vi "Omniax_MotorDrive_XYZR_SUPER.vi"() -> ()   [LabVIEW 2009]
uses:
  <vilib>/Utility/file.llb/Read From Spreadsheet File (DBL).vi
  <vilib>/Utility/file.llb/Read From Spreadsheet File (string).vi
  <vilib>/Instr/_visa.llb/VISA Configure Serial Port (Instr).vi
  <vilib>/Utility/file.llb/Write To Spreadsheet File (string).vi
  <vilib>/Utility/file.llb/Write To Spreadsheet File (DBL).vi
panel:
  out "OP":bool
  out "CL":bool
  out "Valve \nopend/closed":bool
  in  "OK Button":bool
  out "STATUS":string
  in  "Delete Button":bool
  in  "String":string
  in  "Add Button":bool
  in  "Set Button":bool
  in  "Preset positions":i32(ring) items=["ZERO", "Default", "CDOSE", "QMS", "test", "test2", "test3"]
  out "Presets":i32[][](array[numeric])
  out "X MINPOS":i32=-94296
  out "X MAXPOS":i32=-34296
  out "Y MINPOS":i32=-94296
  out "Y MAXPOS":i32=-34296
  out "R MAXPOS":i32=-34296
  out "R MINPOS":i32=-94296
  out "Z MINPOS":i32=-94296
  out "Z MAXPOS":i32=-34296
  in  "HARDSTOP":bool
  in  "GO":bool
  out "XYZR VEL PV Array":i32[](array[numeric])
  out "XYZ in RANGE Array":bool[](array[boolean])
  out "STEP SP Array":i32[](array[numeric])
  out "RUNHOLDArray":i32[](array[numeric])
  out "ZCONSTArray":dbl[](array[numeric])
  out "RCONSTArray":dbl[](array[numeric])
  out "XCONSTArray":dbl[](array[numeric])
  out "YCONSTArray":dbl[](array[numeric])
  out "Error Array":errorcluster[](array[cluster])
  out "COM PORT Array":refnum<visa-resource-name>[](array[refnum])
  out "Z COM PORT":refnum<visa-resource-name>="COM6"
  in  "Tab Control 3":enum32{"Status", "Reset"}(tab)
  out "Y in Range":bool
  out "Y Scan":bool
  out "Y in Motion":bool
  out "Y Backlash corr":bool
  out "X  in Range":bool
  out "X Scan":bool
  out "X  in Motion":bool
  out "X Backlash corr":bool
  out "Z in Range":bool
  out "Z Scan":bool
  out "Z in Motion":bool
  out "Z Backlash corr":bool
  out "R in Range":bool
  out "R Scan":bool
  out "R in Motion":bool
  out "R Backlash corr":bool
  out "X Ready":bool
  out "Y Ready":bool
  out "Z Ready":bool
  out "R Ready":bool
  in  "Reset Y Position mm":dbl
  out "Reset Y Motor Steps":i32
  in  "Reset X Position mm":dbl
  out "Reset X Motor Steps":i32
  in  "Reset Z Position mm":dbl
  out "Reset Z Motor Steps":i32
  in  "Reset R Position deg":dbl
  out "Reset R Motor Steps":i32
  in  "Reset":bool
  in  "Tab Control 2":enum32{"mm", "step"}(tab)
  in  "X Scan Length SP mm":dbl
  in  "X Scan Velocity SP mm/sec":dbl
  in  "Y Scan Length SP mm":dbl
  in  "Y Scan Velocity SP mm/sec":dbl
  in  "Set Scan \nParameters":bool
  in  "Z Scan Length SP mm":dbl
  in  "Z Scan Velocity SP mm/sec":dbl
  in  "R Scan Length SP deg":dbl
  in  "R Scan Velocity SP deg/sec":dbl
  in  "Z as dominating length":bool
  in  "X Scan Velocity SP steps/sec":i32=1 min=1 max=102400 step=1
  in  "X Scan Length SP steps":i32 min=-3507200 max=1100800 step=100
  out "X Scan length MV mm":dbl
  out "X Scan velocity MV mm/sec":dbl format="%#_6f"
  in  "Y Scan Velocity SP steps/sec":i32=1 min=1 max=102400 step=1
  in  "Y Scan Length SP steps":i32 min=-2562560 max=2045440 step=100
  out "Y Scan length MV mm":dbl
  out "Y Scan velocity MV mm/sec":dbl format="%#_6f"
  in  "Z Scan Velocity SP steps/sec":i32=1 min=1 max=102400 step=1
  in  "Z Scan Length SP steps":i32 min=-91443200 max=10956800 step=100
  out "Z Scan length MV mm":dbl
  out "Z Scan velocity MV mm/sec":dbl format="%#_6f"
  in  "R Scan Velocity SP steps/sec":i32=1 min=1 max=102400 step=1
  in  "R Scan Length SP steps":i32 min=-1501867 max=4642133 step=100
  out "R Scan length MV deg":dbl
  out "R Scan velocity MV deg/sec":dbl format="%#_6f"
  out "atan Y/Z":dbl
  in  "Tab Control":enum32{"mm", "step"}(tab)
  in  "X Position SP mm":dbl
  in  "X Velocity SP mm/sec":dbl
  in  "X Move Set":bool
  in  "Y Move Set":bool
  in  "Y Position SP mm":dbl
  in  "Y Velocity SP mm/sec":dbl
  in  "Z Position SP mm":dbl
  in  "Z Velocity SP mm/sec":dbl
  in  "Z Move Set":bool
  in  "R Position SP deg":dbl
  in  "R Velocity SP deg/sec":dbl
  in  "R Move Set":bool
  in  "X Velocity SP step/sec":i32 min=1 max=128000
  out "X Velocity MV mm/sec":dbl
  in  "Y Velocity SP step/sec":i32 min=1 max=128000
  out "Y Velocity MV mm/sec":dbl
  in  "Z Velocity SP step/sec":i32 min=1 max=204800
  out "Z Velocity MV mm/sec":dbl
  in  "R Velocity SP step/sec":i32 min=1 max=20000
  out "R Velocity MVdeg/sec":dbl
  in  "Y Step SP":i32=-20000 min=-2304000 max=2304000 step=500
  out "Y Position MV mm":dbl
  in  "X Step SP":i32=-20000 min=-2304000 max=2304000 step=500
  out "X Position MV mm":dbl
  in  "Z Step SP":i32=-20000 min=0 max=102400000 step=500
  out "Z Position MV mm":dbl
  in  "R Step SP":i32=-20000 min=-6144000 max=0 step=500
  out "R Position MV deg":dbl
  out "X Step PV":i32 max=2000
  out "Y Step PV":i32 max=2000
  out "Z Step PV":i32 max=2000
  out "R Step PV":i32 max=2000
  in  "Clear ZY":bool
  out "ZY Graph":cluster{dbl[], dbl[]}(graph)
  out "ZR Graph":cluster{"Y":dbl[], "Y":dbl[]}[](graph)
  out "XY Graph":cluster{"Y":dbl[], "Y":dbl[]}[](graph)
  out "X Scan Duration":dbl
  out "Y Scan Duration":dbl
  out "Z Scan Duration":dbl
  out "R Scan Duration":dbl
  out "R Backlash steps/sec":i32
  out "R Backlash":i32
  out "R Holding Current %":i32
  out "R Run Current %":i32
  out "R offset deg":dbl
  out "R deg/rev":dbl
  out "R steps/rev":u32
  out "R velocity PV step/sec":i32
  out "R COM PORT":refnum<visa-resource-name>="COM5"
  out "R Position deg PV":dbl
  out "Z Backlash steps/sec":i32
  out "Z Backlash":i32
  out "Z Holding Current %":i32
  out "Z Run Current %":i32
  out "Z offset mm":dbl
  out "Z mm/rev":dbl
  out "Z steps/rev":u32
  out "Z  velocity PV step/sec":i32
  out "Z Position mm PV":dbl
  out "X Position mm PV":dbl
  out "X velocity PV step/sec":i32
  in  "Set for Scan":bool
  out "X Backlash steps/sec":i32
  out "X Backlash":i32
  out "X Holding Current %":i32
  out "X Run Current %":i32
  out "X offset mm":dbl
  out "X mm/rev":dbl
  out "X steps/rev":u32
  out "X COM PORT":refnum<visa-resource-name>="COM5"
  out "Y Backlash steps/sec":i32
  out "Y Backlash":i32
  out "Y Holding Current %":i32
  out "Y Run Current %":i32
  in  "Scan Cancel":bool
  out "Y Position mm PV":dbl
  out "Y offset mm":dbl
  out "Y mm/rev":dbl
  out "Y steps/rev":u32
  out "Y velocity PV step/sec":i32
  in  "Scan Go":bool
  in  "Stop":bool
  out "Y COM PORT":refnum<visa-resource-name>="COM5"
  # "MX"
  # "MY"
  # "MZ"
  # "MR"
  # "Indicators"
  # "L"
  # "M"
  # "B"
  # "S"
  # "R"
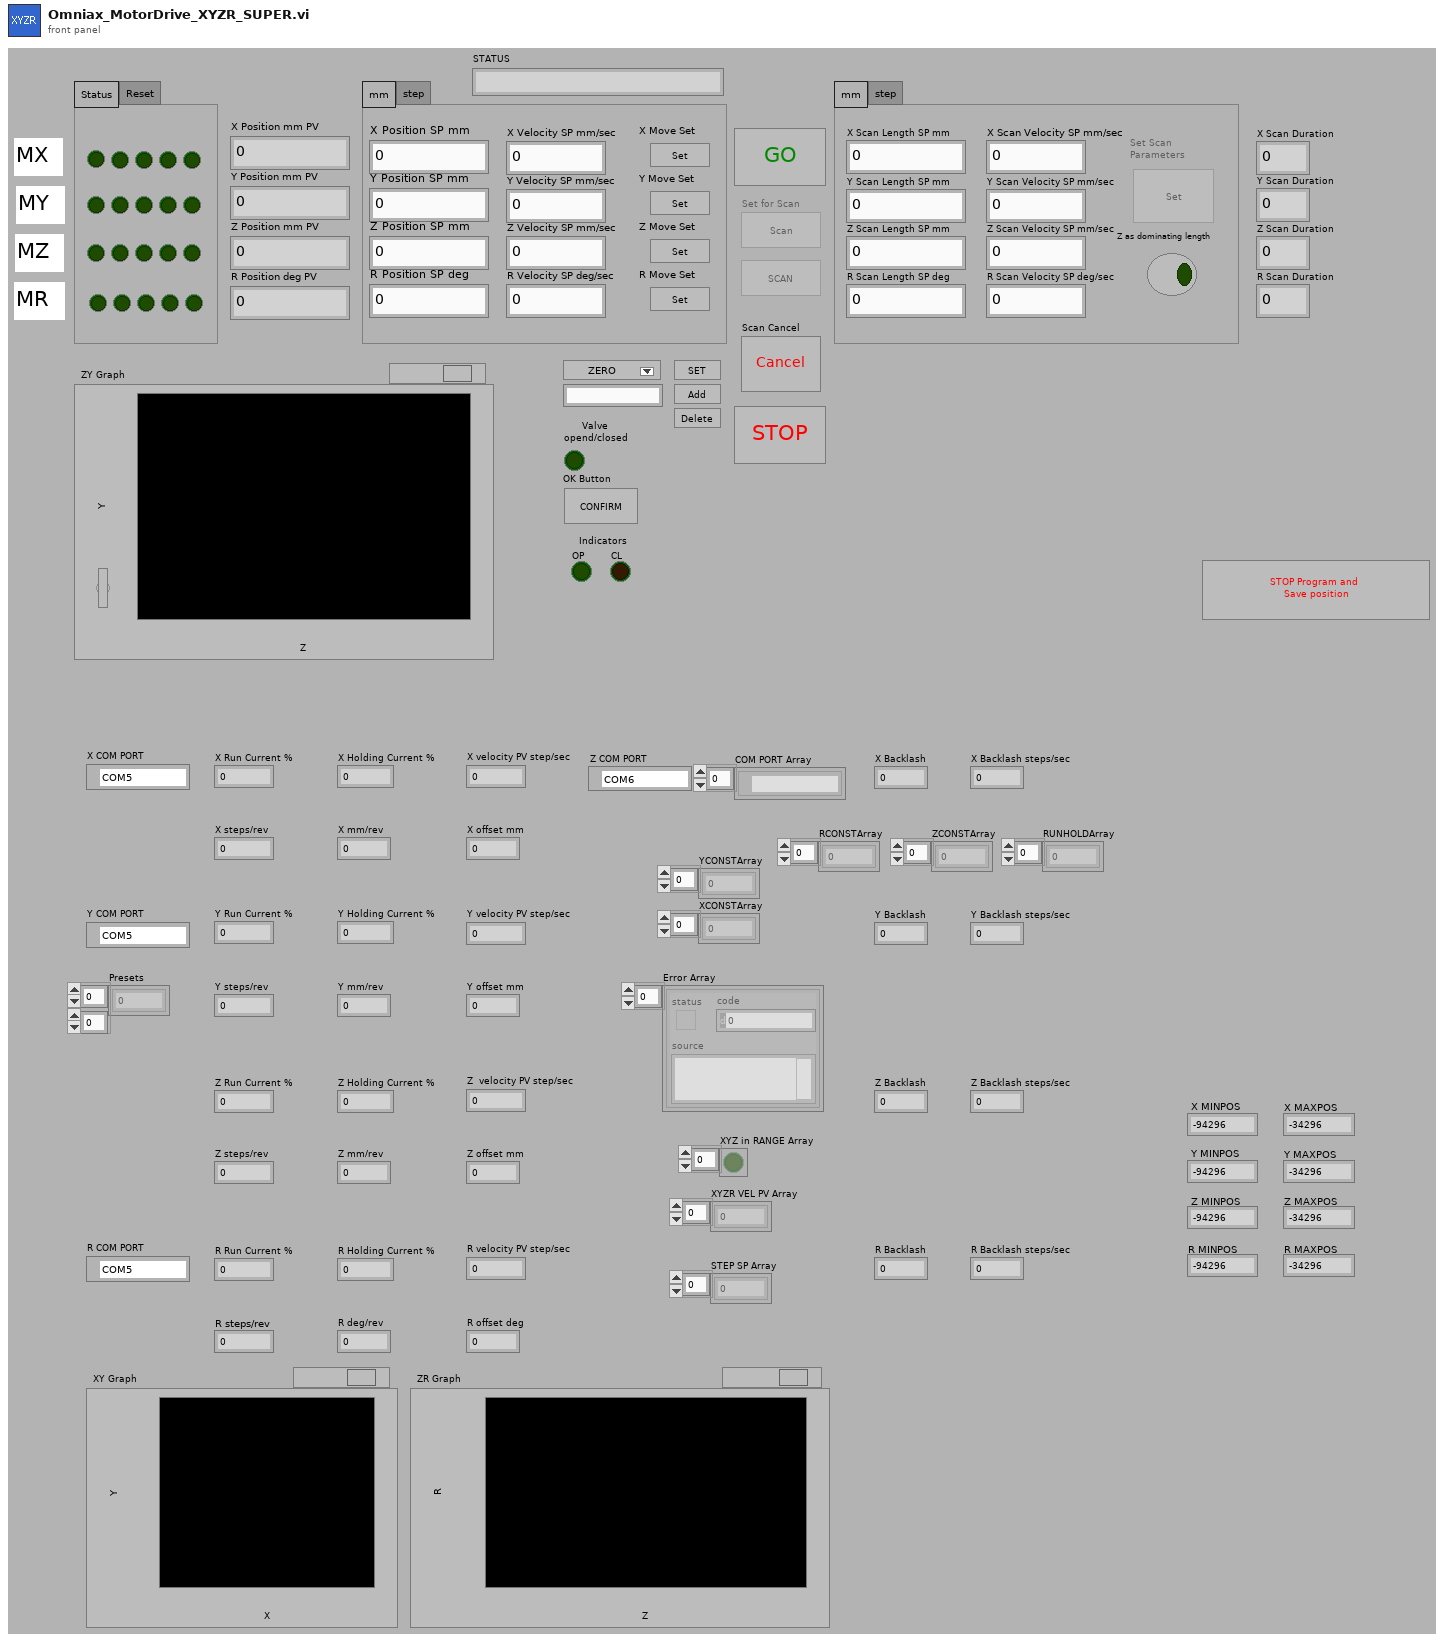
[diagram p1: front panel]
types:
  T1 = enum8{"Enabled", "Disabled", "Disabled and Grayed Out"}
  T2 = cluster{"[0]":i32, "[1]":i32, "[2]":i32, "[3]":i32, "[4]":i32, "[5]":i32, "[6]":i32, "[7]":i32, "[8]":i32}
  T3 = cluster{"XY Max Min array OUT[0]":dbl, "XY Max Min array OUT[1]":dbl, "XY Max Min array OUT[2]":dbl, "XY Max Min array OUT[3]":dbl, "XY Max Min array OUT[4]":dbl, "XY Max Min array OUT[5]":dbl, "XY Max Min array OUT[6]":dbl, "XY Max Min array OUT[7]":dbl, "XY Max Min array OUT[8]":dbl}
  T4 = cluster{"COM PORT Array OUT[0]":refnum<visa-resource-name>, "COM PORT Array OUT[1]":refnum<visa-resource-name>, "COM PORT Array OUT[2]":refnum<visa-resource-name>, "COM PORT Array OUT[3]":refnum<visa-resource-name>, "COM PORT Array OUT[4]":refnum<visa-resource-name>, "COM PORT Array OUT[5]":refnum<visa-resource-name>, "COM PORT Array OUT[6]":refnum<visa-resource-name>, "COM PORT Array OUT[7]":refnum<visa-resource-name>, "COM PORT Array OUT[8]":refnum<visa-resource-name>}
  T5 = cluster{"STEP SP Array OUT[0]":i32, "STEP SP Array OUT[1]":i32, "STEP SP Array OUT[2]":i32, "STEP SP Array OUT[3]":i32, "STEP SP Array OUT[4]":i32, "STEP SP Array OUT[5]":i32, "STEP SP Array OUT[6]":i32, "STEP SP Array OUT[7]":i32, "STEP SP Array OUT[8]":i32}
  T6 = cluster{"XYZ in RANGE Array OUT[0]":bool, "XYZ in RANGE Array OUT[1]":bool, "XYZ in RANGE Array OUT[2]":bool, "XYZ in RANGE Array OUT[3]":bool, "XYZ in RANGE Array OUT[4]":bool, "XYZ in RANGE Array OUT[5]":bool, "XYZ in RANGE Array OUT[6]":bool, "XYZ in RANGE Array OUT[7]":bool, "XYZ in RANGE Array OUT[8]":bool}
  T7 = cluster{"XYZR VEL PV Array OUT[0]":i32, "XYZR VEL PV Array OUT[1]":i32, "XYZR VEL PV Array OUT[2]":i32, "XYZR VEL PV Array OUT[3]":i32, "XYZR VEL PV Array OUT[4]":i32, "XYZR VEL PV Array OUT[5]":i32, "XYZR VEL PV Array OUT[6]":i32, "XYZR VEL PV Array OUT[7]":i32, "XYZR VEL PV Array OUT[8]":i32}
  T8 = cluster{"XYZR MAX MIN POS[0]":i32, "XYZR MAX MIN POS[1]":i32, "XYZR MAX MIN POS[2]":i32, "XYZR MAX MIN POS[3]":i32, "XYZR MAX MIN POS[4]":i32, "XYZR MAX MIN POS[5]":i32, "XYZR MAX MIN POS[6]":i32, "XYZR MAX MIN POS[7]":i32, "XYZR MAX MIN POS[8]":i32}
  T9 = cluster{"Error Array OUT[0]":errorcluster, "Error Array OUT[1]":errorcluster, "Error Array OUT[2]":errorcluster, "Error Array OUT[3]":errorcluster, "Error Array OUT[4]":errorcluster, "Error Array OUT[5]":errorcluster, "Error Array OUT[6]":errorcluster, "Error Array OUT[7]":errorcluster, "Error Array OUT[8]":errorcluster}
  T10 = enum16{"Stop", "Reset", "Run Current", "Holding Current", "Accel Rate", "Decel Rate", "Move to Relative Position", "Move to Absolute Position", "Echo Mode", "Print Parameter", "Send String", "Microstep Resolution", "Set Current Position", "Max Velocity"}
  T11 = cluster{"Presets[0]":i32, "Presets[1]":i32, "Presets[2]":i32, "Presets[3]":i32, "Presets[4]":i32, "Presets[5]":i32, "Presets[6]":i32, "Presets[7]":i32, "Presets[8]":i32}
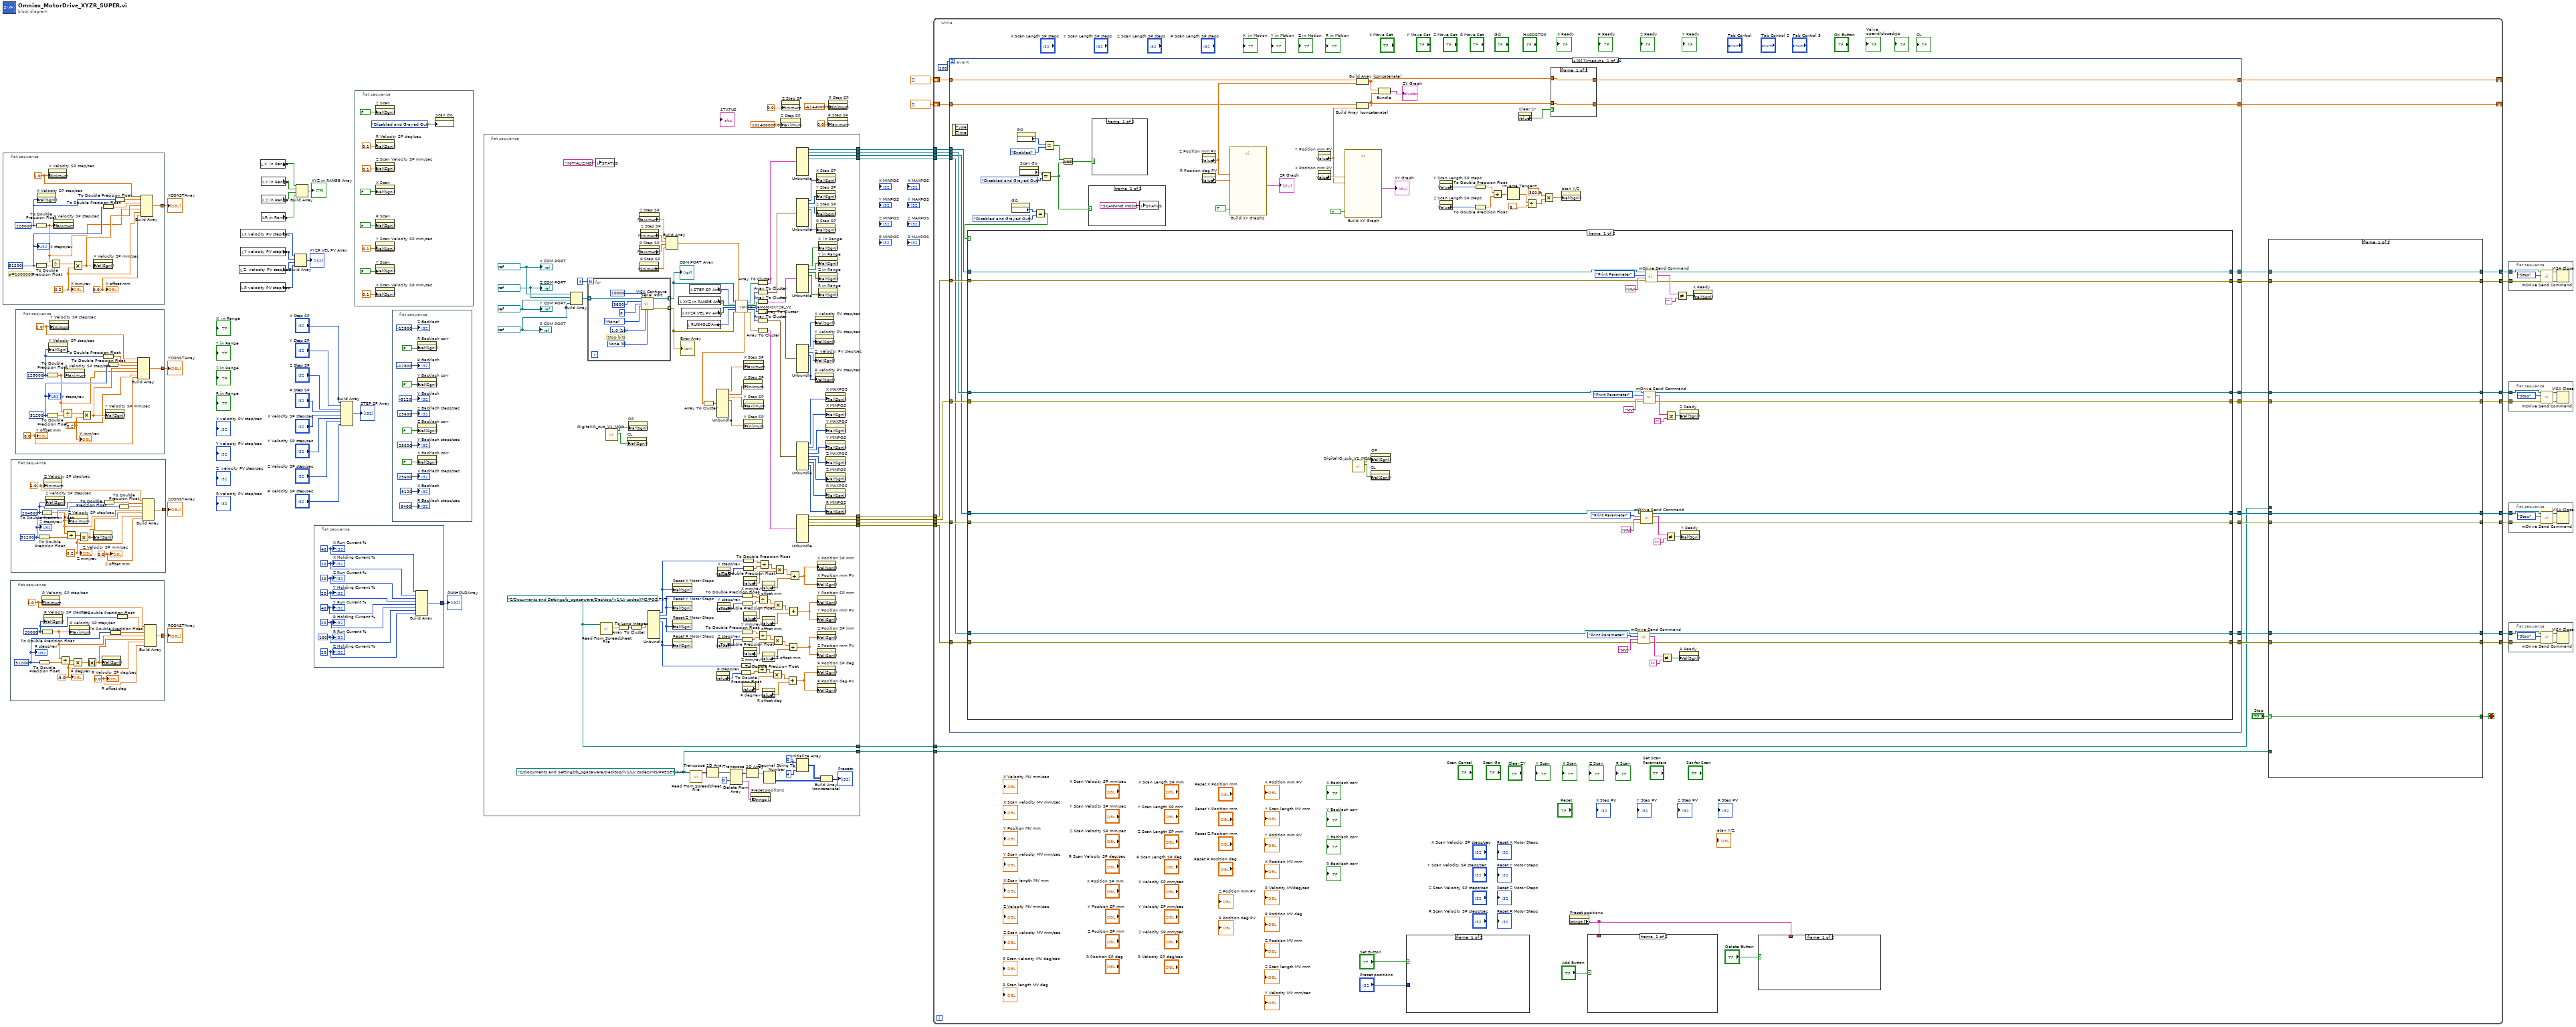
[diagram p0: block diagram]
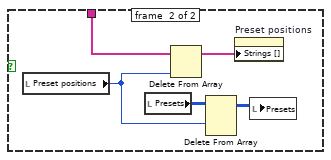
[diagram p2: hidden frame]
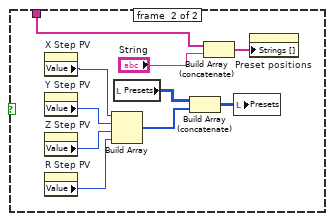
[diagram p3: hidden frame]
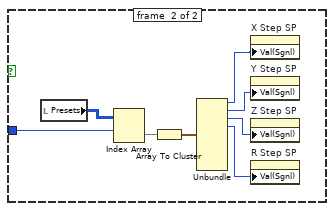
[diagram p4: hidden frame]
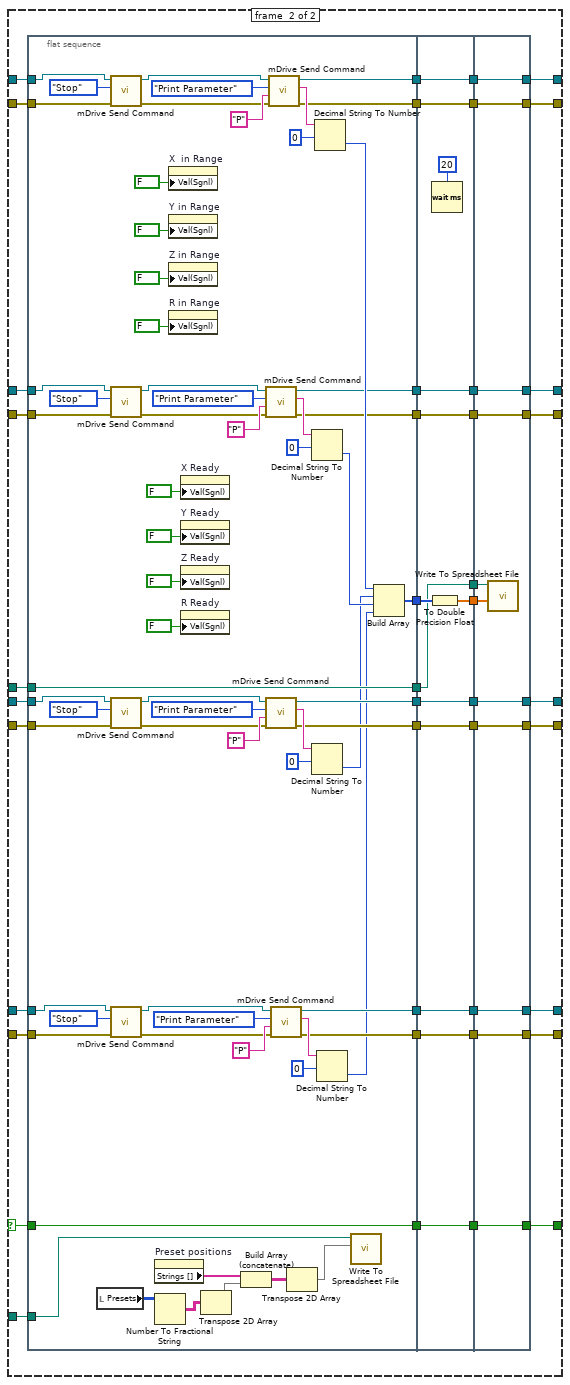
[diagram p5: hidden frame]
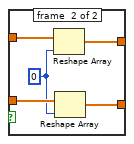
[diagram p6: hidden frame]
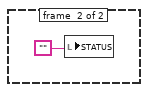
[diagram p8: hidden frame]
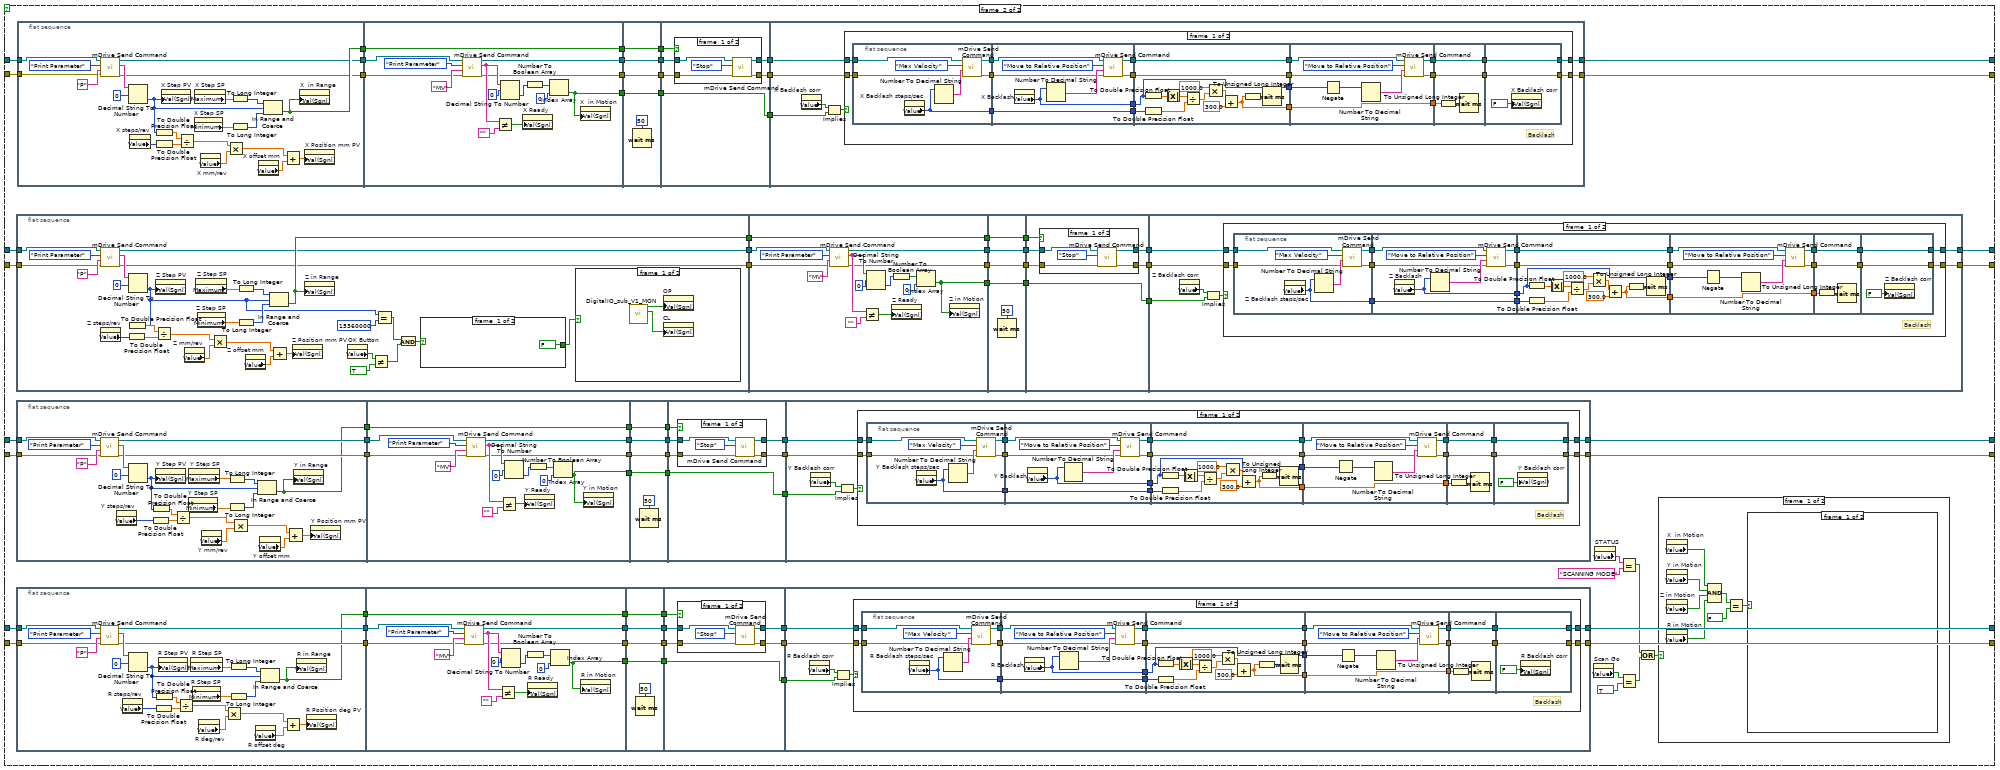
[diagram p9: hidden frame]
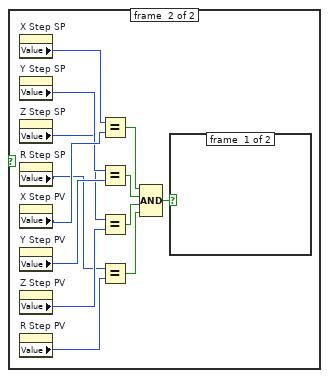
[diagram p10: hidden frame]
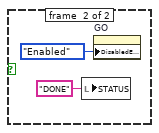
[diagram p11: hidden frame]
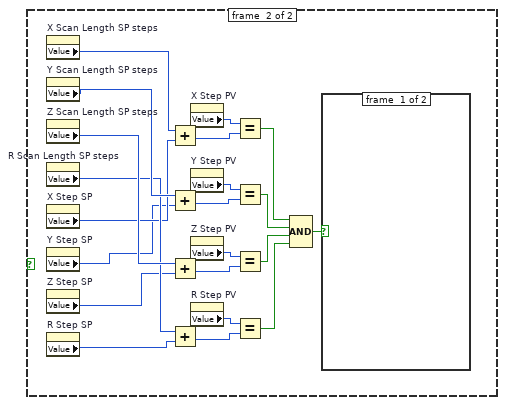
[diagram p12: hidden frame]
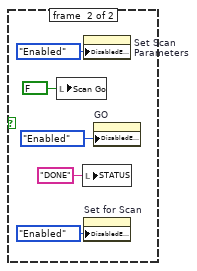
[diagram p13: hidden frame]
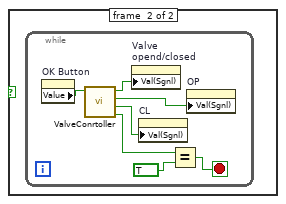
[diagram p18: hidden frame]
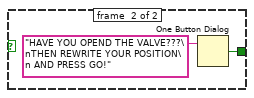
[diagram p19: hidden frame]
diagram:
  n1 = flat-sequence {
    tunnel: [w52] -> w35
    frame #0 {
      w50 = 0.2 ("MM/rev")
      w55 = u32 51200 ("step/rev")
      w57 = 128000 ("Value (Signaling)")
      w58 = 1.0 ("Data Entry Limits:Minimum")
      w51 = 0.0 ("offset")
      # "a=1000000"
      n2 = To Double Precision Float(number=w57) -> (double precision float=w49:dbl)
      n3 = To Double Precision Float(number=w55) -> (double precision float=w60:dbl)
      n4 = property on="X Velocity SP step/sec" class="DigNum (strict)"("Val(Sgnl)"=w57) -> ()  [unwired: 2 in, 2 out]
      n5 = property on="X Velocity SP step/sec" class="DigNum (strict)"("Minimum"=w58) -> ()  [unwired: 2 in, 2 out]
      n6 = Divide(x=w49, y=w60) -> (x/y=w59:dbl)
      n7 = property on="X Velocity SP step/sec" class="DigNum (strict)"("Maximum"=w49) -> ()  [unwired: 2 in, 2 out]
      n8 = Multiply(x=w59, y=w50) -> (x*y=w53:dbl)
      n9 = property on="X Velocity SP mm/sec" class="DigNum (strict)"("Val(Sgnl)"=w53) -> ()  [unwired: 2 in, 2 out]
      n10 = To Double Precision Float(number=w55) -> (double precision float=w54:dbl)
      n11 = To Double Precision Float(number=w57) -> (double precision float=w56:dbl)
      n12 = Build Array(w58, w56, w54, w53, w49, w50, w51) -> (w52:dbl[])
      "X offset mm" <- w51
      "X steps/rev" <- w55
      "X mm/rev" <- w50
    }
  }
  n13 = flat-sequence {
    tunnel: [w61] -> w34
    frame #0 {
      w70 = 1.0 ("Data Entry Limits:Minimum")
      w64 = 0.0 ("R offset deg")
      w65 = -3.0 ("R deg/rev")
      w68 = u32 51200 ("step/rev")
      w69 = 20000 ("Value (Signaling)")
      n14 = To Double Precision Float(number=w68) -> (double precision float=w71:dbl)
      n15 = To Double Precision Float(number=w69) -> (double precision float=w67:dbl)
      n16 = property on="R Velocity SP step/sec" class="DigNum (strict)"("Minimum"=w70) -> ()  [unwired: 2 in, 2 out]
      n17 = property on="R Velocity SP step/sec" class="DigNum (strict)"("Val(Sgnl)"=w69) -> ()  [unwired: 2 in, 2 out]
      n18 = Divide(x=w67, y=w71) -> (x/y=w73:dbl)
      n19 = property on="R Velocity SP step/sec" class="DigNum (strict)"("Maximum"=w67) -> ()  [unwired: 2 in, 2 out]
      n20 = Multiply(x=w73, y=w65) -> (x*y=w72:dbl)
      n21 = Absolute Value(x=w72) -> (abs(x)=w66:dbl)
      n22 = property on="R Velocity SP deg/sec" class="DigNum (strict)"("Val(Sgnl)"=w66) -> ()  [unwired: 2 in, 2 out]
      n23 = To Double Precision Float(number=w68) -> (double precision float=w62:dbl)
      n24 = To Double Precision Float(number=w69) -> (double precision float=w63:dbl)
      n25 = Build Array(w70, w63, w62, w67, w66, w65, w64) -> (w61:dbl[])
      "R offset deg" <- w64
      "R deg/rev" <- w65
      "R steps/rev" <- w68
    }
  }
  n26 = flat-sequence {
    tunnel: [w74] -> w33
    frame #0 {
      w76 = 0.2 ("Z mm/rev")
      w80 = u32 51200 ("step/rev")
      w82 = 204800 ("Value (Signaling)")
      w83 = 1.0 ("Data Entry Limits:Minimum")
      w75 = 0.0 ("Z offset mm")
      n27 = To Double Precision Float(number=w80) -> (double precision float=w85:dbl)
      n28 = To Double Precision Float(number=w82) -> (double precision float=w78:dbl)
      n29 = property on="Z Velocity SP step/sec" class="DigNum (strict)"("Minimum"=w83) -> ()  [unwired: 2 in, 2 out]
      n30 = property on="Z Velocity SP step/sec" class="DigNum (strict)"("Val(Sgnl)"=w82) -> ()  [unwired: 2 in, 2 out]
      n31 = Divide(x=w78, y=w85) -> (x/y=w84:dbl)
      n32 = property on="Z Velocity SP step/sec" class="DigNum (strict)"("Maximum"=w78) -> ()  [unwired: 2 in, 2 out]
      n33 = Multiply(x=w84, y=w76) -> (x*y=w77:dbl)
      n34 = property on="Z Velocity SP mm/sec" class="DigNum (strict)"("Val(Sgnl)"=w77) -> ()  [unwired: 2 in, 2 out]
      n35 = To Double Precision Float(number=w82) -> (double precision float=w81:dbl)
      n36 = To Double Precision Float(number=w80) -> (double precision float=w79:dbl)
      n37 = Build Array(w83, w81, w79, w78, w77, w76, w75) -> (w74:dbl[])
      "Z offset mm" <- w75
      "Z mm/rev" <- w76
      "Z steps/rev" <- w80
    }
  }
  n38 = flat-sequence {
    tunnel: [w89] -> w36
    frame #0 {
      w87 = 0.2 ("MM/rev")
      w92 = u32 51200 ("step/rev")
      w94 = 128000 ("Value (Signaling)")
      w95 = 1.0 ("Data Entry Limits:Minimum")
      w88 = 0.0 ("offset")
      n39 = To Double Precision Float(number=w94) -> (double precision float=w86:dbl)
      n40 = To Double Precision Float(number=w92) -> (double precision float=w97:dbl)
      n41 = property on="Y Velocity SP step/sec" class="DigNum (strict)"("Val(Sgnl)"=w94) -> ()  [unwired: 2 in, 2 out]
      n42 = property on="Y Velocity SP step/sec" class="DigNum (strict)"("Minimum"=w95) -> ()  [unwired: 2 in, 2 out]
      n43 = Divide(x=w86, y=w97) -> (x/y=w96:dbl)
      n44 = property on="Y Velocity SP step/sec" class="DigNum (strict)"("Maximum"=w86) -> ()  [unwired: 2 in, 2 out]
      n45 = Multiply(x=w96, y=w87) -> (x*y=w90:dbl)
      n46 = To Double Precision Float(number=w94) -> (double precision float=w93:dbl)
      n47 = property on="Y Velocity SP mm/sec" class="DigNum (strict)"("Val(Sgnl)"=w90) -> ()  [unwired: 2 in, 2 out]
      n48 = To Double Precision Float(number=w92) -> (double precision float=w91:dbl)
      n49 = Build Array(w95, w93, w91, w90, w86, w87, w88) -> (w89:dbl[])
      "Y offset mm" <- w88
      "Y steps/rev" <- w92
      "Y mm/rev" <- w87
    }
  }
  n50 = local read "Z  velocity PV step/sec"() -> (w16:i32)
  n51 = local read "R velocity PV step/sec"() -> (w18:i32)
  n52 = local read "X velocity PV step/sec"() -> (w19:i32)
  n53 = local read "Y velocity PV step/sec"() -> (w17:i32)
  n54 = local read "X  in Range"() -> (w23:bool)
  n55 = local read "R in Range"() -> (w20:bool)
  n56 = local read "Y in Range"() -> (w22:bool)
  n57 = local read "Z in Range"() -> (w21:bool)
  n58 = Build Array(w19, w17, w16, w18) -> (→"XYZR VEL PV Array":i32[])
  n59 = Build Array(w23, w22, w21, w20) -> (→"XYZ in RANGE Array":bool[])
  n60 = flat-sequence {
    tunnel: [w98] -> w32
    frame #0 {
      w101 = 20 ("R Holding Current %")
      w100 = 100 ("R Run Current %")
      w103 = 20 ("Holding Current %")
      w102 = 40 ("Run Current %")
      w105 = 20 ("Holding Current %")
      w106 = 40 ("Run Current %")
      w104 = 40 ("Z Run Current %")
      w99 = 20 ("Z Holding Current %")
      n61 = Build Array(w106, w105, w104, w103, w102, w101, w100, w99) -> (w98:i32[])
      "Z Holding Current %" <- w99
      "Z Run Current %" <- w104
      "X Run Current %" <- w106
      "X Holding Current %" <- w105
      "Y Run Current %" <- w102
      "Y Holding Current %" <- w103
      "R Holding Current %" <- w101
      "R Run Current %" <- w100
    }
  }
  n62 = Build Array("X Step SP", "Y Step SP", "Z Step SP", "R Step SP", "X Velocity SP step/sec", "Y Velocity SP step/sec", "Z Velocity SP step/sec", "R Velocity SP step/sec") -> (→"STEP SP Array":i32[])
  n63 = flat-sequence {
    frame #0 {
      n64 = property on="Z Scan" class="Bool (strict)"("Val(Sgnl)"=FALSE ("Value (Signaling)")) -> ()  [unwired: 2 in, 2 out]
      n65 = property on="R Velocity SP deg/sec" class="DigNum (strict)"("Val(Sgnl)"=0.1 ("Value (Signaling)")) -> ()  [unwired: 2 in, 2 out]
      n66 = property on="Z Scan Velocity SP mm/sec" class="DigNum (strict)"("Val(Sgnl)"=0.1 ("Value (Signaling)")) -> ()  [unwired: 2 in, 2 out]
      n67 = property on="X Scan" class="Bool (strict)"("Val(Sgnl)"=FALSE ("Value (Signaling)")) -> ()  [unwired: 2 in, 2 out]
      n68 = property on="R Scan" class="Bool (strict)"("Val(Sgnl)"=FALSE ("Value (Signaling)")) -> ()  [unwired: 2 in, 2 out]
      n69 = property on="Y Scan Velocity SP mm/sec" class="DigNum (strict)"("Val(Sgnl)"=0.1 ("Value (Signaling)")) -> ()  [unwired: 2 in, 2 out]
      n70 = property on="Y Scan" class="Bool (strict)"("Val(Sgnl)"=FALSE ("Value (Signaling)")) -> ()  [unwired: 2 in, 2 out]
      n71 = property on="X Scan Velocity SP mm/sec" class="DigNum (strict)"("Val(Sgnl)"=0.1 ("Value (Signaling)")) -> ()  [unwired: 2 in, 2 out]
      n72 = property on="Scan Go" class="Bool (strict)"("DisabledEnum"=T1."Disabled and Grayed Out" ("Disabled")) -> ()  [unwired: 2 in, 2 out]
    }
  }
  n73 = flat-sequence {
    frame #0 {
      n74 = property on="R Backlash corr" class="Bool (strict)"("Val(Sgnl)"=FALSE ("Value (Signaling)")) -> ()  [unwired: 2 in, 2 out]
      n75 = property on="Y Backlash corr" class="Bool (strict)"("Val(Sgnl)"=FALSE ("Value (Signaling)")) -> ()  [unwired: 2 in, 2 out]
      n76 = property on="Z Backlash corr" class="Bool (strict)"("Val(Sgnl)"=FALSE ("Value (Signaling)")) -> ()  [unwired: 2 in, 2 out]
      n77 = property on="X Backlash corr" class="Bool (strict)"("Val(Sgnl)"=FALSE ("Value (Signaling)")) -> ()  [unwired: 2 in, 2 out]
      "Z Backlash steps/sec" <- 25600 ("Z Backlash steps/sec")
      "Z Backlash" <- -12800 ("Z Backlash")
      "X Backlash steps/sec" <- 25600 ("Value (Signaling)")
      "X Backlash" <- 5120 ("Backlash2")
      "Y Backlash" <- -5120 ("Backlash2")
      "Y Backlash steps/sec" <- 25600 ("Value (Signaling)")
      "R Backlash steps/sec" <- 6400 ("R Backlash steps/sec")
      "R Backlash" <- -12800 ("R Backlash")
    }
  }
  n78 = flat-sequence {
    tunnel: [w222] -> w12
    tunnel: [w221] -> w11
    tunnel: [w220] -> w10
    tunnel: [w219] -> w9
    tunnel: [w218] -> w8
    tunnel: [w217] -> w7
    tunnel: [w216] -> w6
    tunnel: [w215] -> w5
    tunnel: [w212] -> w4
    tunnel: [w182] -> w3
    frame #0 {
      w182 = path "C:/Documents and Settings/b_ogasawara/Desktop/lv1/LV codes/IMS/PRESET.TXT"
      w180 = 0 ("element")
      w212 = path "C:/Documents and Settings/b_ogasawara/Desktop/lv1/LV codes/IMS/POS.TXT"
      w242 = refnum<visa-resource-name> "COM7" ("COM PORT")
      w243 = refnum<visa-resource-name> "COM5" ("COM PORT")
      w244 = refnum<visa-resource-name> "COM6" ("VISA resource name")
      w245 = refnum<visa-resource-name> "COM4" ("COM PORT")
      n79 = Build Array(w245, w244, w243, w242) -> (w240:refnum<visa-resource-name>[])
      n80 = for {
        N: 4 -> [_]
        tunnel: w240 -> [w248] mode=indexing
        tunnel: [w247] -> w238 mode=indexing
        tunnel: [w246] -> w239 mode=indexing
        w250 = u16 0 items=["None", "XON/XOFF", "RTS/CTS", "XON/XOFF & RTS/CTS", "DTR/DSR", "XON/XOFF & DTR/DSR"] ("flow control (0:none)")
        w251 = u16 10 items=["1.0"=10, "1.5"=15, "2.0"=20] ("stop bits (10: 1 bit)")
        # "Stop bits"
        n81 = call-poly "VISA Configure Serial Port"("VISA resource name"=w248, "timeout (10sec)"=u32 10000, "baud rate (9600)"=u32 9600, "data bits (8)"=u16 8, "parity (0:none)"=enum16{"None", "Odd", "Even", "Mark", "Space"}."None", "stop bits (10: 1 bit)"=w251, "flow control (0:none)"=w250) -> ("VISA resource name out"=w247:refnum<visa-resource-name>, "error out"=w246:errorcluster)  [unwired: 7 in]
      }
      "COM PORT Array" <- w238
      "Error Array" <- w239
      n82 = local write "STATUS"("INITIALIZING" ("STATUS")) -> ()
      n83 = call-poly <vilib>:"Read From Spreadsheet File.vi"("file path (dialog if empty)"=w212) -> ("first row"=w213:dbl[])  [unwired: 6 in, 4 out]
      n84 = call "DigitalIO_sub_V1_MON.vi"() -> ("CL"=w139:bool, "OP"=w140:bool)  [unwired: 8 in]
      n85 = To Long Integer(number=w213) -> (32bit integer=w179:i32[])
      n86 = property on="CL" class="Bool (strict)"("Val(Sgnl)"=w139) -> ()  [unwired: 2 in, 2 out]
      n87 = property on="OP" class="Bool (strict)"("Val(Sgnl)"=w140) -> ()  [unwired: 2 in, 2 out]
      n88 = Array To Cluster(array=w179) -> (cluster=w178:T2)
      n89 = property on="Z Step SP" class="DigNum (strict)"() -> ("Maximum"=w137:dbl)  [unwired: 2 in, 2 out]
      n90 = property on="R Step SP" class="DigNum (strict)"() -> ("Maximum"=w135:dbl)  [unwired: 2 in, 2 out]
      n91 = property on="R Step SP" class="DigNum (strict)"() -> ("Minimum"=w136:dbl)  [unwired: 2 in, 2 out]
      n92 = property on="Z Step SP" class="DigNum (strict)"() -> ("Minimum"=w138:dbl)  [unwired: 2 in, 2 out]
      n93 = Unbundle(w178) -> ("[0]"=w154:i32, "[1]"=w155:i32, "[2]"=w156:i32, "[3]"=w157:i32)  [unwired: 5 out]
      n94 = Build Array(w137, w138, w135, w136) -> (w134:dbl[])
      n95 = property on="Reset X Motor Steps" class="DigNum (strict)"("Val(Sgnl)"=w154) -> ()  [unwired: 2 in, 2 out]
      n96 = property on="Reset Y Motor Steps" class="DigNum (strict)"("Val(Sgnl)"=w155) -> ()  [unwired: 2 in, 2 out]
      n97 = property on="Reset Z Motor Steps" class="DigNum (strict)"("Val(Sgnl)"=w156) -> ()  [unwired: 2 in, 2 out]
      n98 = property on="Reset R Motor Steps" class="DigNum (strict)"("Val(Sgnl)"=w157) -> ()  [unwired: 2 in, 2 out]
      n99 = local read "XYZ in RANGE Array"() -> (w234:bool[])
      n100 = local read "XYZR VEL PV Array"() -> (w233:i32[])
      n101 = local read "RUNHOLDArray"() -> (w232:i32[])
      n102 = local read "STEP SP Array"() -> (w235:i32[])
      n103 = call-poly <vilib>:"Read From Spreadsheet File.vi"("file path (dialog if empty)"=w182) -> ("all rows"=w187:string[][])  [unwired: 6 in, 4 out]
      n104 = Transpose 2D Array(2D array=w187) -> (transposed array=w186:string[][])
      n105 = property on="R steps/rev" class="DigNum (strict)"() -> ("Value"=w150:u32)  [unwired: 2 in, 2 out]
      n106 = property on="X steps/rev" class="DigNum (strict)"() -> ("Value"=w153:u32)  [unwired: 2 in, 2 out]
      n107 = property on="Y steps/rev" class="DigNum (strict)"() -> ("Value"=w152:u32)  [unwired: 2 in, 2 out]
      n108 = property on="Z steps/rev" class="DigNum (strict)"() -> ("Value"=w151:u32)  [unwired: 2 in, 2 out]
      n109 = Delete From Array(array=w186, index (row)=0) -> (deleted portion=w181:string[], array with subset deleted=w184:string[][])  [unwired: 2 in]
      n110 = call "InitializeMotorsXYZR_V2.vi"("COM PORT Array IN"=w238, "STEP SP Array IN"=w235, "XYZ in RANGE Array IN"=w234, "XYZR VEL PV Array IN"=w233, "RUNHOLDArray IN"=w232, "Error Array IN"=w239, "ZR Max Min array"=w134) -> ("XY Max Min array OUT"=w133:dbl[], "COM PORT Array OUT"=w237:refnum<visa-resource-name>[], "STEP SP Array OUT"=w231:i32[], "XYZ in RANGE Array OUT"=w230:bool[], "XYZR VEL PV Array OUT"=w229:i32[], "XYZR MAX MIN POS"=w214:i32[], "Error Array OUT"=w236:errorcluster[])  [unwired: 6 in]
      n111 = Array To Cluster(array=w133) -> (cluster=w132:T3)
      n112 = Unbundle(w132) -> ("XY Max Min array OUT[0]"=w131:dbl, "XY Max Min array OUT[1]"=w129:dbl, "XY Max Min array OUT[2]"=w128:dbl, "XY Max Min array OUT[3]"=w130:dbl)  [unwired: 5 out]
      n113 = To Double Precision Float(number=w157) -> (double precision float=w163:dbl)
      n114 = To Double Precision Float(number=w150) -> (double precision float=w162:dbl)
      n115 = To Double Precision Float(number=w156) -> (double precision float=w167:dbl)
      n116 = To Double Precision Float(number=w151) -> (double precision float=w166:dbl)
      n117 = To Double Precision Float(number=w155) -> (double precision float=w171:dbl)
      n118 = To Double Precision Float(number=w152) -> (double precision float=w170:dbl)
      n119 = To Double Precision Float(number=w154) -> (double precision float=w175:dbl)
      n120 = To Double Precision Float(number=w153) -> (double precision float=w174:dbl)
      n121 = property on="R deg/rev" class="DigNum (strict)"() -> ("Value"=w146:dbl)  [unwired: 2 in, 2 out]
      n122 = property on="X Step SP" class="DigNum (strict)"("Maximum"=w131) -> ()  [unwired: 2 in, 2 out]
      n123 = property on="X Step SP" class="DigNum (strict)"("Minimum"=w129) -> ()  [unwired: 2 in, 2 out]
      n124 = property on="Y Step SP" class="DigNum (strict)"("Maximum"=w128) -> ()  [unwired: 2 in, 2 out]
      n125 = property on="Y Step SP" class="DigNum (strict)"("Minimum"=w130) -> ()  [unwired: 2 in, 2 out]
      n126 = property on="X mm/rev" class="DigNum (strict)"() -> ("Value"=w147:dbl)  [unwired: 2 in, 2 out]
      n127 = property on="Y mm/rev" class="DigNum (strict)"() -> ("Value"=w148:dbl)  [unwired: 2 in, 2 out]
      n128 = property on="Z mm/rev" class="DigNum (strict)"() -> ("Value"=w149:dbl)  [unwired: 2 in, 2 out]
      n129 = Transpose 2D Array(2D array=w184) -> (transposed array=w183:string[][])
      n130 = property on="Preset positions" class="Ring (strict)"("Strings []"=w181) -> ()  [unwired: 2 in, 2 out]
      n131 = Divide(x=w163, y=w162) -> (x/y=w165:dbl)
      n132 = Array To Cluster(array=w237) -> (cluster=w228:T4)
      n133 = Array To Cluster(array=w231) -> (cluster=w226:T5)
      n134 = Array To Cluster(array=w230) -> (cluster=w225:T6)
      n135 = Array To Cluster(array=w229) -> (cluster=w224:T7)
      n136 = Array To Cluster(array=w214) -> (cluster=w223:T8)
      n137 = Array To Cluster(array=w236) -> (cluster=w227:T9)
      n138 = Divide(x=w167, y=w166) -> (x/y=w169:dbl)
      n139 = Divide(x=w171, y=w170) -> (x/y=w173:dbl)
      n140 = Divide(x=w175, y=w174) -> (x/y=w177:dbl)
      n141 = property on="X offset mm" class="DigNum (strict)"() -> ("Value"=w142:dbl)  [unwired: 2 in, 2 out]
      n142 = property on="Y offset mm" class="DigNum (strict)"() -> ("Value"=w143:dbl)  [unwired: 2 in, 2 out]
      n143 = property on="Z offset mm" class="DigNum (strict)"() -> ("Value"=w144:dbl)  [unwired: 2 in, 2 out]
      n144 = property on="R offset deg" class="DigNum (strict)"() -> ("Value"=w145:dbl)  [unwired: 2 in, 2 out]
      n145 = Decimal String To Number(string=w183) -> (number=w185:i32[][])  [unwired: 2 in, 1 out]
      n146 = Multiply(x=w165, y=w146) -> (x*y=w164:dbl)
      n147 = Multiply(x=w169, y=w149) -> (x*y=w168:dbl)
      n148 = Multiply(x=w173, y=w148) -> (x*y=w172:dbl)
      n149 = Multiply(x=w177, y=w147) -> (x*y=w176:dbl)
      n150 = Add(x=w164, y=w145) -> (x+y=w161:dbl)
      n151 = Add(x=w168, y=w144) -> (x+y=w160:dbl)
      n152 = Add(x=w172, y=w143) -> (x+y=w159:dbl)
      n153 = Add(x=w176, y=w142) -> (x+y=w158:dbl)
      n154 = Unbundle(w228) -> ("COM PORT Array OUT[0]"=w222:refnum<visa-resource-name>, "COM PORT Array OUT[1]"=w221:refnum<visa-resource-name>, "COM PORT Array OUT[2]"=w220:refnum<visa-resource-name>, "COM PORT Array OUT[3]"=w219:refnum<visa-resource-name>)  [unwired: 5 out]
      n155 = Unbundle(w226) -> ("STEP SP Array OUT[0]"=w196:i32, "STEP SP Array OUT[1]"=w197:i32, "STEP SP Array OUT[2]"=w198:i32, "STEP SP Array OUT[3]"=w199:i32)  [unwired: 5 out]
      n156 = Unbundle(w225) -> ("XYZ in RANGE Array OUT[0]"=w211:bool, "XYZ in RANGE Array OUT[1]"=w210:bool, "XYZ in RANGE Array OUT[2]"=w209:bool, "XYZ in RANGE Array OUT[3]"=w208:bool)  [unwired: 5 out]
      n157 = Unbundle(w224) -> ("XYZR VEL PV Array OUT[0]"=w195:i32, "XYZR VEL PV Array OUT[1]"=w194:i32, "XYZR VEL PV Array OUT[2]"=w193:i32, "XYZR VEL PV Array OUT[3]"=w192:i32)  [unwired: 5 out]
      n158 = Unbundle(w223) -> ("XYZR MAX MIN POS[0]"=w207:i32, "XYZR MAX MIN POS[1]"=w206:i32, "XYZR MAX MIN POS[2]"=w205:i32, "XYZR MAX MIN POS[3]"=w204:i32, "XYZR MAX MIN POS[4]"=w203:i32, "XYZR MAX MIN POS[5]"=w202:i32, "XYZR MAX MIN POS[6]"=w201:i32, "XYZR MAX MIN POS[7]"=w200:i32)  [unwired: 1 out]
      n159 = Unbundle(w227) -> ("Error Array OUT[0]"=w218:errorcluster, "Error Array OUT[1]"=w217:errorcluster, "Error Array OUT[2]"=w216:errorcluster, "Error Array OUT[3]"=w215:errorcluster)  [unwired: 5 out]
      n160 = Initialize Array(w180, w180, 4 ("dimension size")) -> (w190:i32[][])
      n161 = property on="X velocity PV step/sec" class="DigNum (strict)"("Val(Sgnl)"=w195) -> ()  [unwired: 2 in, 2 out]
      n162 = property on="Y velocity PV step/sec" class="DigNum (strict)"("Val(Sgnl)"=w194) -> ()  [unwired: 2 in, 2 out]
      n163 = property on="Z  velocity PV step/sec" class="DigNum (strict)"("Val(Sgnl)"=w193) -> ()  [unwired: 2 in, 2 out]
      n164 = property on="R velocity PV step/sec" class="DigNum (strict)"("Val(Sgnl)"=w192) -> ()  [unwired: 2 in, 2 out]
      n165 = property on="X Step SP" class="DigNum (strict)"("Val(Sgnl)"=w196) -> ()  [unwired: 2 in, 2 out]
      n166 = property on="Y Step SP" class="DigNum (strict)"("Val(Sgnl)"=w197) -> ()  [unwired: 2 in, 2 out]
      n167 = property on="Z Step SP" class="DigNum (strict)"("Val(Sgnl)"=w198) -> ()  [unwired: 2 in, 2 out]
      n168 = property on="R Step SP" class="DigNum (strict)"("Val(Sgnl)"=w199) -> ()  [unwired: 2 in, 2 out]
      n169 = property on="X Position SP mm" class="DigNum (strict)"("Val(Sgnl)"=w158) -> ()  [unwired: 2 in, 2 out]
      n170 = property on="X Position mm PV" class="DigNum (strict)"("Val(Sgnl)"=w158) -> ()  [unwired: 2 in, 2 out]
      n171 = property on="Y Position SP mm" class="DigNum (strict)"("Val(Sgnl)"=w159) -> ()  [unwired: 2 in, 2 out]
      n172 = property on="Y Position mm PV" class="DigNum (strict)"("Val(Sgnl)"=w159) -> ()  [unwired: 2 in, 2 out]
      n173 = property on="Z Position SP mm" class="DigNum (strict)"("Val(Sgnl)"=w160) -> ()  [unwired: 2 in, 2 out]
      n174 = property on="Z Position mm PV" class="DigNum (strict)"("Val(Sgnl)"=w160) -> ()  [unwired: 2 in, 2 out]
      n175 = property on="R Position SP deg" class="DigNum (strict)"("Val(Sgnl)"=w161) -> ()  [unwired: 2 in, 2 out]
      n176 = property on="R Position deg PV" class="DigNum (strict)"("Val(Sgnl)"=w161) -> ()  [unwired: 2 in, 2 out]
      n177 = property on="X  in Range" class="Bool (strict)"("Val(Sgnl)"=w211) -> ()  [unwired: 2 in, 2 out]
      n178 = property on="Y in Range" class="Bool (strict)"("Val(Sgnl)"=w210) -> ()  [unwired: 2 in, 2 out]
      n179 = property on="Z in Range" class="Bool (strict)"("Val(Sgnl)"=w209) -> ()  [unwired: 2 in, 2 out]
      n180 = property on="R in Range" class="Bool (strict)"("Val(Sgnl)"=w208) -> ()  [unwired: 2 in, 2 out]
      n181 = Build Array (concatenate)(w190, w185) -> (→"Presets":i32[][])
      n182 = property on="X MAXPOS" class="DigNum (strict)"("Val(Sgnl)"=w207) -> ()  [unwired: 2 in, 2 out]
      n183 = property on="X MINPOS" class="DigNum (strict)"("Val(Sgnl)"=w206) -> ()  [unwired: 2 in, 2 out]
      n184 = property on="Y MAXPOS" class="DigNum (strict)"("Val(Sgnl)"=w205) -> ()  [unwired: 2 in, 2 out]
      n185 = property on="Y MINPOS" class="DigNum (strict)"("Val(Sgnl)"=w204) -> ()  [unwired: 2 in, 2 out]
      n186 = property on="Z MAXPOS" class="DigNum (strict)"("Val(Sgnl)"=w203) -> ()  [unwired: 2 in, 2 out]
      n187 = property on="Z MINPOS" class="DigNum (strict)"("Val(Sgnl)"=w202) -> ()  [unwired: 2 in, 2 out]
      n188 = property on="R MAXPOS" class="DigNum (strict)"("Val(Sgnl)"=w201) -> ()  [unwired: 2 in, 2 out]
      n189 = property on="R MINPOS" class="DigNum (strict)"("Val(Sgnl)"=w200) -> ()  [unwired: 2 in, 2 out]
      "X COM PORT" <- w245
      "Z COM PORT" <- w244
      "Y COM PORT" <- w243
      "R COM PORT" <- w242
    }
  }
  n190 = property on="Z Step SP" class="DigNum (strict)"("Maximum"=102400000.0 ("upper limit")) -> ()  [unwired: 2 in, 2 out]
  n191 = property on="Z Step SP" class="DigNum (strict)"("Minimum"=0.0 ("lower limit")) -> ()  [unwired: 2 in, 2 out]
  n192 = property on="R Step SP" class="DigNum (strict)"("Maximum"=0.0 ("Data Entry Limits:Maximum")) -> ()  [unwired: 2 in, 2 out]
  n193 = property on="R Step SP" class="DigNum (strict)"("Minimum"=-6144000.0 ("Data Entry Limits:Minimum")) -> ()  [unwired: 2 in, 2 out]
  n194 = while {
    tunnel: [w269] -> w39
    tunnel: [w272] -> w40
    tunnel: [w275] -> w48
    tunnel: [w268] -> w47
    tunnel: [w274] -> w42
    tunnel: [w273] -> w41
    tunnel: [w271] -> w38
    tunnel: [w270] -> w37
    tunnel: w12 -> [w291]
    tunnel: w11 -> [w289]
    tunnel: w10 -> [w287]
    tunnel: w9 -> [w285]
    tunnel: w8 -> [w290]
    tunnel: w7 -> [w288]
    tunnel: w6 -> [w286]
    tunnel: w5 -> [w284]
    tunnel: w4 -> [w265]
    tunnel: w3 -> [w264]
    shift-right: [w258] -> _
    shift-left: dbl[] [] -> [w256]
    shift-right: [w257] -> _
    shift-left: dbl[] [] -> [w255]
    stop <- w266 stop-if-true
    n195 = event shown="[0] Timeout" {
      selector: _ -> [_ _ _ _ _ _ _ _ _ _ _ _ _ _ _ _]
      dyn-events: _ -> [_ _ _ _ _ _ _ _ _ _ _ _ _ _ _ _]
      timeout: 100 -> [_ _ _ _ _ _ _ _ _ _ _ _ _ _ _ _]
      tunnel: [w489 w1226 w1262 w1579 w1705 w1749 w1827 w1917 w1946 w1974 w2004 w2033 w2157 w2328 w2398 w2632] -> w281
      tunnel: [w490 w1221 w1263 w1580 w1702 w1746 w1824 w1914 w1943 w1972 w2001 w2030 w2154 w2329 w2399 w2633] -> w280
      tunnel: [w508 w1223 w1271 w1570 w1700 w1744 w1822 w1912 w1941 w1970 w1999 w2028 w2181 w2322 w2391 w2637] -> w277
      tunnel: [w507 w1228 w1270 w1569 w1707 w1751 w1829 w1919 w1948 w1977 w2006 w2035 w2180 w2321 w2389 w2636] -> w276
      tunnel: [w492 w1222 w1267 w1568 w1701 w1745 w1823 w1913 w1942 w1971 w2000 w2029 w2141 w2318 w2397 w2635] -> w278
      tunnel: [w491 w1227 w1266 w1567 w1706 w1750 w1828 w1918 w1947 w1976 w2005 w2034 w2140 w2317 w2396 w2634] -> w279
      tunnel: [w486 w1224 w1259 w1578 w1703 w1747 w1825 w1915 w1944 w1973 w2002 w2031 w2127 w2314 w2394 w2631] -> w283
      tunnel: [w485 w1225 w1258 w1577 w1704 w1748 w1826 w1916 w1945 w1975 w2003 w2032 w2126 w2313 w2393 w2630] -> w282
      tunnel: w291 -> [w484 w1223 w1273 w1573 w1700 w1744 w1822 w1912 w1941 w1970 w1999 w2028 w2176 w2312 w2387 w2625]
      tunnel: w290 -> [w483 w1228 w1272 w1598 w1707 w1751 w1829 w1919 w1948 w1977 w2006 w2035 w2177 w2310 w2386 w2629]
      tunnel: w289 -> [w482 w1222 w1268 w1576 w1701 w1745 w1823 w1913 w1942 w1971 w2000 w2029 w2142 w2311 w2385 w2624]
      tunnel: w288 -> [w481 w1227 w1269 w1597 w1706 w1750 w1828 w1918 w1947 w1976 w2005 w2034 w2143 w2309 w2384 w2628]
      tunnel: w287 -> [w480 w1221 w1264 w1583 w1702 w1746 w1824 w1914 w1943 w1972 w2001 w2030 w2155 w2308 w2383 w2623]
      tunnel: w286 -> [w479 w1226 w1265 w1596 w1705 w1749 w1827 w1917 w1946 w1974 w2004 w2033 w2156 w2306 w2382 w2627]
      tunnel: w285 -> [w478 w1224 w1260 w1586 w1703 w1747 w1825 w1915 w1944 w1973 w2002 w2031 w2128 w2307 w2381 w2622]
      tunnel: w284 -> [w477 w1225 w1261 w1595 w1704 w1748 w1826 w1916 w1945 w1975 w2003 w2032 w2129 w2305 w2380 w2626]
      tunnel: [w460 _ _ _ _ _ _ _ _ _ _ _ _ _ _ _] -> w258
      tunnel: [w458 _ _ _ _ _ _ _ _ _ _ _ _ _ _ _] -> w257
      tunnel: w256 -> [w463 _ _ _ _ _ _ _ _ _ _ _ _ _ _ _]
      tunnel: w255 -> [w462 _ _ _ _ _ _ _ _ _ _ _ _ _ _ _]
      event #0 {
        n196 = event-data() -> ()  [unwired: 1 in, 2 out]
        n197 = property on="GO" class="Bool"() -> ("DisabledEnum"=w476:T1)  [unwired: 2 in, 2 out]
        n198 = property on="GO" class="Bool"() -> ("DisabledEnum"=w473:T1)  [unwired: 2 in, 2 out]
        n199 = property on="Scan Go" class="Bool (strict)"() -> ("DisabledEnum"=w470:T1)  [unwired: 2 in, 2 out]
        n200 = Equal?(x=w476, y=T1."Disabled and Grayed Out") -> (x = y?=w474:bool)
        n201 = case shown="True" w474 {
          tunnel: [w531 w578] -> w508
          tunnel: [w530 w577] -> w507
          tunnel: [w529 w576] -> w492
          tunnel: [w528 w575] -> w491
          tunnel: [w527 w574] -> w490
          tunnel: [w526 w573] -> w489
          tunnel: [w525 w572] -> w486
          tunnel: [w524 w571] -> w485
          tunnel: w484 -> [w539 w570]
          tunnel: w483 -> [w538 w569]
          tunnel: w482 -> [w537 w568]
          tunnel: w481 -> [w536 w567]
          tunnel: w480 -> [w535 w566]
          tunnel: w479 -> [w534 w565]
          tunnel: w478 -> [w533 w564]
          tunnel: w477 -> [w532 w563]
          frame #0 {
            n202 = call "DigitalIO_sub_V1_MON.vi"() -> ("CL"=w518:bool, "OP"=w519:bool)  [unwired: 8 in]
            n203 = property on="CL" class="Bool (strict)"("Val(Sgnl)"=w518) -> ()  [unwired: 2 in, 2 out]
            n204 = property on="OP" class="Bool (strict)"("Val(Sgnl)"=w519) -> ()  [unwired: 2 in, 2 out]
            n205 = call "mDrive Send Command.vi"("error in (no error)"=w532, "Extra"="MV", "Command"=T10."Print Parameter", "VISA resource name"=w533) -> ("error out"=w524:errorcluster, "read buffer"=w541:string, "VISA resource name out"=w525:refnum<visa-resource-name>)  [unwired: 3 in]
            n206 = call "mDrive Send Command.vi"("error in (no error)"=w534, "Extra"="MV", "Command"=T10."Print Parameter", "VISA resource name"=w535) -> ("error out"=w526:errorcluster, "read buffer"=w545:string, "VISA resource name out"=w527:refnum<visa-resource-name>)  [unwired: 3 in]
            n207 = call "mDrive Send Command.vi"("error in (no error)"=w536, "Extra"="MV", "Command"=T10."Print Parameter", "VISA resource name"=w537) -> ("error out"=w528:errorcluster, "read buffer"=w549:string, "VISA resource name out"=w529:refnum<visa-resource-name>)  [unwired: 3 in]
            n208 = call "mDrive Send Command.vi"("error in (no error)"=w538, "Extra"="MV", "Command"=T10."Print Parameter", "VISA resource name"=w539) -> ("error out"=w530:errorcluster, "read buffer"=w553:string, "VISA resource name out"=w531:refnum<visa-resource-name>)  [unwired: 3 in]
            n209 = Not Equal?(x=w541, y="") -> (x != y?=w520:bool)
            n210 = Not Equal?(x=w545, y="") -> (x != y?=w521:bool)
            n211 = Not Equal?(x=w549, y="") -> (x != y?=w522:bool)
            n212 = Not Equal?(x=w553, y="") -> (x != y?=w523:bool)
            n213 = property on="R Ready" class="Bool (strict)"("Val(Sgnl)"=w520) -> ()  [unwired: 2 in, 2 out]
            n214 = property on="Z Ready" class="Bool (strict)"("Val(Sgnl)"=w522) -> ()  [unwired: 2 in, 2 out]
            n215 = property on="Y Ready" class="Bool (strict)"("Val(Sgnl)"=w521) -> ()  [unwired: 2 in, 2 out]
            n216 = property on="X Ready" class="Bool (strict)"("Val(Sgnl)"=w523) -> ()  [unwired: 2 in, 2 out]
          }
          frame #1 {
            n217 = flat-sequence {
              tunnel: [w957] -> w620
              tunnel: [w948] -> w619
              tunnel: [w947] -> w618
              tunnel: w568 -> [w951]
              tunnel: w567 -> [w950]
              tunnel: [w989] -> w617
              tunnel: [w988] -> w616
              tunnel: [w987] -> w615
              tunnel: [w980] -> w614
              tunnel: w620 -> [w987]
              tunnel: w619 -> [w986]
              tunnel: w618 -> [w985]
              tunnel: w617 -> [w999]
              tunnel: [w999] -> w613
              tunnel: w616 -> [w998]
              tunnel: [w998] -> w612
              tunnel: w615 -> [w997]
              tunnel: [w997] -> w611
              tunnel: w614 -> [w996]
              tunnel: [w996] -> w610
              tunnel: [w1003] -> w609
              tunnel: [w1004] -> w608
              tunnel: [w1000] -> w607
              tunnel: w610 -> [w1000]
              tunnel: w611 -> [w1001]
              tunnel: w612 -> [w1005]
              tunnel: w613 -> [w1002]
              tunnel: w609 -> [w1016]
              tunnel: w608 -> [w1017]
              tunnel: w607 -> [w1019]
              tunnel: [w1015] -> w575
              tunnel: [w1014] -> w576
              frame #0 {
                n218 = call "mDrive Send Command.vi"("error in (no error)"=w950, "Extra"="P", "Command"=T10."Print Parameter", "VISA resource name"=w951) -> ("error out"=w947:errorcluster, "read buffer"=w967:string, "VISA resource name out"=w948:refnum<visa-resource-name>)  [unwired: 3 in]
                n219 = property on="Z steps/rev" class="DigNum (strict)"() -> ("Value"=w956:u32)  [unwired: 2 in, 2 out]
                n220 = To Double Precision Float(number=w956) -> (double precision float=w963:dbl)
                n221 = Decimal String To Number(string=w967, offset=0) -> (number=w946:i32)  [unwired: 1 in, 1 out]
                n222 = To Double Precision Float(number=w946) -> (double precision float=w961:dbl)
                n223 = Divide(x=w961, y=w963) -> (x/y=w962:dbl)
                n224 = property on="Z Step PV" class="DigNum (strict)"("Val(Sgnl)"=w946) -> ()  [unwired: 2 in, 2 out]
                n225 = property on="Z mm/rev" class="DigNum (strict)"() -> ("Value"=w955:dbl)  [unwired: 2 in, 2 out]
                n226 = property on="Z Step SP" class="DigNum (strict)"() -> ("Maximum"=w958:dbl)  [unwired: 2 in, 2 out]
                n227 = property on="Z Step SP" class="DigNum (strict)"() -> ("Minimum"=w952:dbl)  [unwired: 2 in, 2 out]
                n228 = Multiply(x=w962, y=w955) -> (x*y=w949:dbl)
                n229 = To Long Integer(number=w958) -> (32bit integer=w964:i32)
                n230 = To Long Integer(number=w952) -> (32bit integer=w965:i32)
                n231 = property on="Z offset mm" class="DigNum (strict)"() -> ("Value"=w954:dbl)  [unwired: 2 in, 2 out]
                n232 = In Range and Coerce(upper limit=w964, x=w946, lower limit=w965) -> (In Range?=w957:bool)  [unwired: 1 out]
                n233 = Add(x=w949, y=w954) -> (x+y=w953:dbl)
                n234 = property on="Z Position mm PV" class="DigNum (strict)"("Val(Sgnl)"=w953) -> ()  [unwired: 2 in, 2 out]
                n235 = property on="Z in Range" class="Bool (strict)"("Val(Sgnl)"=w957) -> ()  [unwired: 2 in, 2 out]
                n236 = property on="OK Button" class="Bool (strict)"() -> ("Value"=w943:bool)  [unwired: 2 in, 2 out]
                n237 = Not Equal?(x=w943, y=TRUE) -> (x != y?=w941:bool)
                n238 = Equal?(x=w946, y=15360000) -> (x = y?=w940:bool)
                n239 = And(x=w940, y=w941) -> (x .and. y?=w939:bool)
                n240 = case shown="True" w939 {
                  tunnel: [FALSE ("true") w978] -> w944
                  frame #0 {
                  }
                  frame #1 {
                    n241 = One Button Dialog(message="HAVE YOU OPEND THE VALVE???\nTHEN REWRITE YOUR POSITION\n AND PRESS GO!") -> (true=w978:bool)  [unwired: 1 in]
                  }
                }
                n242 = case shown="True" w944 {
                  frame #0 {
                    n243 = call "DigitalIO_sub_V1_MON.vi"() -> ("CL"=w968:bool, "OP"=w969:bool)  [unwired: 8 in]
                    n244 = property on="OP" class="Bool (strict)"("Val(Sgnl)"=w969) -> ()  [unwired: 2 in, 2 out]
                    n245 = property on="CL" class="Bool (strict)"("Val(Sgnl)"=w968) -> ()  [unwired: 2 in, 2 out]
                  }
                  frame #1 {
                    n246 = while {
                      stop <- w976 stop-if-true
                      n247 = property on="OK Button" class="Bool (strict)"() -> ("Value"=w970:bool)  [unwired: 2 in, 2 out]
                      n248 = call "ValveConrtoller.vi"("OK Button"=w970) -> ("OUTGOING SIGNAL"=w971:bool, "CL"=w972:bool, "OP"=w973:bool, "VALVE\nopend/closed"=w974:bool)  [unwired: 3 in]
                      n249 = property on="Valve \nopend/closed" class="Bool (strict)"("Val(Sgnl)"=w974) -> ()  [unwired: 2 in, 2 out]
                      n250 = property on="CL" class="Bool (strict)"("Val(Sgnl)"=w972) -> ()  [unwired: 2 in, 2 out]
                      n251 = Equal?(x=w971, y=TRUE) -> (x = y?=w976:bool)
                      n252 = property on="OP" class="Bool (strict)"("Val(Sgnl)"=w973) -> ()  [unwired: 2 in, 2 out]
                    }
                  }
                }
              }
              frame #1 {
                n253 = call "mDrive Send Command.vi"("error in (no error)"=w985, "Extra"="MV", "Command"=T10."Print Parameter", "VISA resource name"=w986) -> ("error out"=w988:errorcluster, "read buffer"=w991:string, "VISA resource name out"=w989:refnum<visa-resource-name>)  [unwired: 3 in]
                n254 = Not Equal?(x=w991, y="") -> (x != y?=w984:bool)
                n255 = Decimal String To Number(string=w991, offset=0 ("offset (0)")) -> (number=w981:i32)  [unwired: 1 in, 1 out]
                n256 = property on="Z Ready" class="Bool (strict)"("Val(Sgnl)"=w984) -> ()  [unwired: 2 in, 2 out]
                n257 = Number To Boolean Array(number=w981) -> (Boolean array=w983:bool[])
                n258 = Index Array(array=w983, index=0) -> (element=w980:bool)
                n259 = property on="Z in Motion" class="Bool (strict)"("Val(Sgnl)"=w980) -> ()  [unwired: 2 in, 2 out]
              }
              frame #2 {
                n260 = Wait (ms)(milliseconds to wait=u32 50) -> ()  [unwired: 1 out]
              }
              frame #3 {
                n261 = case shown="False" w1001 {
                  tunnel: w1002 -> [w1008 w1012]
                  tunnel: [w1009 w1012] -> w1003
                  tunnel: [w1010 w1011] -> w1004
                  tunnel: w1005 -> [w1007 w1011]
                  frame #0 {
                    n262 = call "mDrive Send Command.vi"("error in (no error)"=w1007, "Command"=T10."Stop", "VISA resource name"=w1008) -> ("error out"=w1010:errorcluster, "VISA resource name out"=w1009:refnum<visa-resource-name>)  [unwired: 4 in, 1 out]
                  }
                  frame #1 {
                  }
                }
              }
              frame #4 {
                n263 = property on="Z Backlash corr" class="Bool (strict)"() -> ("Value"=w1013:bool)  [unwired: 2 in, 2 out]
                n264 = Implies(1:w1019, 2:w1013) -> (0:w1018:bool)
                n265 = case shown="False" w1018 {
                  tunnel: w1017 -> [w1027 w1084]
                  tunnel: w1016 -> [w1026 w1085]
                  tunnel: [w1021 w1084] -> w1015
                  tunnel: [w1025 w1085] -> w1014
                  frame #0 {
                    # "Backlash"
                    n266 = flat-sequence {
                      tunnel: [w1040] -> w1039
                      tunnel: [w1044] -> w1038
                      tunnel: [w1043] -> w1037
                      tunnel: w1027 -> [w1042]
                      tunnel: w1026 -> [w1041]
                      tunnel: w1039 -> [w1052]
                      tunnel: [w1052] -> w1036
                      tunnel: w1038 -> [w1051]
                      tunnel: w1037 -> [w1050]
                      tunnel: [w1049] -> w1035
                      tunnel: [w1048] -> w1034
                      tunnel: [w1047] -> w1024
                      tunnel: w1036 -> [w1066]
                      tunnel: w1035 -> [w1057]
                      tunnel: w1034 -> [w1065]
                      tunnel: [w1057] -> w1033
                      tunnel: [w1065] -> w1032
                      tunnel: [w1056] -> w1029
                      tunnel: [w1064] -> w1028
                      tunnel: w1024 -> [w1064]
                      tunnel: w1033 -> [w1069]
                      tunnel: w1032 -> [w1070]
                      tunnel: [w1068] -> w1031
                      tunnel: [w1076] -> w1030
                      tunnel: w1029 -> [w1076]
                      tunnel: w1028 -> [w1072]
                      tunnel: [w1071] -> w1022
                      tunnel: w1031 -> [w1079]
                      tunnel: w1030 -> [w1078]
                      tunnel: [w1080] -> w1023
                      tunnel: w1022 -> [w1080]
                      tunnel: [w1079] -> w1020
                      tunnel: [w1083] -> w1025
                      tunnel: w1023 -> [w1083]
                      tunnel: [w1082] -> w1021
                      tunnel: w1020 -> [w1082]
                      frame #0 {
                        n267 = property on="Z Backlash steps/sec" class="DigNum (strict)"() -> ("Value"=w1040:i32)  [unwired: 2 in, 2 out]
                        n268 = Number To Decimal String(number=w1040) -> (decimal integer string=w1045:string)  [unwired: 1 in]
                        n269 = call "mDrive Send Command.vi"("error in (no error)"=w1042, "Extra"=w1045, "Command"=T10."Max Velocity", "VISA resource name"=w1041) -> ("error out"=w1043:errorcluster, "VISA resource name out"=w1044:refnum<visa-resource-name>)  [unwired: 3 in, 1 out]
                      }
                      frame #1 {
                        n270 = property on="Z Backlash" class="DigNum (strict)"() -> ("Value"=w1047:i32)  [unwired: 2 in, 2 out]
                        n271 = Number To Decimal String(number=w1047) -> (decimal integer string=w1053:string)  [unwired: 1 in]
                        n272 = call "mDrive Send Command.vi"("error in (no error)"=w1050, "Extra"=w1053, "Command"=T10."Move to Relative Position", "VISA resource name"=w1051) -> ("error out"=w1049:errorcluster, "VISA resource name out"=w1048:refnum<visa-resource-name>)  [unwired: 3 in, 1 out]
                      }
                      frame #2 {
                        n273 = To Double Precision Float(number=w1064) -> (double precision float=w1062:dbl)
                        n274 = To Double Precision Float(number=w1066) -> (double precision float=w1067:dbl)
                        n275 = Absolute Value(x=w1062) -> (abs(x)=w1063:dbl)
                        n276 = Divide(x=w1063, y=w1067) -> (x/y=w1060:dbl)
                        n277 = Multiply(x=1000.0, y=w1060) -> (x*y=w1058:dbl)
                        n278 = Add(x=w1058, y=300.0) -> (x+y=w1056:dbl)
                        n279 = To Unsigned Long Integer(number=w1056) -> (unsigned 32bit integer=w1055:u32)
                        n280 = Wait (ms)(milliseconds to wait=w1055) -> ()  [unwired: 1 out]
                      }
                      frame #3 {
                        n281 = Negate(x=w1072) -> (-x=w1073:i32)
                        n282 = Number To Decimal String(number=w1073) -> (decimal integer string=w1074:string)  [unwired: 1 in]
                        n283 = call "mDrive Send Command.vi"("error in (no error)"=w1069, "Extra"=w1074, "Command"=T10."Move to Relative Position", "VISA resource name"=w1070) -> ("error out"=w1068:errorcluster, "VISA resource name out"=w1071:refnum<visa-resource-name>)  [unwired: 3 in, 1 out]
                      }
                      frame #4 {
                        n284 = To Unsigned Long Integer(number=w1078) -> (unsigned 32bit integer=w1077:u32)
                        n285 = Wait (ms)(milliseconds to wait=w1077) -> ()  [unwired: 1 out]
                      }
                      frame #5 {
                        n286 = property on="Z Backlash corr" class="Bool (strict)"("Val(Sgnl)"=FALSE ("Value (Signaling)")) -> ()  [unwired: 2 in, 2 out]
                      }
                    }
                  }
                  frame #1 {
                  }
                }
              }
            }
            n287 = flat-sequence {
              tunnel: [w820] -> w606
              tunnel: [w822] -> w605
              tunnel: [w821] -> w604
              tunnel: w566 -> [w813]
              tunnel: w565 -> [w812]
              tunnel: [w842] -> w603
              tunnel: [w841] -> w602
              tunnel: [w840] -> w601
              tunnel: [w833] -> w600
              tunnel: w606 -> [w840]
              tunnel: w605 -> [w839]
              tunnel: w604 -> [w838]
              tunnel: w603 -> [w852]
              tunnel: [w852] -> w599
              tunnel: w602 -> [w851]
              tunnel: [w851] -> w598
              tunnel: w601 -> [w850]
              tunnel: [w850] -> w597
              tunnel: w600 -> [w849]
              tunnel: [w849] -> w596
              tunnel: [w856] -> w595
              tunnel: [w857] -> w594
              tunnel: [w853] -> w593
              tunnel: w596 -> [w853]
              tunnel: w597 -> [w854]
              tunnel: w598 -> [w858]
              tunnel: w599 -> [w855]
              tunnel: w595 -> [w869]
              tunnel: w594 -> [w870]
              tunnel: w593 -> [w872]
              tunnel: [w868] -> w573
              tunnel: [w867] -> w574
              frame #0 {
                n288 = call "mDrive Send Command.vi"("error in (no error)"=w812, "Extra"="P", "Command"=T10."Print Parameter", "VISA resource name"=w813) -> ("error out"=w821:errorcluster, "read buffer"=w832:string, "VISA resource name out"=w822:refnum<visa-resource-name>)  [unwired: 3 in]
                n289 = property on="Y steps/rev" class="DigNum (strict)"() -> ("Value"=w816:u32)  [unwired: 2 in, 2 out]
                n290 = Decimal String To Number(string=w832, offset=0) -> (number=w811:i32)  [unwired: 1 in, 1 out]
                n291 = To Double Precision Float(number=w816) -> (double precision float=w828:dbl)
                n292 = To Double Precision Float(number=w811) -> (double precision float=w825:dbl)
                n293 = property on="Y Step PV" class="DigNum (strict)"("Val(Sgnl)"=w811) -> ()  [unwired: 2 in, 2 out]
                n294 = Divide(x=w825, y=w828) -> (x/y=w827:dbl)
                n295 = property on="Y Step SP" class="DigNum (strict)"() -> ("Maximum"=w815:dbl)  [unwired: 2 in, 2 out]
                n296 = property on="Y Step SP" class="DigNum (strict)"() -> ("Minimum"=w814:dbl)  [unwired: 2 in, 2 out]
                n297 = property on="Y mm/rev" class="DigNum (strict)"() -> ("Value"=w817:dbl)  [unwired: 2 in, 2 out]
                n298 = To Long Integer(number=w815) -> (32bit integer=w829:i32)
                n299 = To Long Integer(number=w814) -> (32bit integer=w830:i32)
                n300 = Multiply(x=w827, y=w817) -> (x*y=w826:dbl)
                n301 = In Range and Coerce(upper limit=w829, x=w811, lower limit=w830) -> (In Range?=w820:bool)  [unwired: 1 out]
                n302 = property on="Y offset mm" class="DigNum (strict)"() -> ("Value"=w818:dbl)  [unwired: 2 in, 2 out]
                n303 = Add(x=w826, y=w818) -> (x+y=w819:dbl)
                n304 = property on="Y in Range" class="Bool (strict)"("Val(Sgnl)"=w820) -> ()  [unwired: 2 in, 2 out]
                n305 = property on="Y Position mm PV" class="DigNum (strict)"("Val(Sgnl)"=w819) -> ()  [unwired: 2 in, 2 out]
              }
              frame #1 {
                n306 = call "mDrive Send Command.vi"("error in (no error)"=w838, "Extra"="MV", "Command"=T10."Print Parameter", "VISA resource name"=w839) -> ("error out"=w841:errorcluster, "read buffer"=w844:string, "VISA resource name out"=w842:refnum<visa-resource-name>)  [unwired: 3 in]
                n307 = Not Equal?(x=w844, y="") -> (x != y?=w837:bool)
                n308 = Decimal String To Number(string=w844, offset=0 ("offset (0)")) -> (number=w834:i32)  [unwired: 1 in, 1 out]
                n309 = property on="Y Ready" class="Bool (strict)"("Val(Sgnl)"=w837) -> ()  [unwired: 2 in, 2 out]
                n310 = Number To Boolean Array(number=w834) -> (Boolean array=w836:bool[])
                n311 = Index Array(array=w836, index=0) -> (element=w833:bool)
                n312 = property on="Y in Motion" class="Bool (strict)"("Val(Sgnl)"=w833) -> ()  [unwired: 2 in, 2 out]
              }
              frame #2 {
                n313 = Wait (ms)(milliseconds to wait=u32 50) -> ()  [unwired: 1 out]
              }
              frame #3 {
                n314 = case shown="True" w854 {
                  tunnel: w855 -> [w861 w864]
                  tunnel: [w862 w864] -> w856
                  tunnel: [w863 w865] -> w857
                  tunnel: w858 -> [w860 w865]
                  frame #0 {
                    n315 = call "mDrive Send Command.vi"("error in (no error)"=w860, "Command"=T10."Stop", "VISA resource name"=w861) -> ("error out"=w863:errorcluster, "VISA resource name out"=w862:refnum<visa-resource-name>)  [unwired: 4 in, 1 out]
                  }
                  frame #1 {
                  }
                }
              }
              frame #4 {
                n316 = property on="Y Backlash corr" class="Bool (strict)"() -> ("Value"=w866:bool)  [unwired: 2 in, 2 out]
                n317 = Implies(1:w872, 2:w866) -> (0:w871:bool)
                n318 = case shown="False" w871 {
                  tunnel: w870 -> [w880 w937]
                  tunnel: w869 -> [w879 w938]
                  tunnel: [w874 w937] -> w868
                  tunnel: [w878 w938] -> w867
                  frame #0 {
                    # "Backlash"
                    n319 = flat-sequence {
                      tunnel: [w893] -> w892
                      tunnel: [w897] -> w891
                      tunnel: [w896] -> w890
                      tunnel: w880 -> [w895]
                      tunnel: w879 -> [w894]
                      tunnel: w892 -> [w905]
                      tunnel: [w905] -> w889
                      tunnel: w891 -> [w904]
                      tunnel: w890 -> [w903]
                      tunnel: [w902] -> w888
                      tunnel: [w901] -> w887
                      tunnel: [w900] -> w877
                      tunnel: w889 -> [w919]
                      tunnel: w888 -> [w910]
                      tunnel: w887 -> [w918]
                      tunnel: [w910] -> w886
                      tunnel: [w918] -> w885
                      tunnel: [w909] -> w882
                      tunnel: [w917] -> w881
                      tunnel: w877 -> [w917]
                      tunnel: w886 -> [w922]
                      tunnel: w885 -> [w923]
                      tunnel: [w921] -> w884
                      tunnel: [w929] -> w883
                      tunnel: w882 -> [w929]
                      tunnel: w881 -> [w925]
                      tunnel: [w924] -> w875
                      tunnel: w884 -> [w932]
                      tunnel: w883 -> [w931]
                      tunnel: [w933] -> w876
                      tunnel: w875 -> [w933]
                      tunnel: [w932] -> w873
                      tunnel: [w936] -> w878
                      tunnel: w876 -> [w936]
                      tunnel: [w935] -> w874
                      tunnel: w873 -> [w935]
                      frame #0 {
                        n320 = property on="Y Backlash steps/sec" class="DigNum (strict)"() -> ("Value"=w893:i32)  [unwired: 2 in, 2 out]
                        n321 = Number To Decimal String(number=w893) -> (decimal integer string=w898:string)  [unwired: 1 in]
                        n322 = call "mDrive Send Command.vi"("error in (no error)"=w895, "Extra"=w898, "Command"=T10."Max Velocity", "VISA resource name"=w894) -> ("error out"=w896:errorcluster, "VISA resource name out"=w897:refnum<visa-resource-name>)  [unwired: 3 in, 1 out]
                      }
                      frame #1 {
                        n323 = property on="Y Backlash" class="DigNum (strict)"() -> ("Value"=w900:i32)  [unwired: 2 in, 2 out]
                        n324 = Number To Decimal String(number=w900) -> (decimal integer string=w906:string)  [unwired: 1 in]
                        n325 = call "mDrive Send Command.vi"("error in (no error)"=w903, "Extra"=w906, "Command"=T10."Move to Relative Position", "VISA resource name"=w904) -> ("error out"=w902:errorcluster, "VISA resource name out"=w901:refnum<visa-resource-name>)  [unwired: 3 in, 1 out]
                      }
                      frame #2 {
                        n326 = To Double Precision Float(number=w917) -> (double precision float=w915:dbl)
                        n327 = To Double Precision Float(number=w919) -> (double precision float=w920:dbl)
                        n328 = Absolute Value(x=w915) -> (abs(x)=w916:dbl)
                        n329 = Divide(x=w916, y=w920) -> (x/y=w913:dbl)
                        n330 = Multiply(x=1000.0, y=w913) -> (x*y=w911:dbl)
                        n331 = Add(x=w911, y=300.0) -> (x+y=w909:dbl)
                        n332 = To Unsigned Long Integer(number=w909) -> (unsigned 32bit integer=w908:u32)
                        n333 = Wait (ms)(milliseconds to wait=w908) -> ()  [unwired: 1 out]
                      }
                      frame #3 {
                        n334 = Negate(x=w925) -> (-x=w926:i32)
                        n335 = Number To Decimal String(number=w926) -> (decimal integer string=w927:string)  [unwired: 1 in]
                        n336 = call "mDrive Send Command.vi"("error in (no error)"=w922, "Extra"=w927, "Command"=T10."Move to Relative Position", "VISA resource name"=w923) -> ("error out"=w921:errorcluster, "VISA resource name out"=w924:refnum<visa-resource-name>)  [unwired: 3 in, 1 out]
                      }
                      frame #4 {
                        n337 = To Unsigned Long Integer(number=w931) -> (unsigned 32bit integer=w930:u32)
                        n338 = Wait (ms)(milliseconds to wait=w930) -> ()  [unwired: 1 out]
                      }
                      frame #5 {
                        n339 = property on="Y Backlash corr" class="Bool (strict)"("Val(Sgnl)"=FALSE ("Value (Signaling)")) -> ()  [unwired: 2 in, 2 out]
                      }
                    }
                  }
                  frame #1 {
                  }
                }
              }
            }
            n340 = flat-sequence {
              tunnel: [w692] -> w592
              tunnel: [w694] -> w591
              tunnel: [w693] -> w590
              tunnel: w564 -> [w685]
              tunnel: w563 -> [w684]
              tunnel: [w714] -> w589
              tunnel: [w713] -> w588
              tunnel: [w712] -> w587
              tunnel: [w705] -> w586
              tunnel: w592 -> [w712]
              tunnel: w591 -> [w711]
              tunnel: w590 -> [w710]
              tunnel: w589 -> [w724]
              tunnel: [w724] -> w585
              tunnel: w588 -> [w723]
              tunnel: [w723] -> w584
              tunnel: w587 -> [w722]
              tunnel: [w722] -> w583
              tunnel: w586 -> [w721]
              tunnel: [w721] -> w582
              tunnel: [w728] -> w581
              tunnel: [w729] -> w580
              tunnel: [w725] -> w579
              tunnel: w582 -> [w725]
              tunnel: w583 -> [w726]
              tunnel: w584 -> [w730]
              tunnel: w585 -> [w727]
              tunnel: w581 -> [w741]
              tunnel: w580 -> [w742]
              tunnel: w579 -> [w744]
              tunnel: [w740] -> w571
              tunnel: [w739] -> w572
              frame #0 {
                n341 = call "mDrive Send Command.vi"("error in (no error)"=w684, "Extra"="P", "Command"=T10."Print Parameter", "VISA resource name"=w685) -> ("error out"=w693:errorcluster, "read buffer"=w704:string, "VISA resource name out"=w694:refnum<visa-resource-name>)  [unwired: 3 in]
                n342 = property on="R steps/rev" class="DigNum (strict)"() -> ("Value"=w686:u32)  [unwired: 2 in, 2 out]
                n343 = Decimal String To Number(string=w704, offset=0) -> (number=w683:i32)  [unwired: 1 in, 1 out]
                n344 = To Double Precision Float(number=w686) -> (double precision float=w700:dbl)
                n345 = To Double Precision Float(number=w683) -> (double precision float=w697:dbl)
                n346 = property on="R Step PV" class="DigNum (strict)"("Val(Sgnl)"=w683) -> ()  [unwired: 2 in, 2 out]
                n347 = Divide(x=w697, y=w700) -> (x/y=w699:dbl)
                n348 = property on="R Step SP" class="DigNum (strict)"() -> ("Maximum"=w687:dbl)  [unwired: 2 in, 2 out]
                n349 = property on="R Step SP" class="DigNum (strict)"() -> ("Minimum"=w688:dbl)  [unwired: 2 in, 2 out]
                n350 = property on="R deg/rev" class="DigNum (strict)"() -> ("Value"=w689:dbl)  [unwired: 2 in, 2 out]
                n351 = Multiply(x=w699, y=w689) -> (x*y=w698:dbl)
                n352 = To Long Integer(number=w687) -> (32bit integer=w701:i32)
                n353 = To Long Integer(number=w688) -> (32bit integer=w702:i32)
                n354 = property on="R offset deg" class="DigNum (strict)"() -> ("Value"=w690:dbl)  [unwired: 2 in, 2 out]
                n355 = In Range and Coerce(upper limit=w701, x=w683, lower limit=w702) -> (In Range?=w692:bool)  [unwired: 1 out]
                n356 = Add(x=w698, y=w690) -> (x+y=w691:dbl)
                n357 = property on="R in Range" class="Bool (strict)"("Val(Sgnl)"=w692) -> ()  [unwired: 2 in, 2 out]
                n358 = property on="R Position deg PV" class="DigNum (strict)"("Val(Sgnl)"=w691) -> ()  [unwired: 2 in, 2 out]
              }
              frame #1 {
                n359 = call "mDrive Send Command.vi"("error in (no error)"=w710, "Extra"="MV", "Command"=T10."Print Parameter", "VISA resource name"=w711) -> ("error out"=w713:errorcluster, "read buffer"=w716:string, "VISA resource name out"=w714:refnum<visa-resource-name>)  [unwired: 3 in]
                n360 = Not Equal?(x=w716, y="") -> (x != y?=w709:bool)
                n361 = Decimal String To Number(string=w716, offset=0 ("offset (0)")) -> (number=w706:i32)  [unwired: 1 in, 1 out]
                n362 = Number To Boolean Array(number=w706) -> (Boolean array=w708:bool[])
                n363 = property on="R Ready" class="Bool (strict)"("Val(Sgnl)"=w709) -> ()  [unwired: 2 in, 2 out]
                n364 = Index Array(array=w708, index=0) -> (element=w705:bool)
                n365 = property on="R in Motion" class="Bool (strict)"("Val(Sgnl)"=w705) -> ()  [unwired: 2 in, 2 out]
              }
              frame #2 {
                n366 = Wait (ms)(milliseconds to wait=u32 50) -> ()  [unwired: 1 out]
              }
              frame #3 {
                n367 = case shown="True" w726 {
                  tunnel: w727 -> [w733 w737]
                  tunnel: [w734 w737] -> w728
                  tunnel: [w735 w736] -> w729
                  tunnel: w730 -> [w732 w736]
                  frame #0 {
                    n368 = call "mDrive Send Command.vi"("error in (no error)"=w732, "Command"=T10."Stop", "VISA resource name"=w733) -> ("error out"=w735:errorcluster, "VISA resource name out"=w734:refnum<visa-resource-name>)  [unwired: 4 in, 1 out]
                  }
                  frame #1 {
                  }
                }
              }
              frame #4 {
                n369 = property on="R Backlash corr" class="Bool (strict)"() -> ("Value"=w738:bool)  [unwired: 2 in, 2 out]
                n370 = Implies(1:w744, 2:w738) -> (0:w743:bool)
                n371 = case shown="False" w743 {
                  tunnel: w742 -> [w752 w809]
                  tunnel: w741 -> [w751 w810]
                  tunnel: [w746 w809] -> w740
                  tunnel: [w750 w810] -> w739
                  frame #0 {
                    # "Backlash"
                    n372 = flat-sequence {
                      tunnel: [w765] -> w764
                      tunnel: [w769] -> w763
                      tunnel: [w768] -> w762
                      tunnel: w752 -> [w767]
                      tunnel: w751 -> [w766]
                      tunnel: w764 -> [w777]
                      tunnel: [w777] -> w761
                      tunnel: w763 -> [w776]
                      tunnel: w762 -> [w775]
                      tunnel: [w774] -> w760
                      tunnel: [w773] -> w759
                      tunnel: [w772] -> w749
                      tunnel: w761 -> [w791]
                      tunnel: w760 -> [w782]
                      tunnel: w759 -> [w790]
                      tunnel: [w782] -> w758
                      tunnel: [w790] -> w757
                      tunnel: [w781] -> w754
                      tunnel: [w789] -> w753
                      tunnel: w749 -> [w789]
                      tunnel: w758 -> [w794]
                      tunnel: w757 -> [w795]
                      tunnel: [w793] -> w756
                      tunnel: [w801] -> w755
                      tunnel: w754 -> [w801]
                      tunnel: w753 -> [w797]
                      tunnel: [w796] -> w747
                      tunnel: w756 -> [w804]
                      tunnel: w755 -> [w803]
                      tunnel: [w805] -> w748
                      tunnel: w747 -> [w805]
                      tunnel: [w804] -> w745
                      tunnel: [w808] -> w750
                      tunnel: w748 -> [w808]
                      tunnel: [w807] -> w746
                      tunnel: w745 -> [w807]
                      frame #0 {
                        n373 = property on="R Backlash steps/sec" class="DigNum (strict)"() -> ("Value"=w765:i32)  [unwired: 2 in, 2 out]
                        n374 = Number To Decimal String(number=w765) -> (decimal integer string=w770:string)  [unwired: 1 in]
                        n375 = call "mDrive Send Command.vi"("error in (no error)"=w767, "Extra"=w770, "Command"=T10."Max Velocity", "VISA resource name"=w766) -> ("error out"=w768:errorcluster, "VISA resource name out"=w769:refnum<visa-resource-name>)  [unwired: 3 in, 1 out]
                      }
                      frame #1 {
                        n376 = property on="R Backlash" class="DigNum (strict)"() -> ("Value"=w772:i32)  [unwired: 2 in, 2 out]
                        n377 = Number To Decimal String(number=w772) -> (decimal integer string=w778:string)  [unwired: 1 in]
                        n378 = call "mDrive Send Command.vi"("error in (no error)"=w775, "Extra"=w778, "Command"=T10."Move to Relative Position", "VISA resource name"=w776) -> ("error out"=w774:errorcluster, "VISA resource name out"=w773:refnum<visa-resource-name>)  [unwired: 3 in, 1 out]
                      }
                      frame #2 {
                        n379 = To Double Precision Float(number=w789) -> (double precision float=w787:dbl)
                        n380 = To Double Precision Float(number=w791) -> (double precision float=w792:dbl)
                        n381 = Absolute Value(x=w787) -> (abs(x)=w788:dbl)
                        n382 = Divide(x=w788, y=w792) -> (x/y=w785:dbl)
                        n383 = Multiply(x=1000.0, y=w785) -> (x*y=w783:dbl)
                        n384 = Add(x=w783, y=300.0) -> (x+y=w781:dbl)
                        n385 = To Unsigned Long Integer(number=w781) -> (unsigned 32bit integer=w780:u32)
                        n386 = Wait (ms)(milliseconds to wait=w780) -> ()  [unwired: 1 out]
                      }
                      frame #3 {
                        n387 = Negate(x=w797) -> (-x=w798:i32)
                        n388 = Number To Decimal String(number=w798) -> (decimal integer string=w799:string)  [unwired: 1 in]
                        n389 = call "mDrive Send Command.vi"("error in (no error)"=w794, "Extra"=w799, "Command"=T10."Move to Relative Position", "VISA resource name"=w795) -> ("error out"=w793:errorcluster, "VISA resource name out"=w796:refnum<visa-resource-name>)  [unwired: 3 in, 1 out]
                      }
                      frame #4 {
                        n390 = To Unsigned Long Integer(number=w803) -> (unsigned 32bit integer=w802:u32)
                        n391 = Wait (ms)(milliseconds to wait=w802) -> ()  [unwired: 1 out]
                      }
                      frame #5 {
                        n392 = property on="R Backlash corr" class="Bool (strict)"("Val(Sgnl)"=FALSE ("Value (Signaling)")) -> ()  [unwired: 2 in, 2 out]
                      }
                    }
                  }
                  frame #1 {
                  }
                }
              }
            }
            n393 = flat-sequence {
              tunnel: [w1091] -> w634
              tunnel: [w1090] -> w633
              tunnel: [w1089] -> w632
              tunnel: w570 -> [w1088]
              tunnel: w569 -> [w1087]
              tunnel: [w1113] -> w631
              tunnel: [w1112] -> w630
              tunnel: [w1110] -> w629
              tunnel: [w1111] -> w628
              tunnel: w634 -> [w1110]
              tunnel: w633 -> [w1109]
              tunnel: w632 -> [w1108]
              tunnel: w631 -> [w1127]
              tunnel: [w1127] -> w627
              tunnel: w630 -> [w1126]
              tunnel: [w1126] -> w626
              tunnel: w629 -> [w1125]
              tunnel: [w1125] -> w625
              tunnel: w628 -> [w1124]
              tunnel: [w1124] -> w624
              tunnel: [w1131] -> w623
              tunnel: [w1132] -> w622
              tunnel: [w1128] -> w621
              tunnel: w624 -> [w1128]
              tunnel: w625 -> [w1129]
              tunnel: w626 -> [w1133]
              tunnel: w627 -> [w1130]
              tunnel: w623 -> [w1143]
              tunnel: w622 -> [w1144]
              tunnel: w621 -> [w1146]
              tunnel: [w1142] -> w577
              tunnel: [w1141] -> w578
              frame #0 {
                n394 = call "mDrive Send Command.vi"("error in (no error)"=w1087, "Extra"="P", "Command"=T10."Print Parameter", "VISA resource name"=w1088) -> ("error out"=w1089:errorcluster, "read buffer"=w1107:string, "VISA resource name out"=w1090:refnum<visa-resource-name>)  [unwired: 3 in]
                n395 = Decimal String To Number(string=w1107, offset=0) -> (number=w1086:i32)  [unwired: 1 in, 1 out]
                n396 = property on="X steps/rev" class="DigNum (strict)"() -> ("Value"=w1100:u32)  [unwired: 2 in, 2 out]
                n397 = To Double Precision Float(number=w1086) -> (double precision float=w1095:dbl)
                n398 = To Double Precision Float(number=w1100) -> (double precision float=w1101:dbl)
                n399 = property on="X Step PV" class="DigNum (strict)"("Val(Sgnl)"=w1086) -> ()  [unwired: 2 in, 2 out]
                n400 = Divide(x=w1095, y=w1101) -> (x/y=w1099:dbl)
                n401 = property on="X Step SP" class="DigNum (strict)"() -> ("Maximum"=w1103:dbl)  [unwired: 2 in, 2 out]
                n402 = property on="X Step SP" class="DigNum (strict)"() -> ("Minimum"=w1105:dbl)  [unwired: 2 in, 2 out]
                n403 = property on="X mm/rev" class="DigNum (strict)"() -> ("Value"=w1098:dbl)  [unwired: 2 in, 2 out]
                n404 = Multiply(x=w1099, y=w1098) -> (x*y=w1097:dbl)
                n405 = To Long Integer(number=w1103) -> (32bit integer=w1102:i32)
                n406 = To Long Integer(number=w1105) -> (32bit integer=w1104:i32)
                n407 = property on="X offset mm" class="DigNum (strict)"() -> ("Value"=w1096:dbl)  [unwired: 2 in, 2 out]
                n408 = In Range and Coerce(upper limit=w1102, x=w1086, lower limit=w1104) -> (In Range?=w1091:bool)  [unwired: 1 out]
                n409 = Add(x=w1097, y=w1096) -> (x+y=w1094:dbl)
                n410 = property on="X  in Range" class="Bool (strict)"("Val(Sgnl)"=w1091) -> ()  [unwired: 2 in, 2 out]
                n411 = property on="X Position mm PV" class="DigNum (strict)"("Val(Sgnl)"=w1094) -> ()  [unwired: 2 in, 2 out]
              }
              frame #1 {
                n412 = call "mDrive Send Command.vi"("error in (no error)"=w1108, "Extra"="MV", "Command"=T10."Print Parameter", "VISA resource name"=w1109) -> ("error out"=w1112:errorcluster, "read buffer"=w1116:string, "VISA resource name out"=w1113:refnum<visa-resource-name>)  [unwired: 3 in]
                n413 = Not Equal?(x=w1116, y="") -> (x != y?=w1114:bool)
                n414 = Decimal String To Number(string=w1116, offset=0 ("offset (0)")) -> (number=w1119:i32)  [unwired: 1 in, 1 out]
                n415 = property on="X Ready" class="Bool (strict)"("Val(Sgnl)"=w1114) -> ()  [unwired: 2 in, 2 out]
                n416 = Number To Boolean Array(number=w1119) -> (Boolean array=w1118:bool[])
                n417 = Index Array(array=w1118, index=0) -> (element=w1111:bool)
                n418 = property on="X  in Motion" class="Bool (strict)"("Val(Sgnl)"=w1111) -> ()  [unwired: 2 in, 2 out]
              }
              frame #2 {
                n419 = Wait (ms)(milliseconds to wait=u32 50) -> ()  [unwired: 1 out]
              }
              frame #3 {
                n420 = case shown="True" w1129 {
                  tunnel: w1130 -> [w1136 w1140]
                  tunnel: [w1137 w1140] -> w1131
                  tunnel: [w1138 w1139] -> w1132
                  tunnel: w1133 -> [w1135 w1139]
                  frame #0 {
                    n421 = call "mDrive Send Command.vi"("error in (no error)"=w1135, "Command"=T10."Stop", "VISA resource name"=w1136) -> ("error out"=w1138:errorcluster, "VISA resource name out"=w1137:refnum<visa-resource-name>)  [unwired: 4 in, 1 out]
                  }
                  frame #1 {
                  }
                }
              }
              frame #4 {
                n422 = property on="X Backlash corr" class="Bool (strict)"() -> ("Value"=w1147:bool)  [unwired: 2 in, 2 out]
                n423 = Implies(1:w1146, 2:w1147) -> (0:w1145:bool)
                n424 = case shown="False" w1145 {
                  tunnel: w1144 -> [w1155 w1212]
                  tunnel: w1143 -> [w1154 w1213]
                  tunnel: [w1149 w1212] -> w1142
                  tunnel: [w1153 w1213] -> w1141
                  frame #0 {
                    # "Backlash"
                    n425 = flat-sequence {
                      tunnel: [w1170] -> w1167
                      tunnel: [w1172] -> w1166
                      tunnel: [w1171] -> w1165
                      tunnel: w1155 -> [w1169]
                      tunnel: w1154 -> [w1168]
                      tunnel: w1167 -> [w1180]
                      tunnel: [w1180] -> w1164
                      tunnel: w1166 -> [w1179]
                      tunnel: w1165 -> [w1178]
                      tunnel: [w1177] -> w1163
                      tunnel: [w1176] -> w1162
                      tunnel: [w1175] -> w1152
                      tunnel: w1164 -> [w1194]
                      tunnel: w1163 -> [w1185]
                      tunnel: w1162 -> [w1193]
                      tunnel: [w1185] -> w1161
                      tunnel: [w1193] -> w1160
                      tunnel: [w1184] -> w1157
                      tunnel: [w1192] -> w1156
                      tunnel: w1152 -> [w1192]
                      tunnel: w1161 -> [w1197]
                      tunnel: w1160 -> [w1198]
                      tunnel: [w1196] -> w1159
                      tunnel: [w1204] -> w1158
                      tunnel: w1157 -> [w1204]
                      tunnel: w1156 -> [w1200]
                      tunnel: [w1199] -> w1150
                      tunnel: w1159 -> [w1207]
                      tunnel: w1158 -> [w1206]
                      tunnel: [w1208] -> w1151
                      tunnel: w1150 -> [w1208]
                      tunnel: [w1207] -> w1148
                      tunnel: [w1211] -> w1153
                      tunnel: w1151 -> [w1211]
                      tunnel: [w1209] -> w1149
                      tunnel: w1148 -> [w1209]
                      frame #0 {
                        n426 = property on="X Backlash steps/sec" class="DigNum (strict)"() -> ("Value"=w1170:i32)  [unwired: 2 in, 2 out]
                        n427 = Number To Decimal String(number=w1170) -> (decimal integer string=w1173:string)  [unwired: 1 in]
                        n428 = call "mDrive Send Command.vi"("error in (no error)"=w1169, "Extra"=w1173, "Command"=T10."Max Velocity", "VISA resource name"=w1168) -> ("error out"=w1171:errorcluster, "VISA resource name out"=w1172:refnum<visa-resource-name>)  [unwired: 3 in, 1 out]
                      }
                      frame #1 {
                        n429 = property on="X Backlash" class="DigNum (strict)"() -> ("Value"=w1175:i32)  [unwired: 2 in, 2 out]
                        n430 = Number To Decimal String(number=w1175) -> (decimal integer string=w1181:string)  [unwired: 1 in]
                        n431 = call "mDrive Send Command.vi"("error in (no error)"=w1178, "Extra"=w1181, "Command"=T10."Move to Relative Position", "VISA resource name"=w1179) -> ("error out"=w1177:errorcluster, "VISA resource name out"=w1176:refnum<visa-resource-name>)  [unwired: 3 in, 1 out]
                      }
                      frame #2 {
                        n432 = To Double Precision Float(number=w1192) -> (double precision float=w1190:dbl)
                        n433 = To Double Precision Float(number=w1194) -> (double precision float=w1195:dbl)
                        n434 = Absolute Value(x=w1190) -> (abs(x)=w1191:dbl)
                        n435 = Divide(x=w1191, y=w1195) -> (x/y=w1188:dbl)
                        n436 = Multiply(x=1000.0, y=w1188) -> (x*y=w1186:dbl)
                        n437 = Add(x=w1186, y=300.0) -> (x+y=w1184:dbl)
                        n438 = To Unsigned Long Integer(number=w1184) -> (unsigned 32bit integer=w1183:u32)
                        n439 = Wait (ms)(milliseconds to wait=w1183) -> ()  [unwired: 1 out]
                      }
                      frame #3 {
                        n440 = Negate(x=w1200) -> (-x=w1201:i32)
                        n441 = Number To Decimal String(number=w1201) -> (decimal integer string=w1202:string)  [unwired: 1 in]
                        n442 = call "mDrive Send Command.vi"("error in (no error)"=w1197, "Extra"=w1202, "Command"=T10."Move to Relative Position", "VISA resource name"=w1198) -> ("error out"=w1196:errorcluster, "VISA resource name out"=w1199:refnum<visa-resource-name>)  [unwired: 3 in, 1 out]
                      }
                      frame #4 {
                        n443 = To Unsigned Long Integer(number=w1206) -> (unsigned 32bit integer=w1205:u32)
                        n444 = Wait (ms)(milliseconds to wait=w1205) -> ()  [unwired: 1 out]
                      }
                      frame #5 {
                        n445 = property on="X Backlash corr" class="Bool (strict)"("Val(Sgnl)"=FALSE ("Value (Signaling)")) -> ()  [unwired: 2 in, 2 out]
                      }
                    }
                  }
                  frame #1 {
                  }
                }
              }
            }
            n446 = property on="Scan Go" class="Bool (strict)"() -> ("Value"=w562:bool)  [unwired: 2 in, 2 out]
            n447 = property on="STATUS" class="Str"() -> ("Value"=w560:string)  [unwired: 2 in, 2 out]
            n448 = Equal?(x=w560, y="SCANNING MODE" ("STATUS")) -> (x = y?=w558:bool)
            n449 = Equal?(x=w562, y=TRUE) -> (x = y?=w557:bool)
            n450 = Or(x=w558, y=w557) -> (x .or. y?=w556:bool)
            n451 = case shown="True" w556 {
              frame #0 {
                n452 = property on="X  in Motion" class="Bool (strict)"() -> ("Value"=w639:bool)  [unwired: 2 in, 2 out]
                n453 = property on="Y in Motion" class="Bool (strict)"() -> ("Value"=w638:bool)  [unwired: 2 in, 2 out]
                n454 = property on="Z in Motion" class="Bool (strict)"() -> ("Value"=w641:bool)  [unwired: 2 in, 2 out]
                n455 = property on="R in Motion" class="Bool (strict)"() -> ("Value"=w640:bool)  [unwired: 2 in, 2 out]
                n456 = Compound Arithmetic op=AND(w639, w638, w641, w640) -> (w636:bool)
                n457 = Equal?(x=w636, y=FALSE) -> (x = y?=w637:bool)
                n458 = case shown="True" w637 {
                  frame #0 {
                  }
                  frame #1 {
                    n459 = property on="X Step SP" class="DigNum (strict)"() -> ("Value"=w649:i32)  [unwired: 2 in, 2 out]
                    n460 = property on="Y Step SP" class="DigNum (strict)"() -> ("Value"=w647:i32)  [unwired: 2 in, 2 out]
                    n461 = property on="Z Step SP" class="DigNum (strict)"() -> ("Value"=w645:i32)  [unwired: 2 in, 2 out]
                    n462 = property on="R Step SP" class="DigNum (strict)"() -> ("Value"=w642:i32)  [unwired: 2 in, 2 out]
                    n463 = property on="X Step PV" class="DigNum (strict)"() -> ("Value"=w648:i32)  [unwired: 2 in, 2 out]
                    n464 = property on="Y Step PV" class="DigNum (strict)"() -> ("Value"=w646:i32)  [unwired: 2 in, 2 out]
                    n465 = property on="Z Step PV" class="DigNum (strict)"() -> ("Value"=w644:i32)  [unwired: 2 in, 2 out]
                    n466 = property on="R Step PV" class="DigNum (strict)"() -> ("Value"=w643:i32)  [unwired: 2 in, 2 out]
                    n467 = Equal?(x=w649, y=w648) -> (x = y?=w654:bool)
                    n468 = Equal?(x=w647, y=w646) -> (x = y?=w653:bool)
                    n469 = Equal?(x=w645, y=w644) -> (x = y?=w651:bool)
                    n470 = Equal?(x=w642, y=w643) -> (x = y?=w652:bool)
                    n471 = Compound Arithmetic op=AND(w654, w653, w651, w652) -> (w650:bool)
                    n472 = case shown="True" w650 {
                      frame #0 {
                      }
                      frame #1 {
                        n473 = local write "STATUS"("DONE" ("STATUS")) -> ()
                        n474 = property on="GO" class="Bool"("DisabledEnum"=T1."Enabled" ("Disabled")) -> ()  [unwired: 2 in, 2 out]
                      }
                    }
                  }
                }
              }
              frame #1 {
                n475 = property on="X Scan Length SP steps" class="DigNum (strict)"() -> ("Value"=w668:i32)  [unwired: 2 in, 2 out]
                n476 = property on="Y Scan Length SP steps" class="DigNum (strict)"() -> ("Value"=w667:i32)  [unwired: 2 in, 2 out]
                n477 = property on="Z Scan Length SP steps" class="DigNum (strict)"() -> ("Value"=w666:i32)  [unwired: 2 in, 2 out]
                n478 = property on="R Scan Length SP steps" class="DigNum (strict)"() -> ("Value"=w665:i32)  [unwired: 2 in, 2 out]
                n479 = property on="X Step SP" class="DigNum (strict)"() -> ("Value"=w664:i32)  [unwired: 2 in, 2 out]
                n480 = property on="Y Step SP" class="DigNum (strict)"() -> ("Value"=w663:i32)  [unwired: 2 in, 2 out]
                n481 = property on="Z Step SP" class="DigNum (strict)"() -> ("Value"=w662:i32)  [unwired: 2 in, 2 out]
                n482 = property on="R Step SP" class="DigNum (strict)"() -> ("Value"=w661:i32)  [unwired: 2 in, 2 out]
                n483 = Add(x=w668, y=w664) -> (x+y=w677:i32)
                n484 = Add(x=w667, y=w663) -> (x+y=w676:i32)
                n485 = Add(x=w666, y=w662) -> (x+y=w675:i32)
                n486 = Add(x=w665, y=w661) -> (x+y=w674:i32)
                n487 = property on="X Step PV" class="DigNum (strict)"() -> ("Value"=w660:i32)  [unwired: 2 in, 2 out]
                n488 = property on="Y Step PV" class="DigNum (strict)"() -> ("Value"=w659:i32)  [unwired: 2 in, 2 out]
                n489 = property on="Z Step PV" class="DigNum (strict)"() -> ("Value"=w658:i32)  [unwired: 2 in, 2 out]
                n490 = property on="R Step PV" class="DigNum (strict)"() -> ("Value"=w657:i32)  [unwired: 2 in, 2 out]
                n491 = Equal?(x=w660, y=w677) -> (x = y?=w673:bool)
                n492 = Equal?(x=w659, y=w676) -> (x = y?=w672:bool)
                n493 = Equal?(x=w658, y=w675) -> (x = y?=w670:bool)
                n494 = Equal?(x=w657, y=w674) -> (x = y?=w671:bool)
                n495 = Compound Arithmetic op=AND(w673, w672, w670, w671) -> (w669:bool)
                n496 = case shown="True" w669 {
                  frame #0 {
                  }
                  frame #1 {
                    n497 = local write "Scan Go"(FALSE ("Scan Go")) -> ()
                    n498 = local write "STATUS"("DONE" ("STATUS")) -> ()
                    n499 = property on="Set Scan \nParameters" class="Bool"("DisabledEnum"=T1."Enabled" ("Disabled")) -> ()  [unwired: 2 in, 2 out]
                    n500 = property on="Set for Scan" class="Bool"("DisabledEnum"=T1."Enabled" ("Disabled")) -> ()  [unwired: 2 in, 2 out]
                    n501 = property on="GO" class="Bool"("DisabledEnum"=T1."Enabled" ("Disabled")) -> ()  [unwired: 2 in, 2 out]
                  }
                }
              }
            }
          }
        }
        n502 = Equal?(x=w470, y=T1."Disabled and Grayed Out") -> (x = y?=w467:bool)
        n503 = Equal?(x=w473, y=T1."Enabled") -> (x = y?=w471:bool)
        n504 = And(x=w471, y=w467) -> (x .and. y?=w468:bool)
        n505 = case shown="False" w467 {
          frame #0 {
            n506 = local write "STATUS"("SCANNING MODE" ("STATUS")) -> ()
          }
          frame #1 {
          }
        }
        n507 = case shown="False" w468 {
          frame #0 {
          }
          frame #1 {
            n508 = local write "STATUS"("") -> ()
          }
        }
        n509 = property on="Z Position mm PV" class="DigNum (strict)"() -> ("Value"=w466:dbl)  [unwired: 2 in, 2 out]
        n510 = property on="R Position deg PV" class="DigNum (strict)"() -> ("Value"=w504:dbl)  [unwired: 2 in, 2 out]
        n511 = call "Build XY Graph2"("Reset"=TRUE, "Y Input"=w504, "X Input"=w466) -> ("XY Graph"=→"ZR Graph":cluster{"Y":dbl[], "Y":dbl[]}[])  [unwired: 7 in, 1 out]
        n512 = property on="Y Position mm PV" class="DigNum (strict)"() -> ("Value"=w465:dbl)  [unwired: 2 in, 2 out]
        n513 = property on="X Position mm PV" class="DigNum (strict)"() -> ("Value"=w503:dbl)  [unwired: 2 in, 2 out]
        n514 = call "Build XY Graph"("Reset"=TRUE, "Y Input"=w465, "X Input"=w503) -> ("XY Graph"=→"XY Graph":cluster{"Y":dbl[], "Y":dbl[]}[])  [unwired: 7 in, 1 out]
        n515 = Build Array (concatenate)(w463, w466) -> (w461:dbl[])
        n516 = Build Array (concatenate)(w462, w465) -> (w459:dbl[])
        n517 = Bundle(w461, w459) -> (→"ZY Graph":cluster{dbl[], dbl[]})  [unwired: 1 in]
        n518 = property on="Y Scan Length SP steps" class="DigNum (strict)"() -> ("Value"=w493:i32)  [unwired: 2 in, 2 out]
        n519 = property on="Z Scan Length SP steps" class="DigNum (strict)"() -> ("Value"=w494:i32)  [unwired: 2 in, 2 out]
        n520 = To Double Precision Float(number=w494) -> (double precision float=w487:dbl)
        n521 = To Double Precision Float(number=w493) -> (double precision float=w488:dbl)
        n522 = Divide(x=w488, y=w487) -> (x/y=w495:dbl)
        n523 = Inverse Tangent(1:w495) -> (0:w496:dbl)
        n524 = property on="Clear ZY" class="Bool (strict)"() -> ("Value"=w457:bool)  [unwired: 2 in, 2 out]
        n525 = Divide(x=w496, y=6.283185307179586) -> (x/y=w497:dbl)
        n526 = Multiply(x=360.0, y=w497) -> (x*y=w500:dbl)
        n527 = case shown="False" w457 {
          tunnel: w461 -> [w510 w515]
          tunnel: [w510 w514] -> w460
          tunnel: w459 -> [w509 w513]
          tunnel: [w509 w512] -> w458
          frame #0 {
          }
          frame #1 {
            w511 = 0 ("dimension size")
            n528 = Reshape Array(w515, w511) -> (w514:dbl[])
            n529 = Reshape Array(w513, w511) -> (w512:dbl[])
          }
        }
        n530 = property on="atan Y/Z" class="DigNum (strict)"("Val(Sgnl)"=w500) -> ()  [unwired: 2 in, 2 out]
      }
      event #1 {
        n531 = event-data() -> ()  [unwired: 1 in, 5 out]
        n532 = property on="OK Button" class="Bool (strict)"() -> ("Value"=w1214:bool)  [unwired: 2 in, 2 out]
        n533 = property on="Z Step PV" class="DigNum (strict)"() -> ("Value"=w1219:i32)  [unwired: 2 in, 2 out]
        n534 = Greater?(x=w1219, y=15360000) -> (0:w1216:bool)
        n535 = Equal?(x=w1214, y=TRUE) -> (x = y?=w1217:bool)
        n536 = And(x=w1217, y=w1216) -> (x .and. y?=w1215:bool)
        n537 = case shown="False" w1215 {
          frame #0 {
            n538 = property on="Z Step PV" class="DigNum (strict)"() -> ("Value"=w1235:i32)  [unwired: 2 in, 2 out]
            n539 = property on="OK Button" class="Bool (strict)"() -> ("Value"=w1230:bool)  [unwired: 2 in, 2 out]
            n540 = Greater?(x=w1235, y=15360000) -> (0:w1233:bool)
            n541 = Equal?(x=w1230, y=FALSE) -> (x = y?=w1232:bool)
            n542 = And(x=w1232, y=w1233) -> (x .and. y?=w1231:bool)
            n543 = case shown="True" w1231 {
              frame #0 {
              }
              frame #1 {
                n544 = One Button Dialog(message="YOU CAN'T CLOSE THE VALVE\nWHEN YOU ARE IN THE THIS\nPOSITION!!") -> (true=w1237:bool)  [unwired: 1 in]
                n545 = property on="OK Button" class="Bool (strict)"("Val(Sgnl)"=w1237) -> ()  [unwired: 2 in, 2 out]
              }
            }
          }
          frame #1 {
            n546 = flat-sequence {
              frame #0 {
                n547 = local read "OK Button"() -> (w1240:bool)
                n548 = call "DigitalIO_sub_V1_CNTL.vi"("OK Button"=w1240) -> ("Boolean"=w1239:bool)  [unwired: 2 in]
                n549 = property on="Valve \nopend/closed" class="Bool (strict)"("Val(Sgnl)"=w1239) -> ()  [unwired: 2 in, 2 out]
              }
              frame #1 {
                n550 = call "DigitalIO_sub_V1_MON.vi"() -> ("CL"=w1242:bool, "OP"=w1241:bool)  [unwired: 8 in]
                n551 = property on="OP" class="Bool (strict)"("Val(Sgnl)"=w1241) -> ()  [unwired: 2 in, 2 out]
                n552 = property on="CL" class="Bool (strict)"("Val(Sgnl)"=w1242) -> ()  [unwired: 2 in, 2 out]
              }
              frame #2 {
                n553 = Wait (ms)(milliseconds to wait=u32 100) -> ()  [unwired: 1 out]
              }
            }
          }
        }
        n554 = local write "STATUS"("VALVE CHANGED" ("STATUS")) -> ()
      }
      event #2 {
        n555 = event-data() -> ()  [unwired: 1 in, 7 out]
        n556 = property on="X Position mm PV" class="DigNum (strict)"() -> ("Value"=w1256:dbl)  [unwired: 2 in, 2 out]
        n557 = property on="X Position SP mm" class="DigNum (strict)"() -> ("Value"=w1255:dbl)  [unwired: 2 in, 2 out]
        n558 = property on="Z Position mm PV" class="DigNum (strict)"() -> ("Value"=w1252:dbl)  [unwired: 2 in, 2 out]
        n559 = property on="Z Position SP mm" class="DigNum (strict)"() -> ("Value"=w1244:dbl)  [unwired: 2 in, 2 out]
        n560 = property on="R Position SP deg" class="DigNum (strict)"() -> ("Value"=w1247:dbl)  [unwired: 2 in, 2 out]
        n561 = property on="R Position deg PV" class="DigNum (strict)"() -> ("Value"=w1246:dbl)  [unwired: 2 in, 2 out]
        n562 = property on="Y Position mm PV" class="DigNum (strict)"() -> ("Value"=w1250:dbl)  [unwired: 2 in, 2 out]
        n563 = property on="Y Position SP mm" class="DigNum (strict)"() -> ("Value"=w1249:dbl)  [unwired: 2 in, 2 out]
        n564 = Not Equal?(x=w1256, y=w1255) -> (x != y?=w1254:bool)
        n565 = Not Equal?(x=w1252, y=w1244) -> (x != y?=w1253:bool)
        n566 = Not Equal?(x=w1250, y=w1249) -> (x != y?=w1251:bool)
        n567 = Not Equal?(x=w1247, y=w1246) -> (x != y?=w1248:bool)
        n568 = case shown="True" w1253 {
          tunnel: w1269 -> [w1414 w1421]
          tunnel: w1268 -> [w1415 w1420]
          tunnel: [w1415 w1419] -> w1267
          tunnel: [w1414 w1418] -> w1266
          frame #0 {
          }
          frame #1 {
            n569 = flat-sequence {
              tunnel: w1420 -> [w1443]
              tunnel: w1421 -> [w1444]
              tunnel: [w1444] -> w1417
              tunnel: [w1443] -> w1416
              tunnel: [w1459] -> w1435
              tunnel: [w1458] -> w1434
              tunnel: [w1446] -> w1433
              tunnel: w1417 -> [w1459]
              tunnel: w1416 -> [w1458]
              tunnel: [w1462] -> w1432
              tunnel: [w1461] -> w1431
              tunnel: [w1460] -> w1430
              tunnel: w1433 -> [w1460]
              tunnel: w1434 -> [w1461]
              tunnel: w1435 -> [w1462]
              tunnel: [w1478] -> w1429
              tunnel: [w1477] -> w1428
              tunnel: w1432 -> [w1476]
              tunnel: w1431 -> [w1475]
              tunnel: [w1474] -> w1427
              tunnel: w1430 -> [w1474]
              tunnel: w1429 -> [w1485]
              tunnel: [w1485] -> w1426
              tunnel: w1428 -> [w1484]
              tunnel: [w1484] -> w1425
              tunnel: w1427 -> [w1483]
              tunnel: [w1483] -> w1424
              tunnel: [w1490] -> w1423
              tunnel: [w1489] -> w1422
              tunnel: w1426 -> [w1488]
              tunnel: w1425 -> [w1487]
              tunnel: w1424 -> [w1486]
              tunnel: [w1494] -> w1418
              tunnel: [w1495] -> w1419
              tunnel: w1423 -> [w1495]
              tunnel: w1422 -> [w1494]
              frame #0 {
                n570 = property on="Z Position SP mm" class="DigNum (strict)"() -> ("Value"=w1438:dbl)  [unwired: 2 in, 2 out]
                n571 = property on="Z Position mm PV" class="DigNum (strict)"() -> ("Value"=w1436:dbl)  [unwired: 2 in, 2 out]
                n572 = Greater?(x=w1438, y=60.0) -> (0:w1441:bool)
                n573 = Less?(x=w1436, y=60.0) -> (x < y?=w1440:bool)
                n574 = And(x=w1440, y=w1441) -> (x .and. y?=w1442:bool)
                n575 = case shown="True" w1442 {
                  frame #0 {
                  }
                  frame #1 {
                    n576 = property on="Z Position SP mm" class="DigNum (strict)"("Val(Sgnl)"=60.0 ("Value (Signaling)")) -> ()  [unwired: 2 in, 2 out]
                  }
                }
              }
              frame #1 {
                n577 = property on="Z Position SP mm" class="DigNum (strict)"() -> ("Value"=w1452:dbl)  [unwired: 2 in, 2 out]
                n578 = property on="Z offset mm" class="DigNum (strict)"() -> ("Value"=w1453:dbl)  [unwired: 2 in, 2 out]
                n579 = property on="Z mm/rev" class="DigNum (strict)"() -> ("Value"=w1454:dbl)  [unwired: 2 in, 2 out]
                n580 = property on="Z steps/rev" class="DigNum (strict)"() -> ("Value"=w1455:u32)  [unwired: 2 in, 2 out]
                n581 = To Double Precision Float(number=w1455) -> (double precision float=w1451:dbl)
                n582 = Subtract(x=w1452, y=w1453) -> (x-y=w1448:dbl)
                n583 = Divide(x=w1448, y=w1454) -> (x/y=w1447:dbl)
                n584 = property on="Z Step SP" class="DigNum (strict)"() -> ("Maximum"=w1457:dbl)  [unwired: 2 in, 2 out]
                n585 = property on="Z Step SP" class="DigNum (strict)"() -> ("Minimum"=w1456:dbl)  [unwired: 2 in, 2 out]
                n586 = Multiply(x=w1447, y=w1451) -> (x*y=w1449:dbl)
                n587 = In Range and Coerce(upper limit=w1457, x=w1449, lower limit=w1456) -> (coerced(x)=w1450:dbl)  [unwired: 1 out]
                n588 = To Long Integer(number=w1450) -> (32bit integer=w1446:i32)
                n589 = property on="Z Step SP" class="DigNum (strict)"("Val(Sgnl)"=w1446) -> ()  [unwired: 2 in, 2 out]
              }
              frame #2 {
                n590 = property on="Z Step SP" class="DigNum (strict)"() -> ("Value"=w1471:i32)  [unwired: 2 in, 2 out]
                n591 = property on="Z Step PV" class="DigNum (strict)"() -> ("Value"=w1470:i32)  [unwired: 2 in, 2 out]
                n592 = property on="Z Backlash" class="DigNum (strict)"() -> ("Value"=w1463:i32)  [unwired: 2 in, 2 out]
                n593 = Subtract(x=w1471, y=w1470) -> (x-y=w1469:i32)
                n594 = Sign(1:w1463) -> (0:w1467:i32)
                n595 = Sign(1:w1469) -> (0:w1468:i32)
                n596 = Multiply(x=w1468, y=w1467) -> (x*y=w1466:i32)
                n597 = Equal?(x=w1466, y=1) -> (x = y?=w1464:bool)
                n598 = case shown="False" w1464 {
                  frame #0 {
                    n599 = property on="Z Backlash corr" class="Bool (strict)"("Val(Sgnl)"=FALSE ("Value (Signaling)")) -> ()  [unwired: 2 in, 2 out]
                  }
                  frame #1 {
                    n600 = property on="Z Backlash corr" class="Bool (strict)"("Val(Sgnl)"=TRUE ("Value (Signaling)")) -> ()  [unwired: 2 in, 2 out]
                  }
                }
              }
              frame #3 {
                # "Velocity Setting"
                n601 = property on="Z Velocity SP step/sec" class="DigNum (strict)"() -> ("Value"=w1479:i32)  [unwired: 2 in, 2 out]
                n602 = Number To Decimal String(number=w1479) -> (decimal integer string=w1480:string)  [unwired: 1 in]
                n603 = call "mDrive Send Command.vi"("error in (no error)"=w1476, "Extra"=w1480, "Command"=T10."Max Velocity", "VISA resource name"=w1475) -> ("error out"=w1477:errorcluster, "VISA resource name out"=w1478:refnum<visa-resource-name>)  [unwired: 3 in, 1 out]
              }
              frame #4 {
                n604 = Wait (ms)(milliseconds to wait=u32 50) -> ()  [unwired: 1 out]
              }
              frame #5 {
                # "Move to Abs Position"
                n605 = Number To Decimal String(number=w1486) -> (decimal integer string=w1492:string)  [unwired: 1 in]
                n606 = call "mDrive Send Command.vi"("error in (no error)"=w1487, "Extra"=w1492, "Command"=T10."Move to Absolute Position", "VISA resource name"=w1488) -> ("error out"=w1489:errorcluster, "VISA resource name out"=w1490:refnum<visa-resource-name>)  [unwired: 3 in, 1 out]
              }
              frame #6 {
                n607 = Wait (ms)(milliseconds to wait=u32 50) -> ()  [unwired: 1 out]
              }
            }
          }
        }
        n608 = case shown="True" w1254 {
          tunnel: w1273 -> [w1497 w1501]
          tunnel: w1272 -> [w1496 w1500]
          tunnel: [w1497 w1499] -> w1271
          tunnel: [w1496 w1498] -> w1270
          frame #0 {
          }
          frame #1 {
            n609 = flat-sequence {
              tunnel: w1500 -> [w1528]
              tunnel: w1501 -> [w1529]
              tunnel: [w1529] -> w1515
              tunnel: [w1528] -> w1514
              tunnel: [w1517] -> w1513
              tunnel: [w1532] -> w1512
              tunnel: [w1531] -> w1511
              tunnel: [w1530] -> w1510
              tunnel: w1513 -> [w1530]
              tunnel: w1514 -> [w1531]
              tunnel: w1515 -> [w1532]
              tunnel: [w1548] -> w1509
              tunnel: [w1547] -> w1508
              tunnel: w1512 -> [w1546]
              tunnel: w1511 -> [w1545]
              tunnel: w1510 -> [w1544]
              tunnel: [w1544] -> w1507
              tunnel: w1509 -> [w1555]
              tunnel: [w1555] -> w1506
              tunnel: w1508 -> [w1554]
              tunnel: [w1554] -> w1505
              tunnel: [w1552] -> w1504
              tunnel: w1507 -> [w1552]
              tunnel: [w1560] -> w1503
              tunnel: [w1559] -> w1502
              tunnel: w1506 -> [w1558]
              tunnel: w1505 -> [w1557]
              tunnel: w1504 -> [w1556]
              tunnel: [w1564] -> w1498
              tunnel: [w1565] -> w1499
              tunnel: w1503 -> [w1565]
              tunnel: w1502 -> [w1564]
              frame #0 {
                n610 = property on="X Position SP mm" class="DigNum (strict)"() -> ("Value"=w1525:dbl)  [unwired: 2 in, 2 out]
                n611 = property on="X offset mm" class="DigNum (strict)"() -> ("Value"=w1526:dbl)  [unwired: 2 in, 2 out]
                n612 = property on="X mm/rev" class="DigNum (strict)"() -> ("Value"=w1516:dbl)  [unwired: 2 in, 2 out]
                n613 = property on="X steps/rev" class="DigNum (strict)"() -> ("Value"=w1527:u32)  [unwired: 2 in, 2 out]
                n614 = To Double Precision Float(number=w1527) -> (double precision float=w1522:dbl)
                n615 = Subtract(x=w1525, y=w1526) -> (x-y=w1519:dbl)
                n616 = Divide(x=w1519, y=w1516) -> (x/y=w1518:dbl)
                n617 = Multiply(x=w1518, y=w1522) -> (x*y=w1520:dbl)
                n618 = property on="X Step SP" class="DigNum (strict)"() -> ("Maximum"=w1524:dbl)  [unwired: 2 in, 2 out]
                n619 = property on="X Step SP" class="DigNum (strict)"() -> ("Minimum"=w1523:dbl)  [unwired: 2 in, 2 out]
                n620 = In Range and Coerce(upper limit=w1524, x=w1520, lower limit=w1523) -> (coerced(x)=w1521:dbl)  [unwired: 1 out]
                n621 = To Long Integer(number=w1521) -> (32bit integer=w1517:i32)
                n622 = property on="X Step SP" class="DigNum (strict)"("Val(Sgnl)"=w1517) -> ()  [unwired: 2 in, 2 out]
              }
              frame #1 {
                n623 = property on="X Step SP" class="DigNum (strict)"() -> ("Value"=w1541:i32)  [unwired: 2 in, 2 out]
                n624 = property on="X Step PV" class="DigNum (strict)"() -> ("Value"=w1540:i32)  [unwired: 2 in, 2 out]
                n625 = property on="X Backlash" class="DigNum (strict)"() -> ("Value"=w1533:i32)  [unwired: 2 in, 2 out]
                n626 = Sign(1:w1533) -> (0:w1537:i32)
                n627 = Subtract(x=w1541, y=w1540) -> (x-y=w1539:i32)
                n628 = Sign(1:w1539) -> (0:w1538:i32)
                n629 = Multiply(x=w1538, y=w1537) -> (x*y=w1536:i32)
                n630 = Equal?(x=w1536, y=1) -> (x = y?=w1534:bool)
                n631 = case shown="False" w1534 {
                  frame #0 {
                    n632 = property on="X Backlash corr" class="Bool (strict)"("Val(Sgnl)"=FALSE ("Value (Signaling)")) -> ()  [unwired: 2 in, 2 out]
                  }
                  frame #1 {
                    n633 = property on="X Backlash corr" class="Bool (strict)"("Val(Sgnl)"=TRUE ("Value (Signaling)")) -> ()  [unwired: 2 in, 2 out]
                  }
                }
              }
              frame #2 {
                # "Velocity Setting"
                n634 = property on="X Velocity SP step/sec" class="DigNum (strict)"() -> ("Value"=w1549:i32)  [unwired: 2 in, 2 out]
                n635 = Number To Decimal String(number=w1549) -> (decimal integer string=w1550:string)  [unwired: 1 in]
                n636 = call "mDrive Send Command.vi"("error in (no error)"=w1545, "Extra"=w1550, "Command"=T10."Max Velocity", "VISA resource name"=w1546) -> ("error out"=w1547:errorcluster, "VISA resource name out"=w1548:refnum<visa-resource-name>)  [unwired: 3 in, 1 out]
              }
              frame #3 {
                n637 = Wait (ms)(milliseconds to wait=u32 50) -> ()  [unwired: 1 out]
              }
              frame #4 {
                # "Move to Abs Position"
                n638 = Number To Decimal String(number=w1556) -> (decimal integer string=w1562:string)  [unwired: 1 in]
                n639 = call "mDrive Send Command.vi"("error in (no error)"=w1557, "Extra"=w1562, "Command"=T10."Move to Absolute Position", "VISA resource name"=w1558) -> ("error out"=w1559:errorcluster, "VISA resource name out"=w1560:refnum<visa-resource-name>)  [unwired: 3 in, 1 out]
              }
              frame #5 {
                n640 = Wait (ms)(milliseconds to wait=u32 50) -> ()  [unwired: 1 out]
              }
            }
          }
        }
        n641 = case shown="True" w1251 {
          tunnel: w1265 -> [w1344 w1349]
          tunnel: w1264 -> [w1345 w1348]
          tunnel: [w1345 w1347] -> w1263
          tunnel: [w1344 w1346] -> w1262
          frame #0 {
          }
          frame #1 {
            n642 = flat-sequence {
              tunnel: [w1377] -> w1363
              tunnel: [w1376] -> w1362
              tunnel: [w1364] -> w1361
              tunnel: w1348 -> [w1376]
              tunnel: w1349 -> [w1377]
              tunnel: [w1380] -> w1360
              tunnel: [w1379] -> w1359
              tunnel: [w1378] -> w1358
              tunnel: w1361 -> [w1378]
              tunnel: w1362 -> [w1379]
              tunnel: w1363 -> [w1380]
              tunnel: [w1396] -> w1357
              tunnel: [w1395] -> w1356
              tunnel: w1360 -> [w1394]
              tunnel: w1359 -> [w1393]
              tunnel: [w1392] -> w1355
              tunnel: w1358 -> [w1392]
              tunnel: w1357 -> [w1403]
              tunnel: [w1403] -> w1354
              tunnel: w1356 -> [w1402]
              tunnel: [w1402] -> w1353
              tunnel: [w1400] -> w1352
              tunnel: w1355 -> [w1400]
              tunnel: [w1408] -> w1351
              tunnel: [w1407] -> w1350
              tunnel: w1354 -> [w1406]
              tunnel: w1353 -> [w1405]
              tunnel: w1352 -> [w1404]
              tunnel: [w1411] -> w1346
              tunnel: [w1413] -> w1347
              tunnel: w1351 -> [w1413]
              tunnel: w1350 -> [w1411]
              frame #0 {
                n643 = property on="Y Position SP mm" class="DigNum (strict)"() -> ("Value"=w1370:dbl)  [unwired: 2 in, 2 out]
                n644 = property on="Y offset mm" class="DigNum (strict)"() -> ("Value"=w1371:dbl)  [unwired: 2 in, 2 out]
                n645 = property on="Y mm/rev" class="DigNum (strict)"() -> ("Value"=w1372:dbl)  [unwired: 2 in, 2 out]
                n646 = property on="Y steps/rev" class="DigNum (strict)"() -> ("Value"=w1373:u32)  [unwired: 2 in, 2 out]
                n647 = To Double Precision Float(number=w1373) -> (double precision float=w1369:dbl)
                n648 = Subtract(x=w1370, y=w1371) -> (x-y=w1366:dbl)
                n649 = Divide(x=w1366, y=w1372) -> (x/y=w1365:dbl)
                n650 = Multiply(x=w1365, y=w1369) -> (x*y=w1367:dbl)
                n651 = property on="Y Step SP" class="DigNum (strict)"() -> ("Maximum"=w1374:dbl)  [unwired: 2 in, 2 out]
                n652 = property on="Y Step SP" class="DigNum (strict)"() -> ("Minimum"=w1375:dbl)  [unwired: 2 in, 2 out]
                n653 = In Range and Coerce(upper limit=w1374, x=w1367, lower limit=w1375) -> (coerced(x)=w1368:dbl)  [unwired: 1 out]
                n654 = To Long Integer(number=w1368) -> (32bit integer=w1364:i32)
                n655 = property on="Y Step SP" class="DigNum (strict)"("Val(Sgnl)"=w1364) -> ()  [unwired: 2 in, 2 out]
              }
              frame #1 {
                n656 = property on="Y Step SP" class="DigNum (strict)"() -> ("Value"=w1389:i32)  [unwired: 2 in, 2 out]
                n657 = property on="Y Step PV" class="DigNum (strict)"() -> ("Value"=w1388:i32)  [unwired: 2 in, 2 out]
                n658 = property on="Y Backlash" class="DigNum (strict)"() -> ("Value"=w1381:i32)  [unwired: 2 in, 2 out]
                n659 = Subtract(x=w1389, y=w1388) -> (x-y=w1387:i32)
                n660 = Sign(1:w1381) -> (0:w1385:i32)
                n661 = Sign(1:w1387) -> (0:w1386:i32)
                n662 = Multiply(x=w1386, y=w1385) -> (x*y=w1384:i32)
                n663 = Equal?(x=w1384, y=1) -> (x = y?=w1382:bool)
                n664 = case shown="False" w1382 {
                  frame #0 {
                    n665 = property on="Y Backlash corr" class="Bool (strict)"("Val(Sgnl)"=FALSE ("Value (Signaling)")) -> ()  [unwired: 2 in, 2 out]
                  }
                  frame #1 {
                    n666 = property on="Y Backlash corr" class="Bool (strict)"("Val(Sgnl)"=TRUE ("Value (Signaling)")) -> ()  [unwired: 2 in, 2 out]
                  }
                }
              }
              frame #2 {
                # "Velocity Setting"
                n667 = property on="Y Velocity SP step/sec" class="DigNum (strict)"() -> ("Value"=w1397:i32)  [unwired: 2 in, 2 out]
                n668 = Number To Decimal String(number=w1397) -> (decimal integer string=w1398:string)  [unwired: 1 in]
                n669 = call "mDrive Send Command.vi"("error in (no error)"=w1394, "Extra"=w1398, "Command"=T10."Max Velocity", "VISA resource name"=w1393) -> ("error out"=w1395:errorcluster, "VISA resource name out"=w1396:refnum<visa-resource-name>)  [unwired: 3 in, 1 out]
              }
              frame #3 {
                n670 = Wait (ms)(milliseconds to wait=u32 50) -> ()  [unwired: 1 out]
              }
              frame #4 {
                # "Move to Abs Position"
                n671 = Number To Decimal String(number=w1404) -> (decimal integer string=w1410:string)  [unwired: 1 in]
                n672 = call "mDrive Send Command.vi"("error in (no error)"=w1405, "Extra"=w1410, "Command"=T10."Move to Absolute Position", "VISA resource name"=w1406) -> ("error out"=w1407:errorcluster, "VISA resource name out"=w1408:refnum<visa-resource-name>)  [unwired: 3 in, 1 out]
              }
              frame #5 {
                n673 = Wait (ms)(milliseconds to wait=u32 25) -> ()  [unwired: 1 out]
              }
            }
          }
        }
        n674 = case shown="True" w1248 {
          tunnel: w1261 -> [w1274 w1279]
          tunnel: w1260 -> [w1275 w1278]
          tunnel: [w1275 w1277] -> w1259
          tunnel: [w1274 w1276] -> w1258
          frame #0 {
          }
          frame #1 {
            n675 = flat-sequence {
              tunnel: w1278 -> [w1306]
              tunnel: w1279 -> [w1307]
              tunnel: [w1307] -> w1293
              tunnel: [w1306] -> w1292
              tunnel: [w1294] -> w1291
              tunnel: [w1310] -> w1290
              tunnel: [w1309] -> w1289
              tunnel: [w1308] -> w1288
              tunnel: w1291 -> [w1308]
              tunnel: w1292 -> [w1309]
              tunnel: w1293 -> [w1310]
              tunnel: [w1326] -> w1287
              tunnel: [w1325] -> w1286
              tunnel: w1290 -> [w1324]
              tunnel: w1289 -> [w1323]
              tunnel: [w1322] -> w1285
              tunnel: w1288 -> [w1322]
              tunnel: w1287 -> [w1333]
              tunnel: [w1333] -> w1284
              tunnel: w1286 -> [w1332]
              tunnel: [w1332] -> w1283
              tunnel: w1285 -> [w1331]
              tunnel: [w1331] -> w1282
              tunnel: [w1338] -> w1281
              tunnel: [w1337] -> w1280
              tunnel: w1284 -> [w1336]
              tunnel: w1283 -> [w1335]
              tunnel: w1282 -> [w1334]
              tunnel: [w1343] -> w1277
              tunnel: w1281 -> [w1343]
              tunnel: w1280 -> [w1342]
              tunnel: [w1342] -> w1276
              frame #0 {
                n676 = property on="R Position SP deg" class="DigNum (strict)"() -> ("Value"=w1304:dbl)  [unwired: 2 in, 2 out]
                n677 = property on="R offset deg" class="DigNum (strict)"() -> ("Value"=w1303:dbl)  [unwired: 2 in, 2 out]
                n678 = property on="R deg/rev" class="DigNum (strict)"() -> ("Value"=w1305:dbl)  [unwired: 2 in, 2 out]
                n679 = property on="R steps/rev" class="DigNum (strict)"() -> ("Value"=w1302:u32)  [unwired: 2 in, 2 out]
                n680 = To Double Precision Float(number=w1302) -> (double precision float=w1299:dbl)
                n681 = Subtract(x=w1304, y=w1303) -> (x-y=w1296:dbl)
                n682 = Divide(x=w1296, y=w1305) -> (x/y=w1295:dbl)
                n683 = Multiply(x=w1295, y=w1299) -> (x*y=w1297:dbl)
                n684 = property on="R Step SP" class="DigNum (strict)"() -> ("Maximum"=w1300:dbl)  [unwired: 2 in, 2 out]
                n685 = property on="R Step SP" class="DigNum (strict)"() -> ("Minimum"=w1301:dbl)  [unwired: 2 in, 2 out]
                n686 = In Range and Coerce(upper limit=w1300, x=w1297, lower limit=w1301) -> (coerced(x)=w1298:dbl)  [unwired: 1 out]
                n687 = To Long Integer(number=w1298) -> (32bit integer=w1294:i32)
                n688 = property on="R Step SP" class="DigNum (strict)"("Val(Sgnl)"=w1294) -> ()  [unwired: 2 in, 2 out]
              }
              frame #1 {
                n689 = property on="R Step SP" class="DigNum (strict)"() -> ("Value"=w1319:i32)  [unwired: 2 in, 2 out]
                n690 = property on="R Step PV" class="DigNum (strict)"() -> ("Value"=w1318:i32)  [unwired: 2 in, 2 out]
                n691 = property on="R Backlash" class="DigNum (strict)"() -> ("Value"=w1311:i32)  [unwired: 2 in, 2 out]
                n692 = Subtract(x=w1319, y=w1318) -> (x-y=w1317:i32)
                n693 = Sign(1:w1311) -> (0:w1315:i32)
                n694 = Sign(1:w1317) -> (0:w1316:i32)
                n695 = Multiply(x=w1316, y=w1315) -> (x*y=w1314:i32)
                n696 = Equal?(x=w1314, y=1) -> (x = y?=w1312:bool)
                n697 = case shown="False" w1312 {
                  frame #0 {
                    n698 = property on="R Backlash corr" class="Bool (strict)"("Val(Sgnl)"=FALSE ("Value (Signaling)")) -> ()  [unwired: 2 in, 2 out]
                  }
                  frame #1 {
                    n699 = property on="R Backlash corr" class="Bool (strict)"("Val(Sgnl)"=TRUE ("Value (Signaling)")) -> ()  [unwired: 2 in, 2 out]
                  }
                }
              }
              frame #2 {
                # "Velocity Setting"
                n700 = property on="R Velocity SP step/sec" class="DigNum (strict)"() -> ("Value"=w1327:i32)  [unwired: 2 in, 2 out]
                n701 = Number To Decimal String(number=w1327) -> (decimal integer string=w1328:string)  [unwired: 1 in]
                n702 = call "mDrive Send Command.vi"("error in (no error)"=w1324, "Extra"=w1328, "Command"=T10."Max Velocity", "VISA resource name"=w1323) -> ("error out"=w1325:errorcluster, "VISA resource name out"=w1326:refnum<visa-resource-name>)  [unwired: 3 in, 1 out]
              }
              frame #3 {
                n703 = Wait (ms)(milliseconds to wait=u32 50) -> ()  [unwired: 1 out]
              }
              frame #4 {
                # "Move to Abs Position"
                n704 = Number To Decimal String(number=w1334) -> (decimal integer string=w1340:string)  [unwired: 1 in]
                n705 = call "mDrive Send Command.vi"("error in (no error)"=w1335, "Extra"=w1340, "Command"=T10."Move to Absolute Position", "VISA resource name"=w1336) -> ("error out"=w1337:errorcluster, "VISA resource name out"=w1338:refnum<visa-resource-name>)  [unwired: 3 in, 1 out]
              }
              frame #5 {
                n706 = Wait (ms)(milliseconds to wait=u32 25) -> ()  [unwired: 1 out]
              }
            }
          }
        }
        n707 = property on="GO" class="Bool"("DisabledEnum"=T1."Disabled and Grayed Out" ("Disabled")) -> ()  [unwired: 2 in, 2 out]
        n708 = local write "STATUS"("MOVING" ("STATUS")) -> ()
      }
      event #3 {
        n709 = event-data() -> ()  [unwired: 1 in, 7 out]
        n710 = flat-sequence {
          tunnel: w1597 -> [w1652]
          tunnel: [w1651] -> w1591
          tunnel: w1576 -> [w1650]
          tunnel: [w1649] -> w1574
          tunnel: [w1656] -> w1592
          tunnel: w1591 -> [w1656]
          tunnel: [w1655] -> w1575
          tunnel: w1574 -> [w1655]
          tunnel: w1592 -> [w1673]
          tunnel: w1575 -> [w1670]
          tunnel: [w1669] -> w1568
          tunnel: [w1668] -> w1567
          frame #0 {
            n711 = call "mDrive Send Command.vi"("error in (no error)"=w1652, "Command"=T10."Stop", "VISA resource name"=w1650) -> ("error out"=w1651:errorcluster, "VISA resource name out"=w1649:refnum<visa-resource-name>)  [unwired: 4 in, 1 out]
          }
          frame #1 {
            n712 = Wait (ms)(milliseconds to wait=u32 50) -> ()  [unwired: 1 out]
          }
          frame #2 {
            n713 = call "mDrive Send Command.vi"("error in (no error)"=w1673, "Extra"="P", "Command"=T10."Print Parameter", "VISA resource name"=w1670) -> ("error out"=w1668:errorcluster, "read buffer"=w1663:string, "VISA resource name out"=w1669:refnum<visa-resource-name>)  [unwired: 3 in]
            n714 = property on="Z steps/rev" class="DigNum (strict)"() -> ("Value"=w1659:u32)  [unwired: 2 in, 2 out]
            n715 = Decimal String To Number(string=w1663, offset=0) -> (number=w1661:i32)  [unwired: 1 in, 1 out]
            n716 = property on="Z mm/rev" class="DigNum (strict)"() -> ("Value"=w1658:dbl)  [unwired: 2 in, 2 out]
            n717 = property on="Z Step PV" class="DigNum (strict)"("Val(Sgnl)"=w1661) -> ()  [unwired: 2 in, 2 out]
            n718 = To Double Precision Float(number=w1661) -> (double precision float=w1665:dbl)
            n719 = To Double Precision Float(number=w1659) -> (double precision float=w1664:dbl)
            n720 = property on="Z offset mm" class="DigNum (strict)"() -> ("Value"=w1657:dbl)  [unwired: 2 in, 2 out]
            n721 = Divide(x=w1665, y=w1664) -> (x/y=w1667:dbl)
            n722 = Multiply(x=w1667, y=w1658) -> (x*y=w1666:dbl)
            n723 = Add(x=w1666, y=w1657) -> (x+y=w1660:dbl)
            n724 = property on="Z Position mm PV" class="DigNum (strict)"("Val(Sgnl)"=w1660) -> ()  [unwired: 2 in, 2 out]
          }
        }
        n725 = flat-sequence {
          tunnel: w1598 -> [w1627]
          tunnel: [w1626] -> w1593
          tunnel: w1573 -> [w1625]
          tunnel: [w1624] -> w1571
          tunnel: [w1631] -> w1594
          tunnel: w1593 -> [w1631]
          tunnel: [w1630] -> w1572
          tunnel: w1571 -> [w1630]
          tunnel: w1594 -> [w1648]
          tunnel: w1572 -> [w1645]
          tunnel: [w1644] -> w1570
          tunnel: [w1643] -> w1569
          frame #0 {
            n726 = call "mDrive Send Command.vi"("error in (no error)"=w1627, "Command"=T10."Stop", "VISA resource name"=w1625) -> ("error out"=w1626:errorcluster, "VISA resource name out"=w1624:refnum<visa-resource-name>)  [unwired: 4 in, 1 out]
          }
          frame #1 {
            n727 = Wait (ms)(milliseconds to wait=u32 50) -> ()  [unwired: 1 out]
          }
          frame #2 {
            n728 = call "mDrive Send Command.vi"("error in (no error)"=w1648, "Extra"="P", "Command"=T10."Print Parameter", "VISA resource name"=w1645) -> ("error out"=w1643:errorcluster, "read buffer"=w1638:string, "VISA resource name out"=w1644:refnum<visa-resource-name>)  [unwired: 3 in]
            n729 = property on="X steps/rev" class="DigNum (strict)"() -> ("Value"=w1634:u32)  [unwired: 2 in, 2 out]
            n730 = Decimal String To Number(string=w1638, offset=0) -> (number=w1636:i32)  [unwired: 1 in, 1 out]
            n731 = property on="X mm/rev" class="DigNum (strict)"() -> ("Value"=w1633:dbl)  [unwired: 2 in, 2 out]
            n732 = property on="X Step PV" class="DigNum (strict)"("Val(Sgnl)"=w1636) -> ()  [unwired: 2 in, 2 out]
            n733 = To Double Precision Float(number=w1636) -> (double precision float=w1640:dbl)
            n734 = To Double Precision Float(number=w1634) -> (double precision float=w1639:dbl)
            n735 = property on="X offset mm" class="DigNum (strict)"() -> ("Value"=w1632:dbl)  [unwired: 2 in, 2 out]
            n736 = Divide(x=w1640, y=w1639) -> (x/y=w1642:dbl)
            n737 = Multiply(x=w1642, y=w1633) -> (x*y=w1641:dbl)
            n738 = Add(x=w1641, y=w1632) -> (x+y=w1635:dbl)
            n739 = property on="X Position mm PV" class="DigNum (strict)"("Val(Sgnl)"=w1635) -> ()  [unwired: 2 in, 2 out]
          }
        }
        n740 = flat-sequence {
          tunnel: w1596 -> [w1677]
          tunnel: [w1676] -> w1589
          tunnel: w1583 -> [w1675]
          tunnel: [w1674] -> w1581
          tunnel: [w1681] -> w1590
          tunnel: w1589 -> [w1681]
          tunnel: [w1680] -> w1582
          tunnel: w1581 -> [w1680]
          tunnel: w1590 -> [w1698]
          tunnel: w1582 -> [w1695]
          tunnel: [w1694] -> w1580
          tunnel: [w1693] -> w1579
          frame #0 {
            n741 = call "mDrive Send Command.vi"("error in (no error)"=w1677, "Command"=T10."Stop", "VISA resource name"=w1675) -> ("error out"=w1676:errorcluster, "VISA resource name out"=w1674:refnum<visa-resource-name>)  [unwired: 4 in, 1 out]
          }
          frame #1 {
            n742 = Wait (ms)(milliseconds to wait=u32 50) -> ()  [unwired: 1 out]
          }
          frame #2 {
            n743 = call "mDrive Send Command.vi"("error in (no error)"=w1698, "Extra"="P", "Command"=T10."Print Parameter", "VISA resource name"=w1695) -> ("error out"=w1693:errorcluster, "read buffer"=w1688:string, "VISA resource name out"=w1694:refnum<visa-resource-name>)  [unwired: 3 in]
            n744 = property on="Y steps/rev" class="DigNum (strict)"() -> ("Value"=w1684:u32)  [unwired: 2 in, 2 out]
            n745 = Decimal String To Number(string=w1688, offset=0) -> (number=w1685:i32)  [unwired: 1 in, 1 out]
            n746 = property on="Y mm/rev" class="DigNum (strict)"() -> ("Value"=w1683:dbl)  [unwired: 2 in, 2 out]
            n747 = To Double Precision Float(number=w1685) -> (double precision float=w1690:dbl)
            n748 = To Double Precision Float(number=w1684) -> (double precision float=w1689:dbl)
            n749 = property on="Y offset mm" class="DigNum (strict)"() -> ("Value"=w1682:dbl)  [unwired: 2 in, 2 out]
            n750 = Divide(x=w1690, y=w1689) -> (x/y=w1692:dbl)
            n751 = property on="Y Step PV" class="DigNum (strict)"("Val(Sgnl)"=w1685) -> ()  [unwired: 2 in, 2 out]
            n752 = Multiply(x=w1692, y=w1683) -> (x*y=w1691:dbl)
            n753 = Add(x=w1691, y=w1682) -> (x+y=w1686:dbl)
            n754 = property on="Y Position mm PV" class="DigNum (strict)"("Val(Sgnl)"=w1686) -> ()  [unwired: 2 in, 2 out]
          }
        }
        n755 = flat-sequence {
          tunnel: w1595 -> [w1602]
          tunnel: [w1601] -> w1587
          tunnel: w1586 -> [w1600]
          tunnel: [w1599] -> w1584
          tunnel: [w1606] -> w1588
          tunnel: w1587 -> [w1606]
          tunnel: [w1605] -> w1585
          tunnel: w1584 -> [w1605]
          tunnel: w1588 -> [w1623]
          tunnel: w1585 -> [w1620]
          tunnel: [w1619] -> w1578
          tunnel: [w1618] -> w1577
          frame #0 {
            n756 = call "mDrive Send Command.vi"("error in (no error)"=w1602, "Command"=T10."Stop", "VISA resource name"=w1600) -> ("error out"=w1601:errorcluster, "VISA resource name out"=w1599:refnum<visa-resource-name>)  [unwired: 4 in, 1 out]
          }
          frame #1 {
            n757 = Wait (ms)(milliseconds to wait=u32 50) -> ()  [unwired: 1 out]
          }
          frame #2 {
            n758 = call "mDrive Send Command.vi"("error in (no error)"=w1623, "Extra"="P", "Command"=T10."Print Parameter", "VISA resource name"=w1620) -> ("error out"=w1618:errorcluster, "read buffer"=w1613:string, "VISA resource name out"=w1619:refnum<visa-resource-name>)  [unwired: 3 in]
            n759 = property on="R steps/rev" class="DigNum (strict)"() -> ("Value"=w1611:u32)  [unwired: 2 in, 2 out]
            n760 = Decimal String To Number(string=w1613, offset=0) -> (number=w1610:i32)  [unwired: 1 in, 1 out]
            n761 = property on="R deg/rev" class="DigNum (strict)"() -> ("Value"=w1609:dbl)  [unwired: 2 in, 2 out]
            n762 = property on="R Step PV" class="DigNum (strict)"("Val(Sgnl)"=w1610) -> ()  [unwired: 2 in, 2 out]
            n763 = To Double Precision Float(number=w1610) -> (double precision float=w1615:dbl)
            n764 = To Double Precision Float(number=w1611) -> (double precision float=w1614:dbl)
            n765 = property on="R offset deg" class="DigNum (strict)"() -> ("Value"=w1608:dbl)  [unwired: 2 in, 2 out]
            n766 = Divide(x=w1615, y=w1614) -> (x/y=w1617:dbl)
            n767 = Multiply(x=w1617, y=w1609) -> (x*y=w1616:dbl)
            n768 = Add(x=w1616, y=w1608) -> (x+y=w1607:dbl)
            n769 = property on="R Position deg PV" class="DigNum (strict)"("Val(Sgnl)"=w1607) -> ()  [unwired: 2 in, 2 out]
          }
        }
        n770 = property on="GO" class="Bool"("DisabledEnum"=T1."Enabled" ("Disabled")) -> ()  [unwired: 2 in, 2 out]
      }
      event #4 {
        n771 = event-data() -> ()  [unwired: 1 in, 5 out]
        n772 = local write "STATUS"("RESSETTING" ("STATUS")) -> ()
        n773 = property on="R offset deg" class="DigNum (strict)"() -> ("Value"=w1708:dbl)  [unwired: 2 in, 2 out]
        n774 = property on="Reset Z Position mm" class="DigNum (strict)"() -> ("Value"=w1725:dbl)  [unwired: 2 in, 2 out]
        n775 = property on="Z offset mm" class="DigNum (strict)"() -> ("Value"=w1717:dbl)  [unwired: 2 in, 2 out]
        n776 = property on="Reset R Position deg" class="DigNum (strict)"() -> ("Value"=w1716:dbl)  [unwired: 2 in, 2 out]
        n777 = property on="Reset X Position mm" class="DigNum (strict)"() -> ("Value"=w1734:dbl)  [unwired: 2 in, 2 out]
        n778 = property on="X offset mm" class="DigNum (strict)"() -> ("Value"=w1726:dbl)  [unwired: 2 in, 2 out]
        n779 = property on="Reset Y Position mm" class="DigNum (strict)"() -> ("Value"=w1743:dbl)  [unwired: 2 in, 2 out]
        n780 = property on="Y offset mm" class="DigNum (strict)"() -> ("Value"=w1735:dbl)  [unwired: 2 in, 2 out]
        n781 = Subtract(x=w1725, y=w1717) -> (x-y=w1724:dbl)
        n782 = Subtract(x=w1716, y=w1708) -> (x-y=w1715:dbl)
        n783 = Subtract(x=w1734, y=w1726) -> (x-y=w1733:dbl)
        n784 = Subtract(x=w1743, y=w1735) -> (x-y=w1742:dbl)
        n785 = property on="X mm/rev" class="DigNum (strict)"() -> ("Value"=w1727:dbl)  [unwired: 2 in, 2 out]
        n786 = property on="R deg/rev" class="DigNum (strict)"() -> ("Value"=w1709:dbl)  [unwired: 2 in, 2 out]
        n787 = property on="Y mm/rev" class="DigNum (strict)"() -> ("Value"=w1736:dbl)  [unwired: 2 in, 2 out]
        n788 = property on="Z mm/rev" class="DigNum (strict)"() -> ("Value"=w1718:dbl)  [unwired: 2 in, 2 out]
        n789 = Divide(x=w1715, y=w1709) -> (x/y=w1714:dbl)
        n790 = Divide(x=w1733, y=w1727) -> (x/y=w1732:dbl)
        n791 = Divide(x=w1742, y=w1736) -> (x/y=w1741:dbl)
        n792 = Divide(x=w1724, y=w1718) -> (x/y=w1723:dbl)
        n793 = property on="R steps/rev" class="DigNum (strict)"() -> ("Value"=w1710:u32)  [unwired: 2 in, 2 out]
        n794 = property on="Z steps/rev" class="DigNum (strict)"() -> ("Value"=w1719:u32)  [unwired: 2 in, 2 out]
        n795 = property on="X steps/rev" class="DigNum (strict)"() -> ("Value"=w1728:u32)  [unwired: 2 in, 2 out]
        n796 = property on="Y steps/rev" class="DigNum (strict)"() -> ("Value"=w1737:u32)  [unwired: 2 in, 2 out]
        n797 = To Double Precision Float(number=w1719) -> (double precision float=w1722:dbl)
        n798 = To Double Precision Float(number=w1710) -> (double precision float=w1713:dbl)
        n799 = To Double Precision Float(number=w1728) -> (double precision float=w1731:dbl)
        n800 = To Double Precision Float(number=w1737) -> (double precision float=w1740:dbl)
        n801 = Multiply(x=w1723, y=w1722) -> (x*y=w1721:dbl)
        n802 = Multiply(x=w1714, y=w1713) -> (x*y=w1712:dbl)
        n803 = Multiply(x=w1732, y=w1731) -> (x*y=w1730:dbl)
        n804 = Multiply(x=w1741, y=w1740) -> (x*y=w1739:dbl)
        n805 = To Long Integer(number=w1721) -> (32bit integer=w1720:i32)
        n806 = To Long Integer(number=w1712) -> (32bit integer=w1711:i32)
        n807 = To Long Integer(number=w1730) -> (32bit integer=w1729:i32)
        n808 = To Long Integer(number=w1739) -> (32bit integer=w1738:i32)
        n809 = property on="Reset Z Motor Steps" class="DigNum (strict)"("Val(Sgnl)"=w1720) -> ()  [unwired: 2 in, 2 out]
        n810 = property on="Reset R Motor Steps" class="DigNum (strict)"("Val(Sgnl)"=w1711) -> ()  [unwired: 2 in, 2 out]
        n811 = property on="Reset X Motor Steps" class="DigNum (strict)"("Val(Sgnl)"=w1729) -> ()  [unwired: 2 in, 2 out]
        n812 = property on="Reset Y Motor Steps" class="DigNum (strict)"("Val(Sgnl)"=w1738) -> ()  [unwired: 2 in, 2 out]
      }
      event #5 {
        n813 = event-data() -> ()  [unwired: 1 in, 5 out]
        n814 = property on="Y steps/rev" class="DigNum (strict)"() -> ("Value"=w1807:u32)  [unwired: 2 in, 2 out]
        n815 = property on="Y Step SP" class="DigNum (strict)"() -> ("Value"=w1784:i32)  [unwired: 2 in, 2 out]
        n816 = property on="Y steps/rev" class="DigNum (strict)"() -> ("Value"=w1782:u32)  [unwired: 2 in, 2 out]
        n817 = property on="Y Velocity SP step/sec" class="DigNum (strict)"() -> ("Value"=w1809:i32)  [unwired: 2 in, 2 out]
        n818 = property on="Y mm/rev" class="DigNum (strict)"() -> ("Value"=w1753:dbl)  [unwired: 2 in, 2 out]
        n819 = property on="Y offset mm" class="DigNum (strict)"() -> ("Value"=w1781:dbl)  [unwired: 2 in, 2 out]
        n820 = To Double Precision Float(number=w1784) -> (double precision float=w1785:dbl)
        n821 = To Double Precision Float(number=w1782) -> (double precision float=w1788:dbl)
        n822 = To Double Precision Float(number=w1809) -> (double precision float=w1810:dbl)
        n823 = To Double Precision Float(number=w1807) -> (double precision float=w1812:dbl)
        n824 = Divide(x=w1785, y=w1788) -> (x/y=w1787:dbl)
        n825 = Divide(x=w1810, y=w1812) -> (x/y=w1811:dbl)
        n826 = Multiply(x=w1787, y=w1753) -> (x*y=w1786:dbl)
        n827 = Multiply(x=w1811, y=w1753) -> (x*y=w1808:dbl)
        n828 = Add(x=w1786, y=w1781) -> (x+y=w1783:dbl)
        n829 = property on="Y Velocity MV mm/sec" class="DigNum (strict)"("Val(Sgnl)"=w1808) -> ()  [unwired: 2 in, 2 out]
        n830 = property on="Y Position MV mm" class="DigNum (strict)"("Val(Sgnl)"=w1783) -> ()  [unwired: 2 in, 2 out]
        n831 = property on="Z steps/rev" class="DigNum (strict)"() -> ("Value"=w1795:u32)  [unwired: 2 in, 2 out]
        n832 = property on="Z Step SP" class="DigNum (strict)"() -> ("Value"=w1768:i32)  [unwired: 2 in, 2 out]
        n833 = property on="Z steps/rev" class="DigNum (strict)"() -> ("Value"=w1766:u32)  [unwired: 2 in, 2 out]
        n834 = property on="Z Velocity SP step/sec" class="DigNum (strict)"() -> ("Value"=w1797:i32)  [unwired: 2 in, 2 out]
        n835 = property on="Z mm/rev" class="DigNum (strict)"() -> ("Value"=w1755:dbl)  [unwired: 2 in, 2 out]
        n836 = property on="Z offset mm" class="DigNum (strict)"() -> ("Value"=w1765:dbl)  [unwired: 2 in, 2 out]
        n837 = To Double Precision Float(number=w1797) -> (double precision float=w1798:dbl)
        n838 = To Double Precision Float(number=w1795) -> (double precision float=w1800:dbl)
        n839 = To Double Precision Float(number=w1768) -> (double precision float=w1769:dbl)
        n840 = To Double Precision Float(number=w1766) -> (double precision float=w1772:dbl)
        n841 = Divide(x=w1769, y=w1772) -> (x/y=w1771:dbl)
        n842 = Divide(x=w1798, y=w1800) -> (x/y=w1799:dbl)
        n843 = Multiply(x=w1771, y=w1755) -> (x*y=w1770:dbl)
        n844 = Multiply(x=w1799, y=w1755) -> (x*y=w1796:dbl)
        n845 = Add(x=w1770, y=w1765) -> (x+y=w1767:dbl)
        n846 = property on="Z Velocity MV mm/sec" class="DigNum (strict)"("Val(Sgnl)"=w1796) -> ()  [unwired: 2 in, 2 out]
        n847 = property on="Z Position MV mm" class="DigNum (strict)"("Val(Sgnl)"=w1767) -> ()  [unwired: 2 in, 2 out]
        n848 = property on="X Velocity SP step/sec" class="DigNum (strict)"() -> ("Value"=w1803:i32)  [unwired: 2 in, 2 out]
        n849 = property on="X steps/rev" class="DigNum (strict)"() -> ("Value"=w1801:u32)  [unwired: 2 in, 2 out]
        n850 = property on="X Step SP" class="DigNum (strict)"() -> ("Value"=w1776:i32)  [unwired: 2 in, 2 out]
        n851 = property on="X steps/rev" class="DigNum (strict)"() -> ("Value"=w1774:u32)  [unwired: 2 in, 2 out]
        n852 = property on="X offset mm" class="DigNum (strict)"() -> ("Value"=w1773:dbl)  [unwired: 2 in, 2 out]
        n853 = property on="X mm/rev" class="DigNum (strict)"() -> ("Value"=w1754:dbl)  [unwired: 2 in, 2 out]
        n854 = To Double Precision Float(number=w1776) -> (double precision float=w1777:dbl)
        n855 = To Double Precision Float(number=w1774) -> (double precision float=w1780:dbl)
        n856 = To Double Precision Float(number=w1803) -> (double precision float=w1804:dbl)
        n857 = To Double Precision Float(number=w1801) -> (double precision float=w1806:dbl)
        n858 = Divide(x=w1777, y=w1780) -> (x/y=w1779:dbl)
        n859 = Divide(x=w1804, y=w1806) -> (x/y=w1805:dbl)
        n860 = Multiply(x=w1779, y=w1754) -> (x*y=w1778:dbl)
        n861 = Add(x=w1778, y=w1773) -> (x+y=w1775:dbl)
        n862 = Multiply(x=w1805, y=w1754) -> (x*y=w1802:dbl)
        n863 = property on="X Velocity MV mm/sec" class="DigNum (strict)"("Val(Sgnl)"=w1802) -> ()  [unwired: 2 in, 2 out]
        n864 = property on="X Position MV mm" class="DigNum (strict)"("Val(Sgnl)"=w1775) -> ()  [unwired: 2 in, 2 out]
        n865 = property on="R steps/rev" class="DigNum (strict)"() -> ("Value"=w1789:u32)  [unwired: 2 in, 2 out]
        n866 = property on="R Step SP" class="DigNum (strict)"() -> ("Value"=w1760:i32)  [unwired: 2 in, 2 out]
        n867 = property on="R steps/rev" class="DigNum (strict)"() -> ("Value"=w1758:u32)  [unwired: 2 in, 2 out]
        n868 = property on="R deg/rev" class="DigNum (strict)"() -> ("Value"=w1756:dbl)  [unwired: 2 in, 2 out]
        n869 = property on="R offset deg" class="DigNum (strict)"() -> ("Value"=w1757:dbl)  [unwired: 2 in, 2 out]
        n870 = property on="R Velocity SP step/sec" class="DigNum (strict)"() -> ("Value"=w1791:i32)  [unwired: 2 in, 2 out]
        n871 = To Double Precision Float(number=w1760) -> (double precision float=w1761:dbl)
        n872 = To Double Precision Float(number=w1758) -> (double precision float=w1764:dbl)
        n873 = To Double Precision Float(number=w1789) -> (double precision float=w1794:dbl)
        n874 = To Double Precision Float(number=w1791) -> (double precision float=w1792:dbl)
        n875 = Divide(x=w1761, y=w1764) -> (x/y=w1763:dbl)
        n876 = Divide(x=w1792, y=w1794) -> (x/y=w1793:dbl)
        n877 = Multiply(x=w1763, y=w1756) -> (x*y=w1762:dbl)
        n878 = Multiply(x=w1793, y=w1756) -> (x*y=w1790:dbl)
        n879 = Add(x=w1762, y=w1757) -> (x+y=w1759:dbl)
        n880 = Absolute Value(x=w1790) -> (abs(x)=w1752:dbl)
        n881 = property on="R Position MV deg" class="DigNum (strict)"("Val(Sgnl)"=w1759) -> ()  [unwired: 2 in, 2 out]
        n882 = property on="R Velocity MVdeg/sec" class="DigNum (strict)"("Val(Sgnl)"=w1752) -> ()  [unwired: 2 in, 2 out]
      }
      event #6 {
        n883 = event-data() -> ()  [unwired: 1 in, 5 out]
        n884 = property on="R Step PV" class="DigNum (strict)"() -> ("Value"=w1853:i32)  [unwired: 2 in, 2 out]
        n885 = property on="R Step SP" class="DigNum (strict)"() -> ("Maximum"=w1861:dbl)  [unwired: 2 in, 2 out]
        n886 = property on="R Step SP" class="DigNum (strict)"() -> ("Minimum"=w1858:dbl)  [unwired: 2 in, 2 out]
        n887 = property on="X Step PV" class="DigNum (strict)"() -> ("Value"=w1893:i32)  [unwired: 2 in, 2 out]
        n888 = property on="Z Step PV" class="DigNum (strict)"() -> ("Value"=w1867:i32)  [unwired: 2 in, 2 out]
        n889 = property on="Z Step SP" class="DigNum (strict)"() -> ("Minimum"=w1874:dbl)  [unwired: 2 in, 2 out]
        n890 = property on="Z Step SP" class="DigNum (strict)"() -> ("Maximum"=w1873:dbl)  [unwired: 2 in, 2 out]
        n891 = property on="X Step SP" class="DigNum (strict)"() -> ("Maximum"=w1897:dbl)  [unwired: 2 in, 2 out]
        n892 = property on="Y Step SP" class="DigNum (strict)"() -> ("Minimum"=w1887:dbl)  [unwired: 2 in, 2 out]
        n893 = property on="Y Step SP" class="DigNum (strict)"() -> ("Maximum"=w1886:dbl)  [unwired: 2 in, 2 out]
        n894 = property on="X Step SP" class="DigNum (strict)"() -> ("Minimum"=w1898:dbl)  [unwired: 2 in, 2 out]
        n895 = property on="Y Step PV" class="DigNum (strict)"() -> ("Value"=w1880:i32)  [unwired: 2 in, 2 out]
        n896 = To Double Precision Float(number=w1853) -> (double precision float=w1844:dbl)
        n897 = To Double Precision Float(number=w1893) -> (double precision float=w1847:dbl)
        n898 = To Double Precision Float(number=w1867) -> (double precision float=w1845:dbl)
        n899 = To Double Precision Float(number=w1880) -> (double precision float=w1846:dbl)
        n900 = Subtract(x=w1858, y=w1844) -> (x-y=w1859:dbl)
        n901 = Subtract(x=w1861, y=w1844) -> (x-y=w1860:dbl)
        n902 = Subtract(x=w1887, y=w1846) -> (x-y=w1888:dbl)
        n903 = Subtract(x=w1886, y=w1846) -> (x-y=w1885:dbl)
        n904 = Subtract(x=w1898, y=w1847) -> (x-y=w1899:dbl)
        n905 = Subtract(x=w1897, y=w1847) -> (x-y=w1896:dbl)
        n906 = Subtract(x=w1874, y=w1845) -> (x-y=w1875:dbl)
        n907 = Subtract(x=w1873, y=w1845) -> (x-y=w1872:dbl)
        n908 = property on="R Scan Length SP steps" class="DigNum (strict)"("Minimum"=w1859) -> ()  [unwired: 2 in, 2 out]
        n909 = property on="R Scan Length SP steps" class="DigNum (strict)"("Maximum"=w1860) -> ()  [unwired: 2 in, 2 out]
        n910 = property on="Y Scan Length SP steps" class="DigNum (strict)"("Minimum"=w1888) -> ()  [unwired: 2 in, 2 out]
        n911 = property on="Y Scan Length SP steps" class="DigNum (strict)"("Maximum"=w1885) -> ()  [unwired: 2 in, 2 out]
        n912 = property on="X Scan Length SP steps" class="DigNum (strict)"("Minimum"=w1899) -> ()  [unwired: 2 in, 2 out]
        n913 = property on="X Scan Length SP steps" class="DigNum (strict)"("Maximum"=w1896) -> ()  [unwired: 2 in, 2 out]
        n914 = property on="Z Scan Length SP steps" class="DigNum (strict)"("Minimum"=w1875) -> ()  [unwired: 2 in, 2 out]
        n915 = property on="Z Scan Length SP steps" class="DigNum (strict)"("Maximum"=w1872) -> ()  [unwired: 2 in, 2 out]
        n916 = property on="X steps/rev" class="DigNum (strict)"() -> ("Value"=w1894:u32)  [unwired: 2 in, 2 out]
        n917 = property on="X Scan Length SP steps" class="DigNum (strict)"() -> ("Value"=w1891:i32)  [unwired: 2 in, 2 out]
        n918 = property on="X Scan Velocity SP steps/sec" class="DigNum (strict)"() -> ("Value"=w1895:i32)  [unwired: 2 in, 2 out]
        n919 = property on="Y steps/rev" class="DigNum (strict)"() -> ("Value"=w1882:u32)  [unwired: 2 in, 2 out]
        n920 = property on="R Scan Length SP steps" class="DigNum (strict)"() -> ("Value"=w1856:i32)  [unwired: 2 in, 2 out]
        n921 = property on="R steps/rev" class="DigNum (strict)"() -> ("Value"=w1855:u32)  [unwired: 2 in, 2 out]
        n922 = property on="R Scan Velocity SP steps/sec" class="DigNum (strict)"() -> ("Value"=w1851:i32)  [unwired: 2 in, 2 out]
        n923 = property on="Y Scan Length SP steps" class="DigNum (strict)"() -> ("Value"=w1883:i32)  [unwired: 2 in, 2 out]
        n924 = property on="Y Scan Velocity SP steps/sec" class="DigNum (strict)"() -> ("Value"=w1879:i32)  [unwired: 2 in, 2 out]
        n925 = property on="Z Scan Length SP steps" class="DigNum (strict)"() -> ("Value"=w1870:i32)  [unwired: 2 in, 2 out]
        n926 = property on="Z steps/rev" class="DigNum (strict)"() -> ("Value"=w1869:u32)  [unwired: 2 in, 2 out]
        n927 = property on="Z Scan Velocity SP steps/sec" class="DigNum (strict)"() -> ("Value"=w1865:i32)  [unwired: 2 in, 2 out]
        n928 = To Double Precision Float(number=w1891) -> (double precision float=w1834:dbl)
        n929 = To Double Precision Float(number=w1894) -> (double precision float=w1892:dbl)
        n930 = To Double Precision Float(number=w1895) -> (double precision float=w1833:dbl)
        n931 = To Double Precision Float(number=w1856) -> (double precision float=w1841:dbl)
        n932 = To Double Precision Float(number=w1855) -> (double precision float=w1852:dbl)
        n933 = To Double Precision Float(number=w1851) -> (double precision float=w1840:dbl)
        n934 = To Double Precision Float(number=w1870) -> (double precision float=w1843:dbl)
        n935 = To Double Precision Float(number=w1869) -> (double precision float=w1866:dbl)
        n936 = To Double Precision Float(number=w1865) -> (double precision float=w1842:dbl)
        n937 = To Double Precision Float(number=w1883) -> (double precision float=w1836:dbl)
        n938 = To Double Precision Float(number=w1882) -> (double precision float=w1837:dbl)
        n939 = To Double Precision Float(number=w1879) -> (double precision float=w1835:dbl)
        n940 = property on="R deg/rev" class="DigNum (strict)"() -> ("Value"=w1854:dbl)  [unwired: 2 in, 2 out]
        n941 = Divide(x=w1841, y=w1852) -> (x/y=w1857:dbl)
        n942 = property on="Z mm/rev" class="DigNum (strict)"() -> ("Value"=w1868:dbl)  [unwired: 2 in, 2 out]
        n943 = property on="X mm/rev" class="DigNum (strict)"() -> ("Value"=w1820:dbl)  [unwired: 2 in, 2 out]
        n944 = Divide(x=w1834, y=w1892) -> (x/y=w1821:dbl)
        n945 = Divide(x=w1843, y=w1866) -> (x/y=w1871:dbl)
        n946 = property on="Y mm/rev" class="DigNum (strict)"() -> ("Value"=w1881:dbl)  [unwired: 2 in, 2 out]
        n947 = Divide(x=w1836, y=w1837) -> (x/y=w1884:dbl)
        n948 = Divide(x=w1842, y=w1866) -> (x/y=w1864:dbl)
        n949 = Divide(x=w1840, y=w1852) -> (x/y=w1850:dbl)
        n950 = Multiply(x=w1871, y=w1868) -> (x*y=w1863:dbl)
        n951 = Divide(x=w1835, y=w1837) -> (x/y=w1878:dbl)
        n952 = Divide(x=w1833, y=w1892) -> (x/y=w1819:dbl)
        n953 = Multiply(x=w1821, y=w1820) -> (x*y=w1889:dbl)
        n954 = Divide(x=w1843, y=w1842) -> (x/y=w1838:dbl)
        n955 = Multiply(x=w1868, y=w1864) -> (x*y=w1862:dbl)
        n956 = Absolute Value(x=w1838) -> (abs(x)=→"Z Scan Duration":dbl)
        n957 = Multiply(x=w1884, y=w1881) -> (x*y=w1877:dbl)
        n958 = Multiply(x=w1881, y=w1878) -> (x*y=w1876:dbl)
        n959 = Multiply(x=w1820, y=w1819) -> (x*y=w1890:dbl)
        n960 = Divide(x=w1841, y=w1840) -> (x/y=w1839:dbl)
        n961 = Multiply(x=w1857, y=w1854) -> (x*y=w1849:dbl)
        n962 = Multiply(x=w1854, y=w1850) -> (x*y=w1848:dbl)
        n963 = Absolute Value(x=w1839) -> (abs(x)=→"R Scan Duration":dbl)
        n964 = Absolute Value(x=w1848) -> (abs(x)=w1832:dbl)
        n965 = property on="Z Scan length MV mm" class="DigNum (strict)"("Value"=w1863) -> ()  [unwired: 2 in, 2 out]
        n966 = property on="Z Scan velocity MV mm/sec" class="DigNum (strict)"("Val(Sgnl)"=w1862) -> ()  [unwired: 2 in, 2 out]
        n967 = property on="X Scan length MV mm" class="DigNum (strict)"("Val(Sgnl)"=w1889) -> ()  [unwired: 2 in, 2 out]
        n968 = property on="X Scan velocity MV mm/sec" class="DigNum (strict)"("Value"=w1890) -> ()  [unwired: 2 in, 2 out]
        n969 = property on="Y Scan length MV mm" class="DigNum (strict)"("Value"=w1877) -> ()  [unwired: 2 in, 2 out]
        n970 = property on="Y Scan velocity MV mm/sec" class="DigNum (strict)"("Val(Sgnl)"=w1876) -> ()  [unwired: 2 in, 2 out]
        n971 = property on="R Scan length MV deg" class="DigNum (strict)"("Value"=w1849) -> ()  [unwired: 2 in, 2 out]
        n972 = property on="R Scan Velocity SP deg/sec" class="DigNum (strict)"("Val(Sgnl)"=w1832) -> ()  [unwired: 2 in, 2 out]
        n973 = property on="Y Scan Length SP mm" class="DigNum (strict)"() -> ("Value"=w1816:dbl)  [unwired: 2 in, 2 out]
        n974 = property on="X Scan Length SP mm" class="DigNum (strict)"() -> ("Value"=w1815:dbl)  [unwired: 2 in, 2 out]
        n975 = Equal?(x=w1816, y=0.0) -> (x = y?=w1814:bool)
        n976 = Equal?(x=w1815, y=0.0) -> (x = y?=w1813:bool)
        n977 = case shown="True" w1814 {
          tunnel: w1836 -> [w1908 _]
          tunnel: w1835 -> [w1907 _]
          frame #0 {
            n978 = Divide(x=w1908, y=w1907) -> (x/y=w1906:dbl)
            n979 = Absolute Value(x=w1906) -> (abs(x)=→"Y Scan Duration":dbl)
          }
          frame #1 {
            n980 = local write "Y Scan Duration"(0.0 ("Y Scan Duration")) -> ()
          }
        }
        n981 = case shown="True" w1813 {
          tunnel: w1834 -> [w1902 _]
          tunnel: w1833 -> [w1901 _]
          frame #0 {
            n982 = Divide(x=w1902, y=w1901) -> (x/y=w1903:dbl)
            n983 = Absolute Value(x=w1903) -> (abs(x)=→"X Scan Duration":dbl)
          }
          frame #1 {
            n984 = local write "X Scan Duration"(0.0 ("X Scan Duration")) -> ()
          }
        }
      }
      event #7 {
        n985 = event-data() -> ()  [unwired: 1 in, 7 out]
        n986 = Wait (ms)(milliseconds to wait=u32 100) -> ()  [unwired: 1 out]
        n987 = local write "STATUS"("SETTING Y" ("STATUS")) -> ()
        n988 = property on="Y Position SP mm" class="DigNum (strict)"() -> ("Value"=w1933:dbl)  [unwired: 2 in, 2 out]
        n989 = property on="Y offset mm" class="DigNum (strict)"() -> ("Value"=w1934:dbl)  [unwired: 2 in, 2 out]
        n990 = property on="Y mm/rev" class="DigNum (strict)"() -> ("Value"=w1920:dbl)  [unwired: 2 in, 2 out]
        n991 = property on="Y Velocity SP mm/sec" class="DigNum (strict)"() -> ("Value"=w1927:dbl)  [unwired: 2 in, 2 out]
        n992 = property on="Y steps/rev" class="DigNum (strict)"() -> ("Value"=w1936:u32)  [unwired: 2 in, 2 out]
        n993 = Subtract(x=w1933, y=w1934) -> (x-y=w1937:dbl)
        n994 = Divide(x=w1927, y=w1920) -> (x/y=w1928:dbl)
        n995 = To Double Precision Float(number=w1936) -> (double precision float=w1921:dbl)
        n996 = Divide(x=w1937, y=w1920) -> (x/y=w1938:dbl)
        n997 = Multiply(x=w1928, y=w1921) -> (x*y=w1925:dbl)
        n998 = property on="Y Velocity SP step/sec" class="DigNum (strict)"() -> ("Maximum"=w1923:dbl)  [unwired: 2 in, 2 out]
        n999 = property on="Y Velocity SP step/sec" class="DigNum (strict)"() -> ("Minimum"=w1922:dbl)  [unwired: 2 in, 2 out]
        n1000 = Multiply(x=w1938, y=w1921) -> (x*y=w1932:dbl)
        n1001 = In Range and Coerce(upper limit=w1923, x=w1925, lower limit=w1922) -> (coerced(x)=w1924:dbl)  [unwired: 1 out]
        n1002 = property on="Y Step SP" class="DigNum (strict)"() -> ("Maximum"=w1930:dbl)  [unwired: 2 in, 2 out]
        n1003 = property on="Y Step SP" class="DigNum (strict)"() -> ("Minimum"=w1929:dbl)  [unwired: 2 in, 2 out]
        n1004 = To Long Integer(number=w1924) -> (32bit integer=w1926:i32)
        n1005 = property on="Y Velocity SP step/sec" class="DigNum (strict)"("Val(Sgnl)"=w1926) -> ()  [unwired: 2 in, 2 out]
        n1006 = In Range and Coerce(upper limit=w1930, x=w1932, lower limit=w1929) -> (coerced(x)=w1931:dbl)  [unwired: 1 out]
        n1007 = To Long Integer(number=w1931) -> (32bit integer=w1935:i32)
        n1008 = property on="Y Step SP" class="DigNum (strict)"("Val(Sgnl)"=w1935) -> ()  [unwired: 2 in, 2 out]
      }
      event #8 {
        n1009 = event-data() -> ()  [unwired: 1 in, 7 out]
        n1010 = Wait (ms)(milliseconds to wait=u32 100) -> ()  [unwired: 1 out]
        n1011 = property on="X Position SP mm" class="DigNum (strict)"() -> ("Value"=w1962:dbl)  [unwired: 2 in, 2 out]
        n1012 = property on="X offset mm" class="DigNum (strict)"() -> ("Value"=w1963:dbl)  [unwired: 2 in, 2 out]
        n1013 = property on="X steps/rev" class="DigNum (strict)"() -> ("Value"=w1965:u32)  [unwired: 2 in, 2 out]
        n1014 = property on="X Velocity SP mm/sec" class="DigNum (strict)"() -> ("Value"=w1956:dbl)  [unwired: 2 in, 2 out]
        n1015 = property on="X mm/rev" class="DigNum (strict)"() -> ("Value"=w1949:dbl)  [unwired: 2 in, 2 out]
        n1016 = Subtract(x=w1962, y=w1963) -> (x-y=w1966:dbl)
        n1017 = Divide(x=w1956, y=w1949) -> (x/y=w1957:dbl)
        n1018 = To Double Precision Float(number=w1965) -> (double precision float=w1950:dbl)
        n1019 = local write "STATUS"("SETTING X" ("STATUS")) -> ()
        n1020 = Divide(x=w1966, y=w1949) -> (x/y=w1967:dbl)
        n1021 = Multiply(x=w1957, y=w1950) -> (x*y=w1954:dbl)
        n1022 = property on="X Velocity SP step/sec" class="DigNum (strict)"() -> ("Maximum"=w1952:dbl)  [unwired: 2 in, 2 out]
        n1023 = property on="X Velocity SP step/sec" class="DigNum (strict)"() -> ("Minimum"=w1951:dbl)  [unwired: 2 in, 2 out]
        n1024 = Multiply(x=w1967, y=w1950) -> (x*y=w1961:dbl)
        n1025 = property on="X Step SP" class="DigNum (strict)"() -> ("Maximum"=w1959:dbl)  [unwired: 2 in, 2 out]
        n1026 = property on="X Step SP" class="DigNum (strict)"() -> ("Minimum"=w1958:dbl)  [unwired: 2 in, 2 out]
        n1027 = In Range and Coerce(upper limit=w1952, x=w1954, lower limit=w1951) -> (coerced(x)=w1953:dbl)  [unwired: 1 out]
        n1028 = To Long Integer(number=w1953) -> (32bit integer=w1955:i32)
        n1029 = In Range and Coerce(upper limit=w1959, x=w1961, lower limit=w1958) -> (coerced(x)=w1960:dbl)  [unwired: 1 out]
        n1030 = property on="X Velocity SP step/sec" class="DigNum (strict)"("Val(Sgnl)"=w1955) -> ()  [unwired: 2 in, 2 out]
        n1031 = To Long Integer(number=w1960) -> (32bit integer=w1964:i32)
        n1032 = property on="X Step SP" class="DigNum (strict)"("Val(Sgnl)"=w1964) -> ()  [unwired: 2 in, 2 out]
      }
      event #9 {
        n1033 = event-data() -> ()  [unwired: 1 in, 7 out]
        n1034 = Wait (ms)(milliseconds to wait=u32 100) -> ()  [unwired: 1 out]
        n1035 = property on="Z mm/rev" class="DigNum (strict)"() -> ("Value"=w1995:dbl)  [unwired: 2 in, 2 out]
        n1036 = property on="Z steps/rev" class="DigNum (strict)"() -> ("Value"=w1992:u32)  [unwired: 2 in, 2 out]
        n1037 = property on="Z Velocity SP mm/sec" class="DigNum (strict)"() -> ("Value"=w1983:dbl)  [unwired: 2 in, 2 out]
        n1038 = property on="Z Position SP mm" class="DigNum (strict)"() -> ("Value"=w1989:dbl)  [unwired: 2 in, 2 out]
        n1039 = property on="Z offset mm" class="DigNum (strict)"() -> ("Value"=w1990:dbl)  [unwired: 2 in, 2 out]
        n1040 = Divide(x=w1983, y=w1995) -> (x/y=w1984:dbl)
        n1041 = To Double Precision Float(number=w1992) -> (double precision float=w1996:dbl)
        n1042 = Subtract(x=w1989, y=w1990) -> (x-y=w1993:dbl)
        n1043 = Divide(x=w1993, y=w1995) -> (x/y=w1994:dbl)
        n1044 = Multiply(x=w1984, y=w1996) -> (x*y=w1981:dbl)
        n1045 = property on="Z Velocity SP step/sec" class="DigNum (strict)"() -> ("Maximum"=w1979:dbl)  [unwired: 2 in, 2 out]
        n1046 = property on="Z Velocity SP step/sec" class="DigNum (strict)"() -> ("Minimum"=w1978:dbl)  [unwired: 2 in, 2 out]
        n1047 = local write "STATUS"("SETTING Z" ("STATUS")) -> ()
        n1048 = Multiply(x=w1994, y=w1996) -> (x*y=w1988:dbl)
        n1049 = In Range and Coerce(upper limit=w1979, x=w1981, lower limit=w1978) -> (coerced(x)=w1980:dbl)  [unwired: 1 out]
        n1050 = property on="Z Step SP" class="DigNum (strict)"() -> ("Maximum"=w1986:dbl)  [unwired: 2 in, 2 out]
        n1051 = property on="Z Step SP" class="DigNum (strict)"() -> ("Minimum"=w1985:dbl)  [unwired: 2 in, 2 out]
        n1052 = To Long Integer(number=w1980) -> (32bit integer=w1982:i32)
        n1053 = property on="Z Velocity SP step/sec" class="DigNum (strict)"("Val(Sgnl)"=w1982) -> ()  [unwired: 2 in, 2 out]
        n1054 = In Range and Coerce(upper limit=w1986, x=w1988, lower limit=w1985) -> (coerced(x)=w1987:dbl)  [unwired: 1 out]
        n1055 = To Long Integer(number=w1987) -> (32bit integer=w1991:i32)
        n1056 = property on="Z Step SP" class="DigNum (strict)"("Val(Sgnl)"=w1991) -> ()  [unwired: 2 in, 2 out]
      }
      event #10 {
        n1057 = event-data() -> ()  [unwired: 1 in, 7 out]
        n1058 = property on="R offset deg" class="DigNum (strict)"() -> ("Value"=w2022:dbl)  [unwired: 2 in, 2 out]
        n1059 = property on="R Position SP deg" class="DigNum (strict)"() -> ("Value"=w2021:dbl)  [unwired: 2 in, 2 out]
        n1060 = Wait (ms)(milliseconds to wait=u32 100) -> ()  [unwired: 1 out]
        n1061 = Subtract(x=w2021, y=w2022) -> (x-y=w2025:dbl)
        n1062 = property on="R deg/rev" class="DigNum (strict)"() -> ("Value"=w2008:dbl)  [unwired: 2 in, 2 out]
        n1063 = property on="R Velocity SP deg/sec" class="DigNum (strict)"() -> ("Value"=w2015:dbl)  [unwired: 2 in, 2 out]
        n1064 = Divide(x=w2025, y=w2008) -> (x/y=w2026:dbl)
        n1065 = property on="R steps/rev" class="DigNum (strict)"() -> ("Value"=w2024:u32)  [unwired: 2 in, 2 out]
        n1066 = Divide(x=w2015, y=w2008) -> (x/y=w2016:dbl)
        n1067 = To Double Precision Float(number=w2024) -> (double precision float=w2009:dbl)
        n1068 = Multiply(x=w2016, y=w2009) -> (x*y=w2013:dbl)
        n1069 = Multiply(x=w2026, y=w2009) -> (x*y=w2020:dbl)
        n1070 = property on="R Velocity SP step/sec" class="DigNum (strict)"() -> ("Maximum"=w2011:dbl)  [unwired: 2 in, 2 out]
        n1071 = property on="R Step SP" class="DigNum (strict)"() -> ("Maximum"=w2018:dbl)  [unwired: 2 in, 2 out]
        n1072 = property on="R Step SP" class="DigNum (strict)"() -> ("Minimum"=w2017:dbl)  [unwired: 2 in, 2 out]
        n1073 = property on="R Velocity SP step/sec" class="DigNum (strict)"() -> ("Minimum"=w2010:dbl)  [unwired: 2 in, 2 out]
        n1074 = Absolute Value(x=w2013) -> (abs(x)=w2007:dbl)
        n1075 = In Range and Coerce(upper limit=w2018, x=w2020, lower limit=w2017) -> (coerced(x)=w2019:dbl)  [unwired: 1 out]
        n1076 = In Range and Coerce(upper limit=w2011, x=w2007, lower limit=w2010) -> (coerced(x)=w2012:dbl)  [unwired: 1 out]
        n1077 = To Long Integer(number=w2019) -> (32bit integer=w2023:i32)
        n1078 = To Long Integer(number=w2012) -> (32bit integer=w2014:i32)
        n1079 = local write "STATUS"("SETTING R" ("STATUS")) -> ()
        n1080 = property on="R Step SP" class="DigNum (strict)"("Val(Sgnl)"=w2023) -> ()  [unwired: 2 in, 2 out]
        n1081 = property on="R Velocity SP step/sec" class="DigNum (strict)"("Val(Sgnl)"=w2014) -> ()  [unwired: 2 in, 2 out]
      }
      event #11 {
        n1082 = event-data() -> ()  [unwired: 1 in, 7 out]
        n1083 = flat-sequence {
          frame #0 {
            n1084 = property on="Y mm/rev" class="DigNum (strict)"() -> ("Value"=w2036:dbl)  [unwired: 2 in, 2 out]
            n1085 = property on="Z mm/rev" class="DigNum (strict)"() -> ("Value"=w2088:dbl)  [unwired: 2 in, 2 out]
            n1086 = property on="Z Scan Length SP mm" class="DigNum (strict)"() -> ("Value"=w2101:dbl)  [unwired: 2 in, 2 out]
            n1087 = property on="Y Scan Length SP mm" class="DigNum (strict)"() -> ("Value"=w2049:dbl)  [unwired: 2 in, 2 out]
            n1088 = property on="Y steps/rev" class="DigNum (strict)"() -> ("Value"=w2051:u32)  [unwired: 2 in, 2 out]
            n1089 = Divide(x=w2101, y=w2088) -> (x/y=w2104:dbl)
            n1090 = Divide(x=w2049, y=w2036) -> (x/y=w2052:dbl)
            n1091 = property on="Z steps/rev" class="DigNum (strict)"() -> ("Value"=w2103:u32)  [unwired: 2 in, 2 out]
            n1092 = To Double Precision Float(number=w2051) -> (double precision float=w2037:dbl)
            n1093 = To Double Precision Float(number=w2103) -> (double precision float=w2089:dbl)
            n1094 = Multiply(x=w2052, y=w2037) -> (x*y=w2048:dbl)
            n1095 = property on="Y Step SP" class="DigNum (strict)"() -> ("Minimum"=w2046:dbl)  [unwired: 2 in, 2 out]
            n1096 = property on="Y Step SP" class="DigNum (strict)"() -> ("Maximum"=w2045:dbl)  [unwired: 2 in, 2 out]
            n1097 = property on="Z Step SP" class="DigNum (strict)"() -> ("Maximum"=w2097:dbl)  [unwired: 2 in, 2 out]
            n1098 = property on="Z Step SP" class="DigNum (strict)"() -> ("Minimum"=w2098:dbl)  [unwired: 2 in, 2 out]
            n1099 = Multiply(x=w2104, y=w2089) -> (x*y=w2100:dbl)
            n1100 = In Range and Coerce(upper limit=w2045, x=w2048, lower limit=w2046) -> (coerced(x)=w2047:dbl)  [unwired: 1 out]
            n1101 = In Range and Coerce(upper limit=w2097, x=w2100, lower limit=w2098) -> (coerced(x)=w2099:dbl)  [unwired: 1 out]
            n1102 = To Long Integer(number=w2047) -> (32bit integer=w2050:i32)
            n1103 = property on="Y Scan Velocity SP mm/sec" class="DigNum (strict)"() -> ("Value"=w2043:dbl)  [unwired: 2 in, 2 out]
            n1104 = property on="Z Scan Velocity SP mm/sec" class="DigNum (strict)"() -> ("Value"=w2095:dbl)  [unwired: 2 in, 2 out]
            n1105 = To Long Integer(number=w2099) -> (32bit integer=w2102:i32)
            n1106 = Divide(x=w2043, y=w2036) -> (x/y=w2044:dbl)
            n1107 = property on="Y Scan Length SP steps" class="DigNum (strict)"("Val(Sgnl)"=w2050) -> ()  [unwired: 2 in, 2 out]
            n1108 = property on="Y Scan Velocity SP steps/sec" class="DigNum (strict)"() -> ("Maximum"=w2039:dbl)  [unwired: 2 in, 2 out]
            n1109 = property on="Z Scan Velocity SP steps/sec" class="DigNum (strict)"() -> ("Maximum"=w2091:dbl)  [unwired: 2 in, 2 out]
            n1110 = Divide(x=w2095, y=w2088) -> (x/y=w2096:dbl)
            n1111 = property on="Y Scan Velocity SP steps/sec" class="DigNum (strict)"() -> ("Minimum"=w2038:dbl)  [unwired: 2 in, 2 out]
            n1112 = property on="Z Scan Length SP steps" class="DigNum (strict)"("Val(Sgnl)"=w2102) -> ()  [unwired: 2 in, 2 out]
            n1113 = property on="Z Scan Velocity SP steps/sec" class="DigNum (strict)"() -> ("Minimum"=w2090:dbl)  [unwired: 2 in, 2 out]
            n1114 = Multiply(x=w2044, y=w2037) -> (x*y=w2041:dbl)
            n1115 = Multiply(x=w2096, y=w2089) -> (x*y=w2093:dbl)
            n1116 = In Range and Coerce(upper limit=w2039, x=w2041, lower limit=w2038) -> (coerced(x)=w2040:dbl)  [unwired: 1 out]
            n1117 = In Range and Coerce(upper limit=w2091, x=w2093, lower limit=w2090) -> (coerced(x)=w2092:dbl)  [unwired: 1 out]
            n1118 = To Long Integer(number=w2040) -> (32bit integer=w2042:i32)
            n1119 = To Long Integer(number=w2092) -> (32bit integer=w2094:i32)
            n1120 = property on="Y Scan Velocity SP steps/sec" class="DigNum (strict)"("Val(Sgnl)"=w2042) -> ()  [unwired: 2 in, 2 out]
            n1121 = property on="Z Scan Velocity SP steps/sec" class="DigNum (strict)"("Val(Sgnl)"=w2094) -> ()  [unwired: 2 in, 2 out]
            n1122 = property on="X mm/rev" class="DigNum (strict)"() -> ("Value"=w2071:dbl)  [unwired: 2 in, 2 out]
            n1123 = property on="X Scan Length SP mm" class="DigNum (strict)"() -> ("Value"=w2084:dbl)  [unwired: 2 in, 2 out]
            n1124 = property on="R deg/rev" class="DigNum (strict)"() -> ("Value"=w2054:dbl)  [unwired: 2 in, 2 out]
            n1125 = property on="R Scan Length SP deg" class="DigNum (strict)"() -> ("Value"=w2067:dbl)  [unwired: 2 in, 2 out]
            n1126 = Divide(x=w2067, y=w2054) -> (x/y=w2070:dbl)
            n1127 = Divide(x=w2084, y=w2071) -> (x/y=w2087:dbl)
            n1128 = property on="X steps/rev" class="DigNum (strict)"() -> ("Value"=w2086:u32)  [unwired: 2 in, 2 out]
            n1129 = property on="R steps/rev" class="DigNum (strict)"() -> ("Value"=w2069:u32)  [unwired: 2 in, 2 out]
            n1130 = To Double Precision Float(number=w2086) -> (double precision float=w2072:dbl)
            n1131 = To Double Precision Float(number=w2069) -> (double precision float=w2055:dbl)
            n1132 = property on="X Step SP" class="DigNum (strict)"() -> ("Minimum"=w2081:dbl)  [unwired: 2 in, 2 out]
            n1133 = property on="X Step SP" class="DigNum (strict)"() -> ("Maximum"=w2080:dbl)  [unwired: 2 in, 2 out]
            n1134 = Multiply(x=w2087, y=w2072) -> (x*y=w2083:dbl)
            n1135 = In Range and Coerce(upper limit=w2080, x=w2083, lower limit=w2081) -> (coerced(x)=w2082:dbl)  [unwired: 1 out]
            n1136 = property on="R Step SP" class="DigNum (strict)"() -> ("Maximum"=w2063:dbl)  [unwired: 2 in, 2 out]
            n1137 = property on="R Step SP" class="DigNum (strict)"() -> ("Minimum"=w2064:dbl)  [unwired: 2 in, 2 out]
            n1138 = Multiply(x=w2070, y=w2055) -> (x*y=w2066:dbl)
            n1139 = property on="X Scan Velocity SP mm/sec" class="DigNum (strict)"() -> ("Value"=w2078:dbl)  [unwired: 2 in, 2 out]
            n1140 = property on="R Scan Velocity SP deg/sec" class="DigNum (strict)"() -> ("Value"=w2061:dbl)  [unwired: 2 in, 2 out]
            n1141 = To Long Integer(number=w2082) -> (32bit integer=w2085:i32)
            n1142 = Divide(x=w2078, y=w2071) -> (x/y=w2079:dbl)
            n1143 = property on="X Scan Velocity SP steps/sec" class="DigNum (strict)"() -> ("Maximum"=w2074:dbl)  [unwired: 2 in, 2 out]
            n1144 = property on="X Scan Velocity SP steps/sec" class="DigNum (strict)"() -> ("Minimum"=w2073:dbl)  [unwired: 2 in, 2 out]
            n1145 = In Range and Coerce(upper limit=w2063, x=w2066, lower limit=w2064) -> (coerced(x)=w2065:dbl)  [unwired: 1 out]
            n1146 = Divide(x=w2061, y=w2054) -> (x/y=w2062:dbl)
            n1147 = property on="X Scan Length SP steps" class="DigNum (strict)"("Val(Sgnl)"=w2085) -> ()  [unwired: 2 in, 2 out]
            n1148 = Multiply(x=w2079, y=w2072) -> (x*y=w2076:dbl)
            n1149 = Multiply(x=w2062, y=w2055) -> (x*y=w2059:dbl)
            n1150 = To Long Integer(number=w2065) -> (32bit integer=w2068:i32)
            n1151 = property on="R Velocity SP step/sec" class="DigNum (strict)"() -> ("Maximum"=w2057:dbl)  [unwired: 2 in, 2 out]
            n1152 = property on="R Scan Velocity SP steps/sec" class="DigNum (strict)"() -> ("Minimum"=w2056:dbl)  [unwired: 2 in, 2 out]
            n1153 = Absolute Value(x=w2059) -> (abs(x)=w2053:dbl)
            n1154 = property on="R Scan Length SP steps" class="DigNum (strict)"("Val(Sgnl)"=w2068) -> ()  [unwired: 2 in, 2 out]
            n1155 = In Range and Coerce(upper limit=w2074, x=w2076, lower limit=w2073) -> (coerced(x)=w2075:dbl)  [unwired: 1 out]
            n1156 = In Range and Coerce(upper limit=w2057, x=w2053, lower limit=w2056) -> (coerced(x)=w2058:dbl)  [unwired: 1 out]
            n1157 = To Long Integer(number=w2075) -> (32bit integer=w2077:i32)
            n1158 = To Long Integer(number=w2058) -> (32bit integer=w2060:i32)
            n1159 = property on="X Scan Velocity SP steps/sec" class="DigNum (strict)"("Val(Sgnl)"=w2077) -> ()  [unwired: 2 in, 2 out]
            n1160 = property on="R Scan Velocity SP steps/sec" class="DigNum (strict)"("Val(Sgnl)"=w2060) -> ()  [unwired: 2 in, 2 out]
          }
          frame #1 {
            n1161 = case shown="True" "Z as dominating length" {
              frame #0 {
              }
              frame #1 {
                n1162 = property on="Y Scan Length SP steps" class="DigNum (strict)"() -> ("Value"=w2114:i32)  [unwired: 2 in, 2 out]
                n1163 = property on="Z Scan Length SP steps" class="DigNum (strict)"() -> ("Value"=w2113:i32)  [unwired: 2 in, 2 out]
                n1164 = property on="Y Scan Velocity SP steps/sec" class="DigNum (strict)"() -> ("Value"=w2110:i32)  [unwired: 2 in, 2 out]
                n1165 = property on="X Scan Length SP steps" class="DigNum (strict)"() -> ("Value"=w2122:i32)  [unwired: 2 in, 2 out]
                n1166 = property on="Z Scan Length SP steps" class="DigNum (strict)"() -> ("Value"=w2121:i32)  [unwired: 2 in, 2 out]
                n1167 = property on="X Scan Velocity SP steps/sec" class="DigNum (strict)"() -> ("Value"=w2120:i32)  [unwired: 2 in, 2 out]
                n1168 = To Double Precision Float(number=w2114) -> (double precision float=w2112:dbl)
                n1169 = To Double Precision Float(number=w2113) -> (double precision float=w2111:dbl)
                n1170 = To Double Precision Float(number=w2110) -> (double precision float=w2109:dbl)
                n1171 = To Double Precision Float(number=w2122) -> (double precision float=w2116:dbl)
                n1172 = To Double Precision Float(number=w2121) -> (double precision float=w2117:dbl)
                n1173 = To Double Precision Float(number=w2120) -> (double precision float=w2118:dbl)
                n1174 = Divide(x=w2112, y=w2111) -> (x/y=w2106:dbl)
                n1175 = Divide(x=w2116, y=w2117) -> (x/y=w2123:dbl)
                n1176 = Multiply(x=w2106, y=w2109) -> (x*y=w2108:dbl)
                n1177 = Multiply(x=w2123, y=w2118) -> (x*y=w2119:dbl)
                n1178 = To Long Integer(number=w2108) -> (32bit integer=w2107:i32)
                n1179 = To Long Integer(number=w2119) -> (32bit integer=w2115:i32)
                n1180 = property on="Y Scan Velocity SP steps/sec" class="DigNum (strict)"("Val(Sgnl)"=w2107) -> ()  [unwired: 2 in, 2 out]
                n1181 = property on="X Scan Velocity SP steps/sec" class="DigNum (strict)"("Val(Sgnl)"=w2115) -> ()  [unwired: 2 in, 2 out]
              }
            }
          }
        }
        n1182 = local write "STATUS"("SCANNING PARAMETERS SET" ("STATUS")) -> ()
      }
      event #12 {
        n1183 = event-data() -> ()  [unwired: 1 in, 7 out]
        n1184 = flat-sequence {
          tunnel: [w2273] -> w2171
          tunnel: [w2272] -> w2169
          tunnel: w2177 -> [w2275]
          tunnel: w2176 -> [w2274]
          tunnel: w2171 -> [w2281]
          tunnel: [w2281] -> w2170
          tunnel: w2169 -> [w2280]
          tunnel: [w2280] -> w2168
          tunnel: w2170 -> [w2285]
          tunnel: [w2284] -> w2173
          tunnel: w2168 -> [w2283]
          tunnel: [w2282] -> w2172
          tunnel: w2173 -> [w2293]
          tunnel: [w2293] -> w2175
          tunnel: w2172 -> [w2292]
          tunnel: [w2292] -> w2174
          tunnel: w2175 -> [w2298]
          tunnel: w2174 -> [w2297]
          tunnel: [w2298] -> w2179
          tunnel: [w2297] -> w2178
          tunnel: [w2300] -> w2180
          tunnel: [w2301] -> w2181
          tunnel: w2179 -> [w2301]
          tunnel: w2178 -> [w2300]
          frame #0 {
            n1185 = property on="X Scan Velocity SP steps/sec" class="DigNum (strict)"() -> ("Value"=w2277:i32)  [unwired: 2 in, 2 out]
            n1186 = Number To Decimal String(number=w2277) -> (decimal integer string=w2278:string)  [unwired: 1 in]
            n1187 = call "mDrive Send Command.vi"("error in (no error)"=w2275, "Extra"=w2278, "Command"=T10."Max Velocity", "VISA resource name"=w2274) -> ("error out"=w2272:errorcluster, "VISA resource name out"=w2273:refnum<visa-resource-name>)  [unwired: 3 in, 1 out]
          }
          frame #1 {
            n1188 = Wait (ms)(milliseconds to wait=u32 100) -> ()  [unwired: 1 out]
          }
          frame #2 {
            # "VELOCITY"
            n1189 = call "mDrive Send Command.vi"("error in (no error)"=w2283, "Extra"="VM", "Command"=T10."Print Parameter", "VISA resource name"=w2285) -> ("error out"=w2282:errorcluster, "read buffer"=w2288:string, "VISA resource name out"=w2284:refnum<visa-resource-name>)  [unwired: 3 in]
            n1190 = Decimal String To Number(string=w2288, offset=0) -> (number=w2286:i32)  [unwired: 1 in, 1 out]
            n1191 = property on="X velocity PV step/sec" class="DigNum (strict)"("Val(Sgnl)"=w2286) -> ()  [unwired: 2 in, 2 out]
          }
          frame #3 {
            n1192 = Wait (ms)(milliseconds to wait=u32 100) -> ()  [unwired: 1 out]
          }
          frame #4 {
            n1193 = property on="X Scan Velocity SP steps/sec" class="DigNum (strict)"("DisabledEnum"=T1."Disabled and Grayed Out" ("Disabled")) -> ()  [unwired: 2 in, 2 out]
            n1194 = property on="X Scan Length SP steps" class="DigNum (strict)"("DisabledEnum"=T1."Disabled and Grayed Out" ("Disabled")) -> ()  [unwired: 2 in, 2 out]
            n1195 = property on="Scan Go" class="Bool (strict)"("DisabledEnum"=T1."Enabled" ("Disabled")) -> ()  [unwired: 2 in, 2 out]
          }
          frame #5 {
            n1196 = property on="X Scan" class="Bool (strict)"("Val(Sgnl)"=TRUE ("Slew Ready 2")) -> ()  [unwired: 2 in, 2 out]
          }
        }
        n1197 = flat-sequence {
          tunnel: [w2215] -> w2153
          tunnel: [w2214] -> w2152
          tunnel: w2143 -> [w2213]
          tunnel: w2142 -> [w2212]
          tunnel: w2153 -> [w2221]
          tunnel: [w2221] -> w2151
          tunnel: w2152 -> [w2220]
          tunnel: [w2220] -> w2150
          tunnel: w2151 -> [w2227]
          tunnel: [w2226] -> w2149
          tunnel: w2150 -> [w2225]
          tunnel: [w2224] -> w2148
          tunnel: w2149 -> [w2233]
          tunnel: [w2233] -> w2147
          tunnel: w2148 -> [w2232]
          tunnel: [w2232] -> w2146
          tunnel: w2147 -> [w2238]
          tunnel: w2146 -> [w2237]
          tunnel: [w2238] -> w2145
          tunnel: [w2237] -> w2144
          tunnel: [w2240] -> w2140
          tunnel: [w2241] -> w2141
          tunnel: w2145 -> [w2241]
          tunnel: w2144 -> [w2240]
          frame #0 {
            n1198 = property on="Z Scan Velocity SP steps/sec" class="DigNum (strict)"() -> ("Value"=w2217:i32)  [unwired: 2 in, 2 out]
            n1199 = Number To Decimal String(number=w2217) -> (decimal integer string=w2218:string)  [unwired: 1 in]
            n1200 = call "mDrive Send Command.vi"("error in (no error)"=w2213, "Extra"=w2218, "Command"=T10."Max Velocity", "VISA resource name"=w2212) -> ("error out"=w2214:errorcluster, "VISA resource name out"=w2215:refnum<visa-resource-name>)  [unwired: 3 in, 1 out]
          }
          frame #1 {
            n1201 = Wait (ms)(milliseconds to wait=u32 100) -> ()  [unwired: 1 out]
          }
          frame #2 {
            # "VELOCITY"
            n1202 = call "mDrive Send Command.vi"("error in (no error)"=w2225, "Extra"="VM", "Command"=T10."Print Parameter", "VISA resource name"=w2227) -> ("error out"=w2224:errorcluster, "read buffer"=w2228:string, "VISA resource name out"=w2226:refnum<visa-resource-name>)  [unwired: 3 in]
            n1203 = Decimal String To Number(string=w2228, offset=0) -> (number=w2229:i32)  [unwired: 1 in, 1 out]
            n1204 = property on="Z  velocity PV step/sec" class="DigNum (strict)"("Val(Sgnl)"=w2229) -> ()  [unwired: 2 in, 2 out]
          }
          frame #3 {
            n1205 = Wait (ms)(milliseconds to wait=u32 100) -> ()  [unwired: 1 out]
          }
          frame #4 {
            n1206 = property on="Z Scan Length SP steps" class="DigNum (strict)"("DisabledEnum"=T1."Disabled and Grayed Out" ("Disabled")) -> ()  [unwired: 2 in, 2 out]
            n1207 = property on="Z Scan Velocity SP steps/sec" class="DigNum (strict)"("DisabledEnum"=T1."Disabled and Grayed Out" ("Disabled")) -> ()  [unwired: 2 in, 2 out]
            n1208 = property on="Scan Go" class="Bool (strict)"("DisabledEnum"=T1."Enabled" ("Disabled")) -> ()  [unwired: 2 in, 2 out]
          }
          frame #5 {
            n1209 = property on="Z Scan" class="Bool (strict)"("Val(Sgnl)"=TRUE ("Slew Ready 2")) -> ()  [unwired: 2 in, 2 out]
          }
        }
        n1210 = flat-sequence {
          tunnel: [w2245] -> w2167
          tunnel: [w2244] -> w2166
          tunnel: w2156 -> [w2243]
          tunnel: w2155 -> [w2242]
          tunnel: w2167 -> [w2251]
          tunnel: [w2251] -> w2165
          tunnel: w2166 -> [w2250]
          tunnel: [w2250] -> w2164
          tunnel: w2165 -> [w2255]
          tunnel: [w2254] -> w2163
          tunnel: w2164 -> [w2253]
          tunnel: [w2252] -> w2162
          tunnel: w2163 -> [w2263]
          tunnel: [w2263] -> w2161
          tunnel: w2162 -> [w2262]
          tunnel: [w2262] -> w2160
          tunnel: w2161 -> [w2268]
          tunnel: w2160 -> [w2267]
          tunnel: [w2268] -> w2159
          tunnel: [w2267] -> w2158
          tunnel: [w2270] -> w2157
          tunnel: [w2271] -> w2154
          tunnel: w2159 -> [w2271]
          tunnel: w2158 -> [w2270]
          frame #0 {
            n1211 = property on="Y Scan Velocity SP steps/sec" class="DigNum (strict)"() -> ("Value"=w2247:i32)  [unwired: 2 in, 2 out]
            n1212 = Number To Decimal String(number=w2247) -> (decimal integer string=w2248:string)  [unwired: 1 in]
            n1213 = call "mDrive Send Command.vi"("error in (no error)"=w2243, "Extra"=w2248, "Command"=T10."Max Velocity", "VISA resource name"=w2242) -> ("error out"=w2244:errorcluster, "VISA resource name out"=w2245:refnum<visa-resource-name>)  [unwired: 3 in, 1 out]
          }
          frame #1 {
            n1214 = Wait (ms)(milliseconds to wait=u32 100) -> ()  [unwired: 1 out]
          }
          frame #2 {
            # "VELOCITY"
            n1215 = call "mDrive Send Command.vi"("error in (no error)"=w2253, "Extra"="VM", "Command"=T10."Print Parameter", "VISA resource name"=w2255) -> ("error out"=w2252:errorcluster, "read buffer"=w2259:string, "VISA resource name out"=w2254:refnum<visa-resource-name>)  [unwired: 3 in]
            n1216 = Decimal String To Number(string=w2259, offset=0) -> (number=w2257:i32)  [unwired: 1 in, 1 out]
            n1217 = property on="Y velocity PV step/sec" class="DigNum (strict)"("Val(Sgnl)"=w2257) -> ()  [unwired: 2 in, 2 out]
          }
          frame #3 {
            n1218 = Wait (ms)(milliseconds to wait=u32 100) -> ()  [unwired: 1 out]
          }
          frame #4 {
            n1219 = property on="Y Scan Velocity SP steps/sec" class="DigNum (strict)"("DisabledEnum"=T1."Disabled and Grayed Out" ("Disabled")) -> ()  [unwired: 2 in, 2 out]
            n1220 = property on="Y Scan Length SP steps" class="DigNum (strict)"("DisabledEnum"=T1."Disabled and Grayed Out" ("Disabled")) -> ()  [unwired: 2 in, 2 out]
            n1221 = property on="Scan Go" class="Bool (strict)"("DisabledEnum"=T1."Enabled" ("Disabled")) -> ()  [unwired: 2 in, 2 out]
          }
          frame #5 {
            n1222 = property on="Y Scan" class="Bool (strict)"("Val(Sgnl)"=TRUE ("Slew Ready 2")) -> ()  [unwired: 2 in, 2 out]
          }
        }
        n1223 = flat-sequence {
          tunnel: [w2185] -> w2139
          tunnel: [w2184] -> w2138
          tunnel: w2129 -> [w2183]
          tunnel: w2128 -> [w2182]
          tunnel: w2139 -> [w2191]
          tunnel: [w2191] -> w2137
          tunnel: w2138 -> [w2190]
          tunnel: [w2190] -> w2136
          tunnel: w2137 -> [w2197]
          tunnel: [w2196] -> w2135
          tunnel: w2136 -> [w2195]
          tunnel: [w2194] -> w2134
          tunnel: w2135 -> [w2203]
          tunnel: w2134 -> [w2202]
          tunnel: [w2203] -> w2133
          tunnel: [w2202] -> w2132
          tunnel: w2133 -> [w2208]
          tunnel: w2132 -> [w2207]
          tunnel: [w2208] -> w2131
          tunnel: [w2207] -> w2130
          tunnel: [w2210] -> w2126
          tunnel: [w2211] -> w2127
          tunnel: w2131 -> [w2211]
          tunnel: w2130 -> [w2210]
          frame #0 {
            n1224 = property on="R Scan Velocity SP steps/sec" class="DigNum (strict)"() -> ("Value"=w2187:i32)  [unwired: 2 in, 2 out]
            n1225 = Number To Decimal String(number=w2187) -> (decimal integer string=w2188:string)  [unwired: 1 in]
            n1226 = call "mDrive Send Command.vi"("error in (no error)"=w2183, "Extra"=w2188, "Command"=T10."Max Velocity", "VISA resource name"=w2182) -> ("error out"=w2184:errorcluster, "VISA resource name out"=w2185:refnum<visa-resource-name>)  [unwired: 3 in, 1 out]
          }
          frame #1 {
            n1227 = Wait (ms)(milliseconds to wait=u32 100) -> ()  [unwired: 1 out]
          }
          frame #2 {
            # "VELOCITY"
            n1228 = call "mDrive Send Command.vi"("error in (no error)"=w2195, "Extra"="VM", "Command"=T10."Print Parameter", "VISA resource name"=w2197) -> ("error out"=w2194:errorcluster, "read buffer"=w2199:string, "VISA resource name out"=w2196:refnum<visa-resource-name>)  [unwired: 3 in]
            n1229 = Decimal String To Number(string=w2199, offset=0) -> (number=w2198:i32)  [unwired: 1 in, 1 out]
            n1230 = property on="R velocity PV step/sec" class="DigNum (strict)"("Val(Sgnl)"=w2198) -> ()  [unwired: 2 in, 2 out]
          }
          frame #3 {
            n1231 = Wait (ms)(milliseconds to wait=u32 100) -> ()  [unwired: 1 out]
          }
          frame #4 {
            n1232 = property on="R Scan Velocity SP steps/sec" class="DigNum (strict)"("DisabledEnum"=T1."Disabled and Grayed Out" ("Disabled")) -> ()  [unwired: 2 in, 2 out]
            n1233 = property on="R Scan Length SP steps" class="DigNum (strict)"("DisabledEnum"=T1."Disabled and Grayed Out" ("Disabled")) -> ()  [unwired: 2 in, 2 out]
            n1234 = property on="Scan Go" class="Bool (strict)"("DisabledEnum"=T1."Enabled" ("Disabled")) -> ()  [unwired: 2 in, 2 out]
          }
          frame #5 {
            n1235 = property on="R Scan" class="Bool (strict)"("Val(Sgnl)"=TRUE ("Slew Ready 2")) -> ()  [unwired: 2 in, 2 out]
          }
        }
        n1236 = property on="GO" class="Bool"("DisabledEnum"=T1."Disabled and Grayed Out" ("Disabled")) -> ()  [unwired: 2 in, 2 out]
        n1237 = local write "STATUS"("READY TO SCAN" ("STATUS")) -> ()
      }
      event #13 {
        n1238 = event-data() -> ()  [unwired: 1 in, 7 out]
        n1239 = flat-sequence {
          tunnel: [w2354] -> w2324
          tunnel: [w2353] -> w2323
          tunnel: w2312 -> [w2351]
          tunnel: w2310 -> [w2350]
          tunnel: [w2358] -> w2321
          tunnel: [w2359] -> w2322
          tunnel: w2324 -> [w2359]
          tunnel: w2323 -> [w2358]
          frame #0 {
            n1240 = call "mDrive Send Command.vi"("error in (no error)"=w2350, "Command"=T10."Stop", "VISA resource name"=w2351) -> ("error out"=w2353:errorcluster, "VISA resource name out"=w2354:refnum<visa-resource-name>)  [unwired: 4 in, 1 out]
          }
          frame #1 {
            n1241 = property on="X Scan" class="Bool (strict)"("Value"=FALSE ("Slew Ready")) -> ()  [unwired: 2 in, 2 out]
            n1242 = property on="X Scan Velocity SP steps/sec" class="DigNum (strict)"("DisabledEnum"=T1."Enabled" ("Disabled")) -> ()  [unwired: 2 in, 2 out]
            n1243 = property on="X Scan Length SP steps" class="DigNum (strict)"("DisabledEnum"=T1."Enabled" ("Disabled")) -> ()  [unwired: 2 in, 2 out]
          }
        }
        n1244 = flat-sequence {
          tunnel: [w2344] -> w2320
          tunnel: [w2343] -> w2319
          tunnel: w2311 -> [w2341]
          tunnel: w2309 -> [w2340]
          tunnel: [w2348] -> w2317
          tunnel: [w2349] -> w2318
          tunnel: w2320 -> [w2349]
          tunnel: w2319 -> [w2348]
          frame #0 {
            n1245 = call "mDrive Send Command.vi"("error in (no error)"=w2340, "Command"=T10."Stop", "VISA resource name"=w2341) -> ("error out"=w2343:errorcluster, "VISA resource name out"=w2344:refnum<visa-resource-name>)  [unwired: 4 in, 1 out]
          }
          frame #1 {
            n1246 = property on="Z Scan" class="Bool (strict)"("Value"=FALSE ("Slew Ready")) -> ()  [unwired: 2 in, 2 out]
            n1247 = property on="Z Scan Length SP steps" class="DigNum (strict)"("DisabledEnum"=T1."Enabled" ("Disabled")) -> ()  [unwired: 2 in, 2 out]
            n1248 = property on="Z Scan Velocity SP steps/sec" class="DigNum (strict)"("DisabledEnum"=T1."Enabled" ("Disabled")) -> ()  [unwired: 2 in, 2 out]
          }
        }
        n1249 = flat-sequence {
          tunnel: [w2364] -> w2326
          tunnel: [w2363] -> w2325
          tunnel: w2308 -> [w2361]
          tunnel: w2306 -> [w2360]
          tunnel: [w2368] -> w2328
          tunnel: [w2369] -> w2329
          tunnel: w2326 -> [w2369]
          tunnel: w2325 -> [w2368]
          frame #0 {
            n1250 = call "mDrive Send Command.vi"("error in (no error)"=w2360, "Command"=T10."Stop", "VISA resource name"=w2361) -> ("error out"=w2363:errorcluster, "VISA resource name out"=w2364:refnum<visa-resource-name>)  [unwired: 4 in, 1 out]
          }
          frame #1 {
            n1251 = property on="Y Scan" class="Bool (strict)"("Value"=FALSE ("Slew Ready")) -> ()  [unwired: 2 in, 2 out]
            n1252 = property on="Y Scan Velocity SP steps/sec" class="DigNum (strict)"("DisabledEnum"=T1."Enabled" ("Disabled")) -> ()  [unwired: 2 in, 2 out]
            n1253 = property on="Y Scan Length SP steps" class="DigNum (strict)"("DisabledEnum"=T1."Enabled" ("Disabled")) -> ()  [unwired: 2 in, 2 out]
          }
        }
        n1254 = flat-sequence {
          tunnel: [w2334] -> w2316
          tunnel: [w2333] -> w2315
          tunnel: w2307 -> [w2331]
          tunnel: w2305 -> [w2330]
          tunnel: [w2338] -> w2313
          tunnel: [w2339] -> w2314
          tunnel: w2316 -> [w2339]
          tunnel: w2315 -> [w2338]
          frame #0 {
            n1255 = call "mDrive Send Command.vi"("error in (no error)"=w2330, "Command"=T10."Stop", "VISA resource name"=w2331) -> ("error out"=w2333:errorcluster, "VISA resource name out"=w2334:refnum<visa-resource-name>)  [unwired: 4 in, 1 out]
          }
          frame #1 {
            n1256 = property on="R Scan" class="Bool (strict)"("Value"=FALSE ("Slew Ready")) -> ()  [unwired: 2 in, 2 out]
            n1257 = property on="R Scan Velocity SP steps/sec" class="DigNum (strict)"("DisabledEnum"=T1."Enabled" ("Disabled")) -> ()  [unwired: 2 in, 2 out]
            n1258 = property on="R Scan Length SP steps" class="DigNum (strict)"("DisabledEnum"=T1."Enabled" ("Disabled")) -> ()  [unwired: 2 in, 2 out]
          }
        }
        n1259 = property on="Set for Scan" class="Bool"("DisabledEnum"=T1."Enabled" ("Disabled")) -> ()  [unwired: 2 in, 2 out]
        n1260 = property on="Scan Go" class="Bool (strict)"("DisabledEnum"=T1."Disabled and Grayed Out" ("Disabled")) -> ()  [unwired: 2 in, 2 out]
        n1261 = property on="GO" class="Bool"("DisabledEnum"=T1."Enabled" ("Disabled")) -> ()  [unwired: 2 in, 2 out]
        n1262 = property on="Set Scan \nParameters" class="Bool"("DisabledEnum"=T1."Enabled" ("Disabled")) -> ()  [unwired: 2 in, 2 out]
      }
      event #14 {
        w2370 = T1."Disabled and Grayed Out" ("Disabled")
        n1263 = event-data() -> ()  [unwired: 1 in, 7 out]
        n1264 = flat-sequence {
          tunnel: [w2451] -> w2435
          tunnel: [w2449] -> w2428
          tunnel: [w2450] -> w2425
          tunnel: [w2444] -> w2424
          tunnel: [w2448] -> w2423
          tunnel: [w2447] -> w2422
          tunnel: [w2446] -> w2421
          tunnel: [w2445] -> w2420
          tunnel: w2387 -> [w2443]
          tunnel: w2386 -> [w2442]
          tunnel: w2385 -> [w2441]
          tunnel: w2384 -> [w2440]
          tunnel: w2383 -> [w2439]
          tunnel: w2382 -> [w2438]
          tunnel: w2381 -> [w2437]
          tunnel: w2380 -> [w2436]
          tunnel: [w2443] -> w2379
          tunnel: [w2442] -> w2378
          tunnel: [w2441] -> w2377
          tunnel: [w2440] -> w2376
          tunnel: [w2439] -> w2375
          tunnel: [w2438] -> w2374
          tunnel: [w2437] -> w2373
          tunnel: [w2436] -> w2372
          tunnel: [w2503] -> w2432
          tunnel: [w2502] -> w2430
          tunnel: w2435 -> [w2501]
          tunnel: w2428 -> [w2500]
          tunnel: [w2500] -> w2426
          tunnel: w2425 -> [w2499]
          tunnel: w2424 -> [w2488]
          tunnel: w2423 -> [w2498]
          tunnel: w2422 -> [w2494]
          tunnel: w2421 -> [w2491]
          tunnel: w2420 -> [w2497]
          tunnel: [w2496] -> w2418
          tunnel: [w2495] -> w2416
          tunnel: [w2494] -> w2413
          tunnel: [w2493] -> w2411
          tunnel: [w2492] -> w2409
          tunnel: [w2491] -> w2407
          tunnel: [w2490] -> w2405
          tunnel: [w2489] -> w2403
          tunnel: [w2488] -> w2402
          tunnel: w2379 -> [w2487]
          tunnel: w2378 -> [w2486]
          tunnel: w2377 -> [w2485]
          tunnel: w2376 -> [w2484]
          tunnel: w2375 -> [w2483]
          tunnel: w2374 -> [w2482]
          tunnel: w2373 -> [w2481]
          tunnel: w2372 -> [w2480]
          tunnel: w2432 -> [w2544]
          tunnel: [w2544] -> w2431
          tunnel: w2430 -> [w2543]
          tunnel: [w2543] -> w2429
          tunnel: [w2542] -> w2427
          tunnel: w2426 -> [w2542]
          tunnel: [w2541] -> w2419
          tunnel: w2418 -> [w2541]
          tunnel: [w2540] -> w2417
          tunnel: w2416 -> [w2540]
          tunnel: [w2539] -> w2415
          tunnel: [w2538] -> w2414
          tunnel: w2413 -> [w2538]
          tunnel: [w2537] -> w2412
          tunnel: w2411 -> [w2537]
          tunnel: [w2536] -> w2410
          tunnel: w2409 -> [w2536]
          tunnel: [w2535] -> w2408
          tunnel: w2407 -> [w2535]
          tunnel: [w2534] -> w2406
          tunnel: w2405 -> [w2534]
          tunnel: [w2533] -> w2404
          tunnel: w2403 -> [w2533]
          tunnel: w2402 -> [w2539]
          tunnel: w2431 -> [w2564]
          tunnel: [w2562] -> w2434
          tunnel: w2429 -> [w2563]
          tunnel: [w2561] -> w2433
          tunnel: w2427 -> [w2560]
          tunnel: w2419 -> [w2559]
          tunnel: w2417 -> [w2558]
          tunnel: w2415 -> [w2557]
          tunnel: w2414 -> [w2556]
          tunnel: w2412 -> [w2555]
          tunnel: w2410 -> [w2554]
          tunnel: w2408 -> [w2553]
          tunnel: w2406 -> [w2552]
          tunnel: w2404 -> [w2551]
          tunnel: [w2550] -> w2401
          tunnel: [w2549] -> w2400
          tunnel: [w2548] -> w2395
          tunnel: [w2547] -> w2392
          tunnel: [w2546] -> w2390
          tunnel: [w2545] -> w2388
          tunnel: w2434 -> [w2621]
          tunnel: w2433 -> [w2620]
          tunnel: [w2621] -> w2399
          tunnel: [w2620] -> w2398
          tunnel: [w2615] -> w2397
          tunnel: w2401 -> [w2615]
          tunnel: [w2614] -> w2396
          tunnel: w2400 -> [w2614]
          tunnel: w2395 -> [w2604]
          tunnel: [w2604] -> w2394
          tunnel: [w2603] -> w2393
          tunnel: w2392 -> [w2603]
          tunnel: [w2602] -> w2391
          tunnel: w2390 -> [w2602]
          tunnel: [w2601] -> w2389
          tunnel: w2388 -> [w2601]
          frame #0 {
            n1265 = property on="X Scan" class="Bool (strict)"() -> ("Value"=w2444:bool)  [unwired: 2 in, 2 out]
            n1266 = property on="Z Scan" class="Bool (strict)"() -> ("Value"=w2446:bool)  [unwired: 2 in, 2 out]
            n1267 = property on="Y Scan" class="Bool (strict)"() -> ("Value"=w2449:bool)  [unwired: 2 in, 2 out]
            n1268 = property on="R Scan" class="Bool (strict)"() -> ("Value"=w2447:bool)  [unwired: 2 in, 2 out]
            n1269 = case shown="False" w2449 {
              tunnel: ["" w2474] -> w2451
              frame #0 {
              }
              frame #1 {
                n1270 = property on="Y Scan Length SP steps" class="DigNum (strict)"() -> ("Value"=w2479:i32)  [unwired: 2 in, 2 out]
                n1271 = Number To Decimal String(number=w2479) -> (decimal integer string=w2476:string)  [unwired: 1 in]
                n1272 = call <vilib>:"Space Constant.vi"() -> ("String"=w2477:string)
                n1273 = Concatenate Strings("MR", w2477, w2476, "\r") -> (w2474:string)
              }
            }
            n1274 = case shown="False" w2444 {
              tunnel: ["" w2467] -> w2450
              frame #0 {
              }
              frame #1 {
                n1275 = property on="X Scan Length SP steps" class="DigNum (strict)"() -> ("Value"=w2472:i32)  [unwired: 2 in, 2 out]
                n1276 = Number To Decimal String(number=w2472) -> (decimal integer string=w2469:string)  [unwired: 1 in]
                n1277 = call <vilib>:"Space Constant.vi"() -> ("String"=w2470:string)
                n1278 = Concatenate Strings("MR", w2470, w2469, "\r") -> (w2467:string)
              }
            }
            n1279 = case shown="True" w2447 {
              tunnel: ["" w2453] -> w2445
              frame #0 {
              }
              frame #1 {
                n1280 = property on="R Scan Length SP steps" class="DigNum (strict)"() -> ("Value"=w2458:i32)  [unwired: 2 in, 2 out]
                n1281 = Number To Decimal String(number=w2458) -> (decimal integer string=w2455:string)  [unwired: 1 in]
                n1282 = call <vilib>:"Space Constant.vi"() -> ("String"=w2456:string)
                n1283 = Concatenate Strings("MR", w2456, w2455, "\r") -> (w2453:string)
              }
            }
            n1284 = case shown="False" w2446 {
              tunnel: ["" w2460] -> w2448
              frame #0 {
              }
              frame #1 {
                n1285 = property on="Z Scan Length SP steps" class="DigNum (strict)"() -> ("Value"=w2465:i32)  [unwired: 2 in, 2 out]
                n1286 = Number To Decimal String(number=w2465) -> (decimal integer string=w2462:string)  [unwired: 1 in]
                n1287 = call <vilib>:"Space Constant.vi"() -> ("String"=w2463:string)
                n1288 = Concatenate Strings("MR", w2463, w2462, "\r") -> (w2460:string)
              }
            }
          }
          frame #1 {
            n1289 = case shown="False" w2488 {
              tunnel: [w2519 w2524] -> w2496
              tunnel: [w2518 w2523] -> w2495
              tunnel: w2499 -> [_ w2522]
              tunnel: w2487 -> [w2519 w2521]
              tunnel: w2486 -> [w2518 w2520]
              frame #0 {
              }
              frame #1 {
                n1290 = VISA Write(VISA resource name=w2521, write buffer=w2522, error in (no error)=w2520) -> (VISA resource name out=w2524:refnum<visa-resource-name>, error out=w2523:errorcluster)  [unwired: 1 out]
              }
            }
            n1291 = case shown="True" w2491 {
              tunnel: [w2512 w2517] -> w2490
              tunnel: [w2511 w2516] -> w2489
              tunnel: w2498 -> [_ w2515]
              tunnel: w2485 -> [w2512 w2514]
              tunnel: w2484 -> [w2511 w2513]
              frame #0 {
              }
              frame #1 {
                n1292 = VISA Write(VISA resource name=w2514, write buffer=w2515, error in (no error)=w2513) -> (VISA resource name out=w2517:refnum<visa-resource-name>, error out=w2516:errorcluster)  [unwired: 1 out]
              }
            }
            n1293 = case shown="True" w2500 {
              tunnel: [w2526 w2531] -> w2503
              tunnel: [w2525 w2530] -> w2502
              tunnel: w2501 -> [_ w2529]
              tunnel: w2483 -> [w2526 w2528]
              tunnel: w2482 -> [w2525 w2527]
              frame #0 {
              }
              frame #1 {
                n1294 = VISA Write(VISA resource name=w2528, write buffer=w2529, error in (no error)=w2527) -> (VISA resource name out=w2531:refnum<visa-resource-name>, error out=w2530:errorcluster)  [unwired: 1 out]
              }
            }
            n1295 = case shown="True" w2494 {
              tunnel: [w2505 w2510] -> w2493
              tunnel: [w2504 w2509] -> w2492
              tunnel: w2497 -> [_ w2508]
              tunnel: w2481 -> [w2505 w2507]
              tunnel: w2480 -> [w2504 w2506]
              frame #0 {
              }
              frame #1 {
                n1296 = VISA Write(VISA resource name=w2507, write buffer=w2508, error in (no error)=w2506) -> (VISA resource name out=w2510:refnum<visa-resource-name>, error out=w2509:errorcluster)  [unwired: 1 out]
              }
            }
          }
          frame #2 {
            n1297 = Wait (ms)(milliseconds to wait=u32 100) -> ()  [unwired: 1 out]
          }
          frame #3 {
            n1298 = case shown="True" w2557 {
              tunnel: w2559 -> [w2584 w2588]
              tunnel: w2558 -> [w2583 w2587]
              tunnel: [w2584 w2586] -> w2546
              tunnel: [w2583 w2585] -> w2545
              frame #0 {
              }
              frame #1 {
                n1299 = property class="Instr"(reference=w2588, error in=w2587) -> (reference out=w2590:refnum<visa-resource-name>, error out=w2589:errorcluster, "Serial Settings:Number of Bytes at Serial Port"=w2591:u32)
                n1300 = VISA Read(VISA resource name=w2590, byte count=w2591, error in (no error)=w2589) -> (VISA resource name out=w2586:refnum<visa-resource-name>, error out=w2585:errorcluster)  [unwired: 2 out]
              }
            }
            n1301 = case shown="True" w2553 {
              tunnel: w2552 -> [w2566 w2570]
              tunnel: w2551 -> [w2565 w2569]
              tunnel: [w2566 w2568] -> w2550
              tunnel: [w2565 w2567] -> w2549
              frame #0 {
              }
              frame #1 {
                n1302 = property class="Instr"(reference=w2570, error in=w2569) -> (reference out=w2572:refnum<visa-resource-name>, error out=w2571:errorcluster, "Serial Settings:Number of Bytes at Serial Port"=w2573:u32)
                n1303 = VISA Read(VISA resource name=w2572, byte count=w2573, error in (no error)=w2571) -> (VISA resource name out=w2568:refnum<visa-resource-name>, error out=w2567:errorcluster)  [unwired: 2 out]
              }
            }
            n1304 = case shown="True" w2560 {
              tunnel: w2564 -> [w2593 w2597]
              tunnel: w2563 -> [w2592 w2596]
              tunnel: [w2593 w2595] -> w2562
              tunnel: [w2592 w2594] -> w2561
              frame #0 {
              }
              frame #1 {
                n1305 = property class="Instr"(reference=w2597, error in=w2596) -> (reference out=w2599:refnum<visa-resource-name>, error out=w2598:errorcluster, "Serial Settings:Number of Bytes at Serial Port"=w2600:u32)
                n1306 = VISA Read(VISA resource name=w2599, byte count=w2600, error in (no error)=w2598) -> (VISA resource name out=w2595:refnum<visa-resource-name>, error out=w2594:errorcluster)  [unwired: 2 out]
              }
            }
            n1307 = case shown="True" w2556 {
              tunnel: w2555 -> [w2575 w2579]
              tunnel: w2554 -> [w2574 w2578]
              tunnel: [w2575 w2577] -> w2548
              tunnel: [w2574 w2576] -> w2547
              frame #0 {
              }
              frame #1 {
                n1308 = property class="Instr"(reference=w2579, error in=w2578) -> (reference out=w2581:refnum<visa-resource-name>, error out=w2580:errorcluster, "Serial Settings:Number of Bytes at Serial Port"=w2582:u32)
                n1309 = VISA Read(VISA resource name=w2581, byte count=w2582, error in (no error)=w2580) -> (VISA resource name out=w2577:refnum<visa-resource-name>, error out=w2576:errorcluster)  [unwired: 2 out]
              }
            }
          }
          frame #4 {
            n1310 = property on="Y Scan" class="Bool (strict)"("Val(Sgnl)"=FALSE ("Slew Ready 2")) -> ()  [unwired: 2 in, 2 out]
            n1311 = property on="Z Scan" class="Bool (strict)"("Val(Sgnl)"=FALSE ("Slew Ready 2")) -> ()  [unwired: 2 in, 2 out]
            n1312 = property on="X Scan" class="Bool (strict)"("Val(Sgnl)"=FALSE ("Slew Ready 2")) -> ()  [unwired: 2 in, 2 out]
            n1313 = property on="R Scan" class="Bool (strict)"("Val(Sgnl)"=FALSE ("Slew Ready 2")) -> ()  [unwired: 2 in, 2 out]
            n1314 = property on="R Scan Length SP steps" class="DigNum (strict)"("DisabledEnum"=T1."Enabled" ("Disabled")) -> ()  [unwired: 2 in, 2 out]
            n1315 = property on="Y Scan Selocity SP steps/sec" class="DigNum (strict)"("DisabledEnum"=T1."Enabled" ("Disabled")) -> ()  [unwired: 2 in, 2 out]
            n1316 = property on="Scan Go" class="Bool (strict)"("DisabledEnum"=T1."Disabled and Grayed Out" ("Disabled")) -> ()  [unwired: 2 in, 2 out]
            n1317 = property on="Z Scan Velocity SP steps/sec" class="DigNum (strict)"("DisabledEnum"=T1."Enabled" ("Disabled")) -> ()  [unwired: 2 in, 2 out]
            n1318 = property on="X Scan Velocity SP steps/sec" class="DigNum (strict)"("DisabledEnum"=T1."Enabled" ("Disabled")) -> ()  [unwired: 2 in, 2 out]
            n1319 = property on="Y Scan Length SP steps" class="DigNum (strict)"("DisabledEnum"=T1."Enabled" ("Disabled")) -> ()  [unwired: 2 in, 2 out]
            n1320 = property on="R Scan Velocity SP steps/sec" class="DigNum (strict)"("DisabledEnum"=T1."Enabled" ("Disabled")) -> ()  [unwired: 2 in, 2 out]
            n1321 = property on="X Scan Length SP steps" class="DigNum (strict)"("DisabledEnum"=T1."Enabled" ("Disabled")) -> ()  [unwired: 2 in, 2 out]
            n1322 = property on="Z Scan Length SP steps" class="DigNum (strict)"("DisabledEnum"=T1."Enabled" ("Disabled")) -> ()  [unwired: 2 in, 2 out]
          }
        }
        n1323 = local write "STATUS"("SCANNING" ("STATUS")) -> ()
        n1324 = property on="GO" class="Bool"("DisabledEnum"=w2370) -> ()  [unwired: 2 in, 2 out]
        n1325 = property on="Set Scan \nParameters" class="Bool"("DisabledEnum"=w2370) -> ()  [unwired: 2 in, 2 out]
        n1326 = property on="Set for Scan" class="Bool"("DisabledEnum"=w2370) -> ()  [unwired: 2 in, 2 out]
      }
      event #15 {
        n1327 = event-data() -> ()  [unwired: 1 in, 7 out]
        n1328 = flat-sequence {
          tunnel: [w2661] -> w2637
          tunnel: [w2662] -> w2636
          tunnel: w2629 -> [w2660]
          tunnel: w2625 -> [w2659]
          frame #0 {
            n1329 = property on="Reset X Motor Steps" class="DigNum (strict)"() -> ("Value"=w2663:i32)  [unwired: 2 in, 2 out]
            n1330 = Number To Decimal String(number=w2663) -> (decimal integer string=w2664:string)  [unwired: 1 in]
            n1331 = call "mDrive Send Command.vi"("error in (no error)"=w2660, "Extra"=w2664, "Command"=T10."Set Current Position", "VISA resource name"=w2659) -> ("error out"=w2662:errorcluster, "VISA resource name out"=w2661:refnum<visa-resource-name>)  [unwired: 3 in, 1 out]
          }
        }
        n1332 = flat-sequence {
          tunnel: [w2655] -> w2635
          tunnel: [w2656] -> w2634
          tunnel: w2628 -> [w2653]
          tunnel: w2624 -> [w2652]
          frame #0 {
            n1333 = property on="Reset Z Motor Steps" class="DigNum (strict)"() -> ("Value"=w2654:i32)  [unwired: 2 in, 2 out]
            n1334 = Number To Decimal String(number=w2654) -> (decimal integer string=w2657:string)  [unwired: 1 in]
            n1335 = call "mDrive Send Command.vi"("error in (no error)"=w2653, "Extra"=w2657, "Command"=T10."Set Current Position", "VISA resource name"=w2652) -> ("error out"=w2656:errorcluster, "VISA resource name out"=w2655:refnum<visa-resource-name>)  [unwired: 3 in, 1 out]
          }
        }
        n1336 = flat-sequence {
          tunnel: [w2648] -> w2633
          tunnel: [w2649] -> w2632
          tunnel: w2627 -> [w2646]
          tunnel: w2623 -> [w2645]
          frame #0 {
            n1337 = property on="Reset Y Motor Steps" class="DigNum (strict)"() -> ("Value"=w2647:i32)  [unwired: 2 in, 2 out]
            n1338 = Number To Decimal String(number=w2647) -> (decimal integer string=w2650:string)  [unwired: 1 in]
            n1339 = call "mDrive Send Command.vi"("error in (no error)"=w2646, "Extra"=w2650, "Command"=T10."Set Current Position", "VISA resource name"=w2645) -> ("error out"=w2649:errorcluster, "VISA resource name out"=w2648:refnum<visa-resource-name>)  [unwired: 3 in, 1 out]
          }
        }
        n1340 = flat-sequence {
          tunnel: [w2641] -> w2631
          tunnel: [w2642] -> w2630
          tunnel: w2626 -> [w2639]
          tunnel: w2622 -> [w2638]
          frame #0 {
            n1341 = property on="Reset R Motor Steps" class="DigNum (strict)"() -> ("Value"=w2640:i32)  [unwired: 2 in, 2 out]
            n1342 = Number To Decimal String(number=w2640) -> (decimal integer string=w2643:string)  [unwired: 1 in]
            n1343 = call "mDrive Send Command.vi"("error in (no error)"=w2639, "Extra"=w2643, "Command"=T10."Set Current Position", "VISA resource name"=w2638) -> ("error out"=w2642:errorcluster, "VISA resource name out"=w2641:refnum<visa-resource-name>)  [unwired: 3 in, 1 out]
          }
        }
      }
    }
    n1344 = case shown="False" "Set Button" {
      tunnel: "Preset positions" -> [_ w314]
      frame #0 {
      }
      frame #1 {
        n1345 = local read "Presets"() -> (w315:i32[][])
        n1346 = Index Array(array=w315, index (row)=w314) -> (element=w313:i32[])  [unwired: 1 in]
        n1347 = Array To Cluster(array=w313) -> (cluster=w312:T11)
        n1348 = Unbundle(w312) -> ("Presets[0]"=w311:i32, "Presets[1]"=w310:i32, "Presets[2]"=w309:i32, "Presets[3]"=w308:i32)  [unwired: 5 out]
        n1349 = property on="X Step SP" class="DigNum (strict)"("Val(Sgnl)"=w311) -> ()  [unwired: 2 in, 2 out]
        n1350 = property on="Y Step SP" class="DigNum (strict)"("Val(Sgnl)"=w310) -> ()  [unwired: 2 in, 2 out]
        n1351 = property on="Z Step SP" class="DigNum (strict)"("Val(Sgnl)"=w309) -> ()  [unwired: 2 in, 2 out]
        n1352 = property on="R Step SP" class="DigNum (strict)"("Val(Sgnl)"=w308) -> ()  [unwired: 2 in, 2 out]
      }
    }
    n1353 = property on="Preset positions" class="Ring (strict)"() -> ("Strings []"=w259:string[])  [unwired: 2 in, 2 out]
    n1354 = case shown="False" "Add Button" {
      tunnel: w259 -> [_ w307]
      frame #0 {
      }
      frame #1 {
        n1355 = property on="X Step PV" class="DigNum (strict)"() -> ("Value"=w301:i32)  [unwired: 2 in, 2 out]
        n1356 = property on="Y Step PV" class="DigNum (strict)"() -> ("Value"=w300:i32)  [unwired: 2 in, 2 out]
        n1357 = property on="Z Step PV" class="DigNum (strict)"() -> ("Value"=w298:i32)  [unwired: 2 in, 2 out]
        n1358 = property on="R Step PV" class="DigNum (strict)"() -> ("Value"=w299:i32)  [unwired: 2 in, 2 out]
        n1359 = Build Array(w301, w300, w298, w299) -> (w304:i32[])
        n1360 = local read "Presets"() -> (w305:i32[][])
        n1361 = Build Array (concatenate)(w305, w304) -> (w303:i32[][])
        n1362 = Build Array (concatenate)(w307, "String") -> (w302:string[])
        n1363 = local write "Presets"(w303) -> ()
        n1364 = property on="Preset positions" class="Ring (strict)"("Strings []"=w302) -> ()  [unwired: 2 in, 2 out]
      }
    }
    n1365 = case shown="False" "Delete Button" {
      tunnel: w259 -> [_ w297]
      frame #0 {
      }
      frame #1 {
        n1366 = local read "Preset positions"() -> (w295:i32)
        n1367 = local read "Presets"() -> (w296:i32[][])
        n1368 = Delete From Array(array=w297, index=w295) -> (array with subset deleted=w293:string[])  [unwired: 1 in, 1 out]
        n1369 = Delete From Array(array=w296, index (row)=w295) -> (array with subset deleted=w294:i32[][])  [unwired: 2 in, 1 out]
        n1370 = property on="Preset positions" class="Ring (strict)"("Strings []"=w293) -> ()  [unwired: 2 in, 2 out]
        n1371 = local write "Presets"(w294) -> ()
      }
    }
    n1372 = case shown="False" "Stop" {
      selector: "Stop" -> [w324 w366]
      tunnel: [w324 w363] -> w266
      tunnel: w283 -> [w319 w354]
      tunnel: w282 -> [w318 w353]
      tunnel: w281 -> [w317 w355]
      tunnel: w280 -> [w320 w356]
      tunnel: w279 -> [w321 w357]
      tunnel: w278 -> [w322 w358]
      tunnel: w277 -> [w323 w360]
      tunnel: w276 -> [w316 w359]
      tunnel: [w323 w329] -> w275
      tunnel: [w322 w335] -> w274
      tunnel: [w321 w332] -> w273
      tunnel: [w320 w341] -> w272
      tunnel: [w319 w347] -> w271
      tunnel: [w318 w344] -> w270
      tunnel: [w317 w338] -> w269
      tunnel: [w316 w326] -> w268
      tunnel: w265 -> [_ w350]
      tunnel: w264 -> [_ w325]
      frame #0 {
      }
      frame #1 {
        n1373 = flat-sequence {
          tunnel: w366 -> [w432]
          tunnel: [w432] -> w365
          tunnel: [w431] -> w361
          tunnel: w360 -> [w425]
          tunnel: w359 -> [w424]
          tunnel: w358 -> [w423]
          tunnel: w357 -> [w422]
          tunnel: w356 -> [w421]
          tunnel: w355 -> [w418]
          tunnel: w354 -> [w420]
          tunnel: w353 -> [w419]
          tunnel: [w430] -> w351
          tunnel: w350 -> [w430]
          tunnel: [w377] -> w348
          tunnel: [w376] -> w345
          tunnel: [w386] -> w342
          tunnel: [w385] -> w339
          tunnel: [w396] -> w336
          tunnel: [w394] -> w333
          tunnel: [w405] -> w330
          tunnel: [w403] -> w327
          tunnel: w325 -> [w413]
          tunnel: w365 -> [w444]
          tunnel: [w444] -> w364
          tunnel: [w433] -> w362
          tunnel: w361 -> [w443]
          tunnel: [w442] -> w352
          tunnel: w351 -> [w442]
          tunnel: [w441] -> w349
          tunnel: w348 -> [w441]
          tunnel: [w440] -> w346
          tunnel: w345 -> [w440]
          tunnel: [w439] -> w343
          tunnel: w342 -> [w439]
          tunnel: [w438] -> w340
          tunnel: w339 -> [w438]
          tunnel: [w437] -> w337
          tunnel: w336 -> [w437]
          tunnel: [w436] -> w334
          tunnel: w333 -> [w436]
          tunnel: [w435] -> w331
          tunnel: w330 -> [w435]
          tunnel: [w434] -> w328
          tunnel: w327 -> [w434]
          tunnel: w364 -> [w456]
          tunnel: [w456] -> w363
          tunnel: w362 -> [w446]
          tunnel: w352 -> [w455]
          tunnel: w349 -> [w454]
          tunnel: [w454] -> w347
          tunnel: w346 -> [w453]
          tunnel: [w453] -> w344
          tunnel: w343 -> [w452]
          tunnel: [w452] -> w341
          tunnel: [w451] -> w338
          tunnel: w340 -> [w451]
          tunnel: [w450] -> w335
          tunnel: w337 -> [w450]
          tunnel: [w449] -> w332
          tunnel: w334 -> [w449]
          tunnel: [w448] -> w329
          tunnel: w331 -> [w448]
          tunnel: [w447] -> w326
          tunnel: w328 -> [w447]
          frame #0 {
            n1374 = local read "Presets"() -> (w412:i32[][])
            n1375 = call "mDrive Send Command.vi"("error in (no error)"=w424, "Command"=T10."Stop", "VISA resource name"=w425) -> ("error out"=w404:errorcluster, "VISA resource name out"=w406:refnum<visa-resource-name>)  [unwired: 4 in, 1 out]
            n1376 = call "mDrive Send Command.vi"("error in (no error)"=w422, "Command"=T10."Stop", "VISA resource name"=w423) -> ("error out"=w395:errorcluster, "VISA resource name out"=w397:refnum<visa-resource-name>)  [unwired: 4 in, 1 out]
            n1377 = call "mDrive Send Command.vi"("error in (no error)"=w418, "Command"=T10."Stop", "VISA resource name"=w421) -> ("error out"=w387:errorcluster, "VISA resource name out"=w388:refnum<visa-resource-name>)  [unwired: 4 in, 1 out]
            n1378 = call "mDrive Send Command.vi"("error in (no error)"=w419, "Command"=T10."Stop", "VISA resource name"=w420) -> ("error out"=w378:errorcluster, "VISA resource name out"=w379:refnum<visa-resource-name>)  [unwired: 4 in, 1 out]
            n1379 = property on="Preset positions" class="Ring (strict)"() -> ("Strings []"=w411:string[])  [unwired: 2 in, 2 out]
            n1380 = Number To Fractional String(number=w412) -> (F-format string=w414:string[][])  [unwired: 3 in]
            n1381 = property on="X  in Range" class="Bool (strict)"("Val(Sgnl)"=FALSE ("Value (Signaling)")) -> ()  [unwired: 2 in, 2 out]
            n1382 = property on="Y in Range" class="Bool (strict)"("Val(Sgnl)"=FALSE ("Value (Signaling)")) -> ()  [unwired: 2 in, 2 out]
            n1383 = property on="Z in Range" class="Bool (strict)"("Val(Sgnl)"=FALSE ("Value (Signaling)")) -> ()  [unwired: 2 in, 2 out]
            n1384 = property on="R in Range" class="Bool (strict)"("Val(Sgnl)"=FALSE ("Value (Signaling)")) -> ()  [unwired: 2 in, 2 out]
            n1385 = property on="X Ready" class="Bool (strict)"("Val(Sgnl)"=FALSE ("Value (Signaling)")) -> ()  [unwired: 2 in, 2 out]
            n1386 = property on="Y Ready" class="Bool (strict)"("Val(Sgnl)"=FALSE ("Value (Signaling)")) -> ()  [unwired: 2 in, 2 out]
            n1387 = property on="Z Ready" class="Bool (strict)"("Val(Sgnl)"=FALSE ("Value (Signaling)")) -> ()  [unwired: 2 in, 2 out]
            n1388 = property on="R Ready" class="Bool (strict)"("Val(Sgnl)"=FALSE ("Value (Signaling)")) -> ()  [unwired: 2 in, 2 out]
            n1389 = Transpose 2D Array(2D array=w414) -> (transposed array=w415:string[][])
            n1390 = Build Array (concatenate)(w411, w415) -> (w416:string[][])
            n1391 = call "mDrive Send Command.vi"("error in (no error)"=w395, "Extra"="P", "Command"=T10."Print Parameter", "VISA resource name"=w397) -> ("error out"=w394:errorcluster, "read buffer"=w401:string, "VISA resource name out"=w396:refnum<visa-resource-name>)  [unwired: 3 in]
            n1392 = call "mDrive Send Command.vi"("error in (no error)"=w387, "Extra"="P", "Command"=T10."Print Parameter", "VISA resource name"=w388) -> ("error out"=w385:errorcluster, "read buffer"=w392:string, "VISA resource name out"=w386:refnum<visa-resource-name>)  [unwired: 3 in]
            n1393 = call "mDrive Send Command.vi"("error in (no error)"=w404, "Extra"="P", "Command"=T10."Print Parameter", "VISA resource name"=w406) -> ("error out"=w403:errorcluster, "read buffer"=w410:string, "VISA resource name out"=w405:refnum<visa-resource-name>)  [unwired: 3 in]
            n1394 = call "mDrive Send Command.vi"("error in (no error)"=w378, "Extra"="P", "Command"=T10."Print Parameter", "VISA resource name"=w379) -> ("error out"=w376:errorcluster, "read buffer"=w383:string, "VISA resource name out"=w377:refnum<visa-resource-name>)  [unwired: 3 in]
            n1395 = Transpose 2D Array(2D array=w416) -> (transposed array=w417:string[][])
            n1396 = Decimal String To Number(string=w401, offset=0) -> (number=w393:i32)  [unwired: 1 in, 1 out]
            n1397 = Decimal String To Number(string=w392, offset=0) -> (number=w384:i32)  [unwired: 1 in, 1 out]
            n1398 = Decimal String To Number(string=w410, offset=0) -> (number=w402:i32)  [unwired: 1 in, 1 out]
            n1399 = Decimal String To Number(string=w383, offset=0) -> (number=w375:i32)  [unwired: 1 in, 1 out]
            n1400 = call-poly <vilib>:"Write To Spreadsheet File.vi"("2D data"=w417, "file path (dialog if empty)"=w413) -> ()  [unwired: 6 in, 1 out]
            n1401 = Build Array(w402, w384, w393, w375) -> (w431:i32[])
          }
          frame #1 {
            n1402 = To Double Precision Float(number=w443) -> (double precision float=w433:dbl[])
            n1403 = Wait (ms)(milliseconds to wait=u32 20) -> ()  [unwired: 1 out]
          }
          frame #2 {
            n1404 = call-poly <vilib>:"Write To Spreadsheet File.vi"("1D data"=w446, "file path (dialog if empty)"=w455) -> ()  [unwired: 6 in, 1 out]
          }
        }
      }
    }
  }
  n1405 = flat-sequence {
    tunnel: w48 -> [w2670]
    tunnel: w47 -> [w2667]
    frame #0 {
      n1406 = call "mDrive Send Command.vi"("error in (no error)"=w2667, "Command"=T10."Stop", "VISA resource name"=w2670) -> ("error out"=w2668:errorcluster, "VISA resource name out"=w2669:refnum<visa-resource-name>)  [unwired: 4 in, 1 out]
      n1407 = VISA Close(VISA resource name=w2669, error in (no error)=w2668) -> ()  [unwired: 1 out]
    }
  }
  n1408 = flat-sequence {
    tunnel: w42 -> [w2675]
    tunnel: w41 -> [w2672]
    frame #0 {
      n1409 = call "mDrive Send Command.vi"("error in (no error)"=w2672, "Command"=T10."Stop", "VISA resource name"=w2675) -> ("error out"=w2673:errorcluster, "VISA resource name out"=w2674:refnum<visa-resource-name>)  [unwired: 4 in, 1 out]
      n1410 = VISA Close(VISA resource name=w2674, error in (no error)=w2673) -> ()  [unwired: 1 out]
    }
  }
  n1411 = flat-sequence {
    tunnel: w40 -> [w2680]
    tunnel: w39 -> [w2677]
    frame #0 {
      n1412 = call "mDrive Send Command.vi"("error in (no error)"=w2677, "Command"=T10."Stop", "VISA resource name"=w2680) -> ("error out"=w2678:errorcluster, "VISA resource name out"=w2679:refnum<visa-resource-name>)  [unwired: 4 in, 1 out]
      n1413 = VISA Close(VISA resource name=w2679, error in (no error)=w2678) -> ()  [unwired: 1 out]
    }
  }
  n1414 = flat-sequence {
    tunnel: w38 -> [w2685]
    tunnel: w37 -> [w2682]
    frame #0 {
      n1415 = call "mDrive Send Command.vi"("error in (no error)"=w2682, "Command"=T10."Stop", "VISA resource name"=w2685) -> ("error out"=w2683:errorcluster, "VISA resource name out"=w2684:refnum<visa-resource-name>)  [unwired: 4 in, 1 out]
      n1416 = VISA Close(VISA resource name=w2684, error in (no error)=w2683) -> ()  [unwired: 1 out]
    }
  }
  "YCONSTArray" <- w36
  "XCONSTArray" <- w35
  "RCONSTArray" <- w34
  "ZCONSTArray" <- w33
  "RUNHOLDArray" <- w32
